vi "Condition _string_4_prod_count_YEAR_3.vi"(0 "Form Date":timestamp format="%<%Y-%m-%d>T", 1 "To Date":timestamp format="%<%Y-%m-%d>T", 3 "Shift":string(combo)="ALL", 4 "Select Station":string(combo)="ST 1", 5 "STACKHOLDER_ID":i32, 6 "Select Stakeholder":string(combo), 7 "Refnum out 2":T1, 9 "error in (no error)":errorcluster, 10 "Select Month":string(combo), 12 "Select Year":string(combo)) -> (11 "error out":errorcluster, 13 "Refnum out":T1, 14 "sum":i32[](array[numeric]), 15 "PROD COUNT TEST":string[](array[string]), 17 "Table":string[][](array[string]), 18 "Elements Found out":string[](array[string]), 19 "Array 3":string[][](array[string]))   [LabVIEW 2017]
uses:
  <vilib>/addons/database/Connection.llb/Conn ObjectReference.ctl
  <vilib>/addons/database/NI_Database_API.lvlib
panel:
  out "COUNT":string[](array[string])
  out "DATE":string[](array[string])
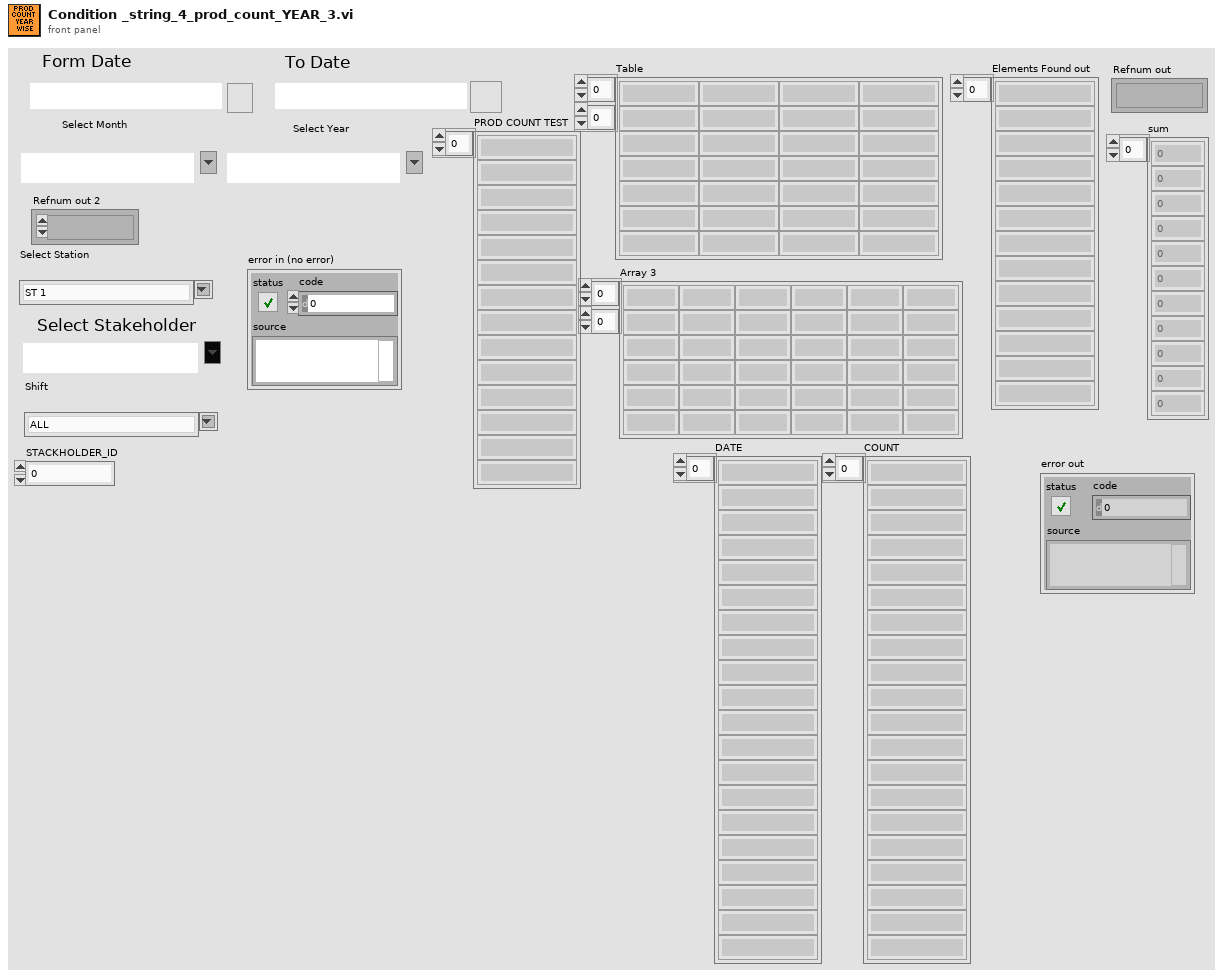
[diagram p1: front panel]
types:
  T1 = typedef "NI_Database_API.lvlib/Conn ObjectReference.ctl" = refnum<k1>
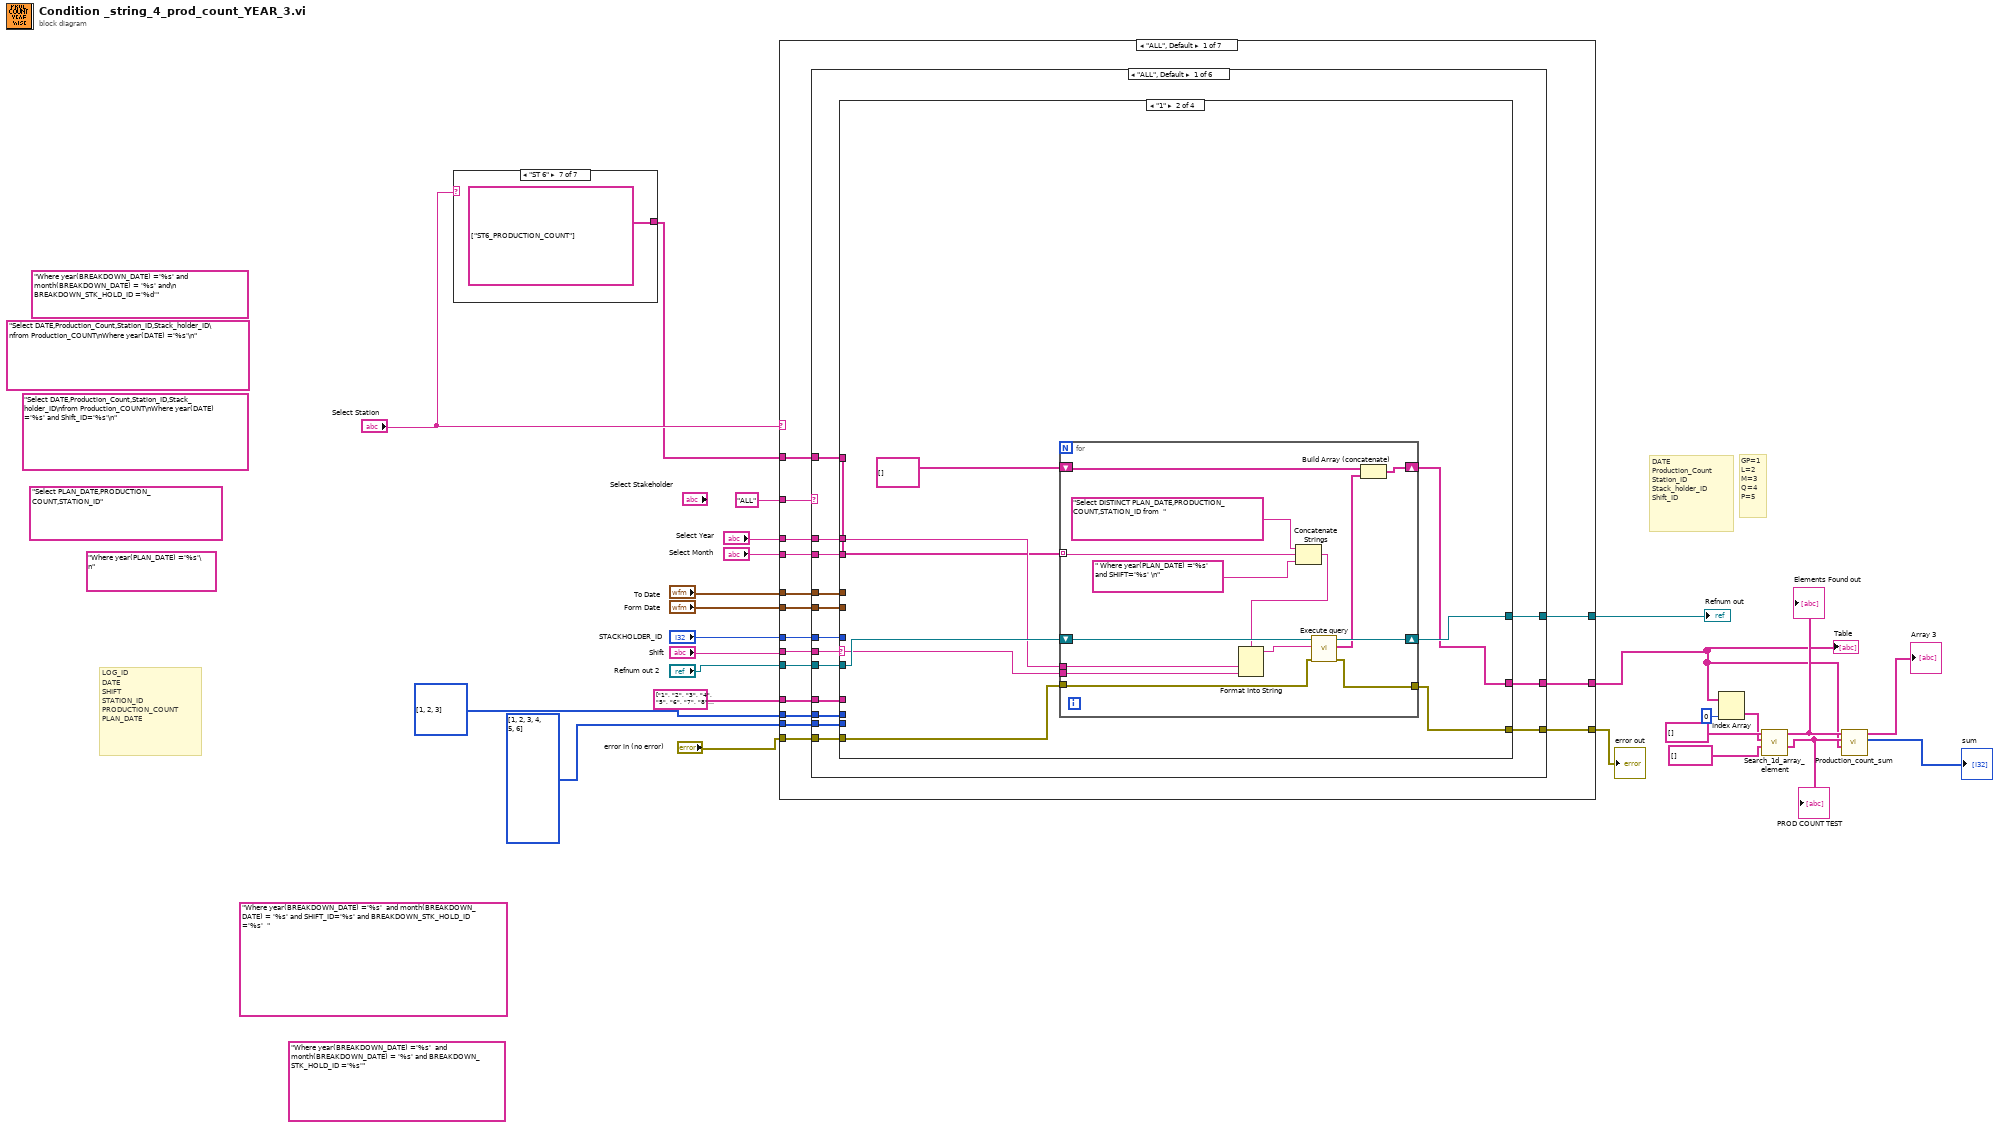
[diagram p0: block diagram]
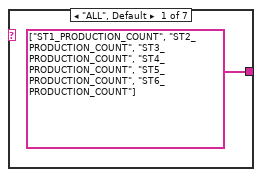
[diagram p2: hidden frame]
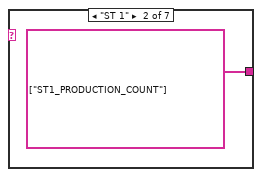
[diagram p3: hidden frame]
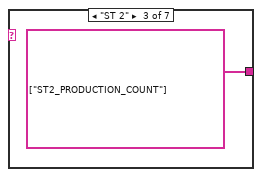
[diagram p4: hidden frame]
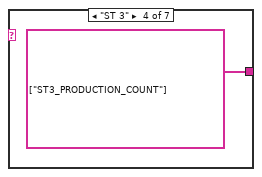
[diagram p5: hidden frame]
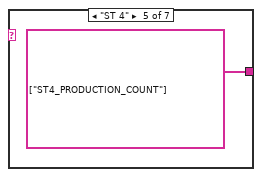
[diagram p6: hidden frame]
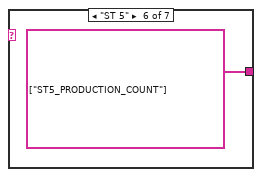
[diagram p7: hidden frame]
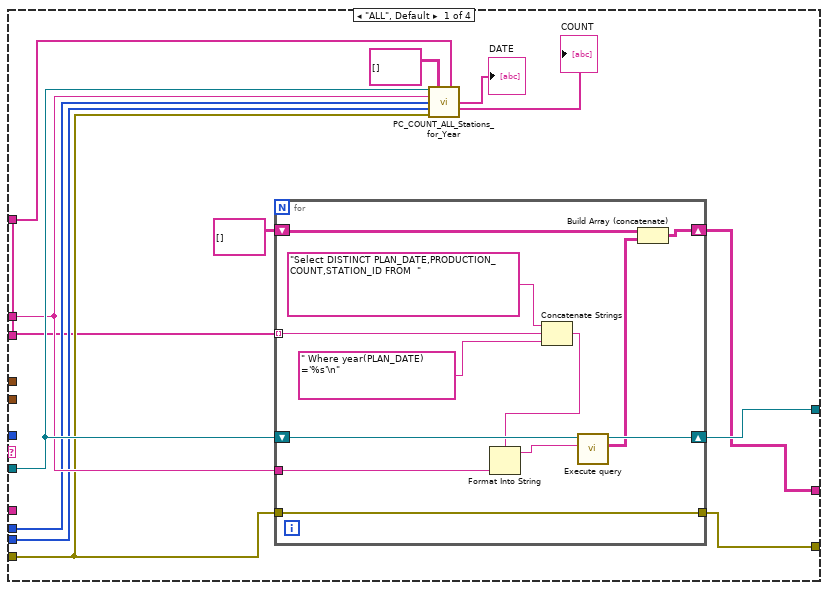
[diagram p8: hidden frame]
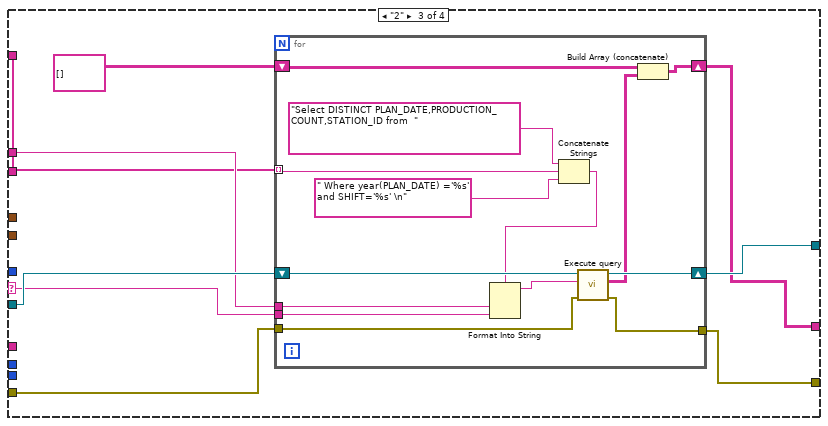
[diagram p9: hidden frame]
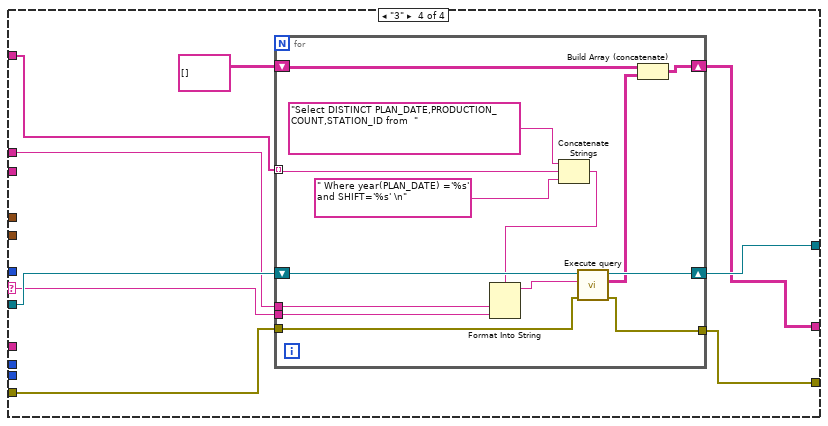
[diagram p10: hidden frame]
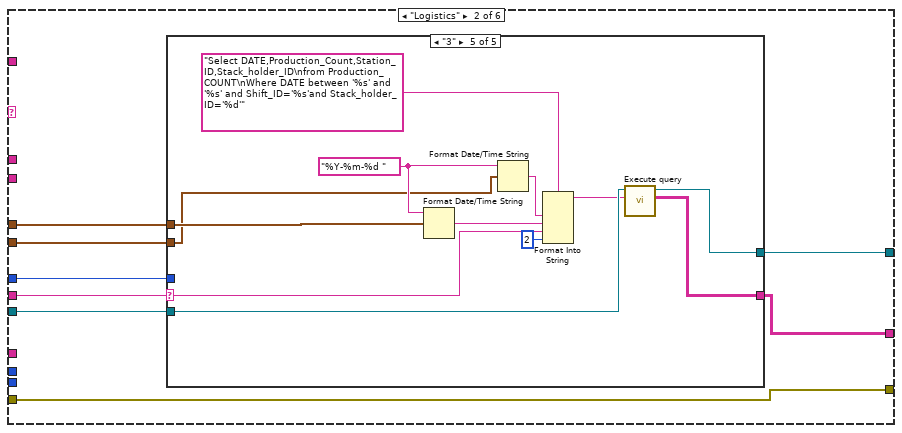
[diagram p11: hidden frame]
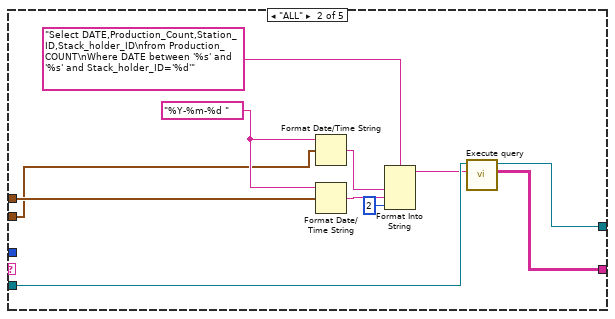
[diagram p13: hidden frame]
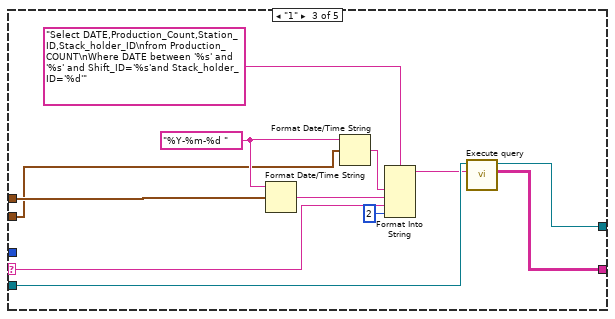
[diagram p14: hidden frame]
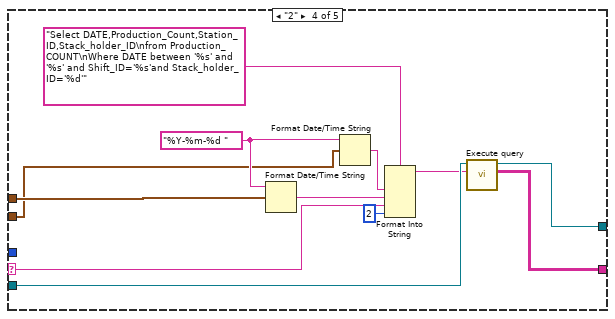
[diagram p15: hidden frame]
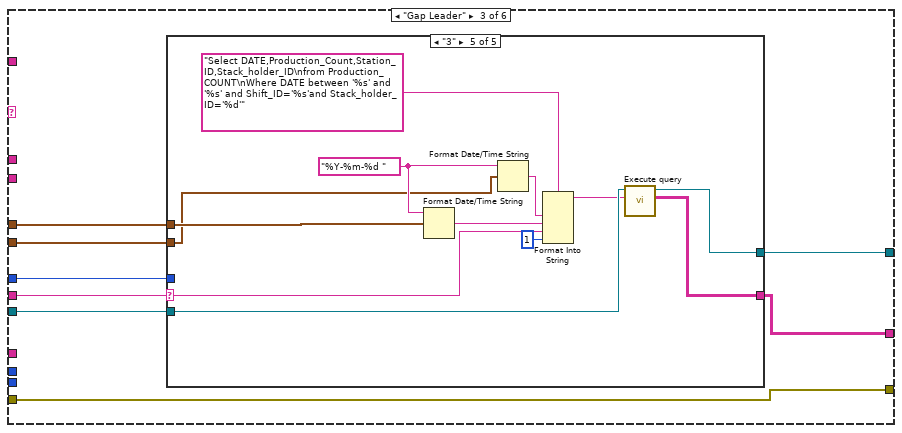
[diagram p16: hidden frame]
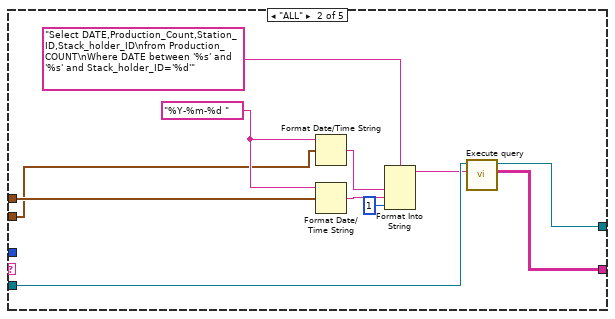
[diagram p18: hidden frame]
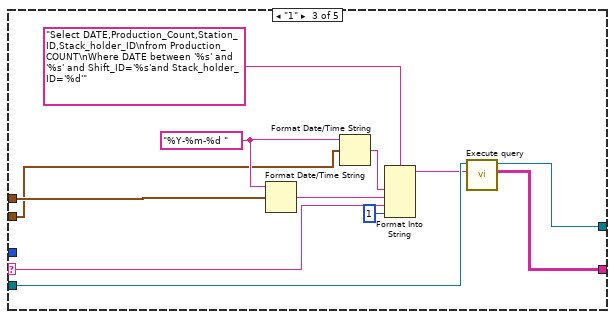
[diagram p19: hidden frame]
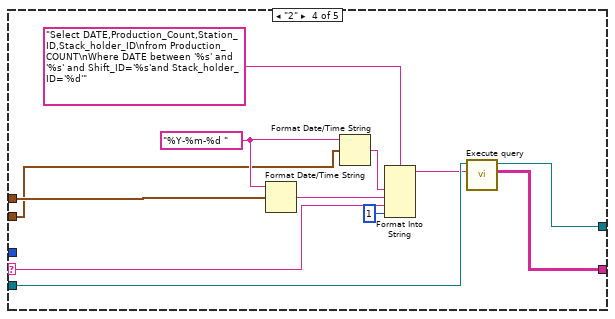
[diagram p20: hidden frame]
diagram:
  (unwired) "Where year(PLAN_DATE) ='%s'\n"
  (unwired) "Select PLAN_DATE,PRODUCTION_COUNT,STATION_ID"
  (unwired) "Select DATE,Production_Count,Station_ID,Stack_holder_ID\nfrom Production_COUNT\nWhere year(DATE) ='%s' and Shift_ID='%s'\n" ("string")
  (unwired) "Select DATE,Production_Count,Station_ID,Stack_holder_ID\nfrom Production_COUNT\nWhere year(DATE) ='%s'\n" ("string")
  (unwired) "Where year(BREAKDOWN_DATE) ='%s' and month(BREAKDOWN_DATE) = '%s' and\n BREAKDOWN_STK_HOLD_ID ='%d'" ("condition")
  (unwired) "Where year(BREAKDOWN_DATE) ='%s'  and month(BREAKDOWN_DATE) = '%s' and BREAKDOWN_STK_HOLD_ID ='%s'" ("condition")
  (unwired) "Where year(BREAKDOWN_DATE) ='%s'  and month(BREAKDOWN_DATE) = '%s' and SHIFT_ID='%s' and BREAKDOWN_STK_HOLD_ID ='%s'  " ("condition")
  # "LOG_ID\nDATE\nSHIFT\nSTATION_ID\nPRODUCTION_COUNT\nPLAN_DATE"
  # "GP=1\nL=2\nM=3\nQ=4\nP=5"
  # "DATE\nProduction_Count\nStation_ID\nStack_holder_ID\nShift_ID"
  n1 = case shown="\"ST 6\"" "Select Station" {
    tunnel: [string[] ["ST1_PRODUCTION_COUNT", "ST2_PRODUCTION_COUNT", "ST3_PRODUCTION_COUNT", "ST4_PRODUCTION_COUNT", "ST5_PRODUCTION_COUNT", "ST6_PRODUCTION_COUNT"] string[] ["ST1_PRODUCTION_COUNT"] string[] ["ST2_PRODUCTION_COUNT"] string[] ["ST3_PRODUCTION_COUNT"] string[] ["ST4_PRODUCTION_COUNT"] string[] ["ST5_PRODUCTION_COUNT"] string[] ["ST6_PRODUCTION_COUNT"]] -> w4
    frame "ALL", Default {
    }
    frame "ST 1" {
    }
    frame "ST 2" {
    }
    frame "ST 3" {
    }
    frame "ST 4" {
    }
    frame "ST 5" {
    }
    frame "ST 6" {
    }
  }
  n2 = case shown="\"ALL\", Default" "Select Station" {
    tunnel: "Shift" -> [w48 w450 w861 w1272 w1683 w2094 w2505]
    tunnel: "To Date" -> [w47 w449 w860 w1271 w1682 w2093 w2504]
    tunnel: "Form Date" -> [w46 w448 w859 w1270 w1681 w2092 w2503]
    tunnel: "STACKHOLDER_ID" -> [w45 w447 w858 w1269 w1680 w2091 w2502]
    tunnel: "Refnum out 2" -> [w44 w446 w857 w1268 w1679 w2090 w2501]
    tunnel: [w43 w445 w856 w1267 w1678 w2089 w2500] -> w20
    tunnel: "ALL" -> [w42 w444 w855 w1266 w1677 w2088 w2499]
    tunnel: i32[] [1, 2, 3, 4, 5, 6] -> [w41 _ _ _ _ _ _]
    tunnel: string[] ["1", "2", "3", "4", "5", "6", "7", "8", "9", "10", "11", "12"] -> [w40 _ _ _ _ _ _]
    tunnel: "Select Year" -> [w39 w443 w854 w1265 w1676 w2087 w2498]
    tunnel: "Select Month" -> [w38 w442 w853 w1264 w1675 w2086 w2497]
    tunnel: [w37 w441 w852 w1263 w1674 w2085 w2496] -> w7
    tunnel: w4 -> [w36 w440 w851 w1262 w1673 w2084 w2495]
    tunnel: "error in (no error)" -> [w35 w438 w849 w1260 w1671 w2082 w2493]
    tunnel: [w34 w439 w850 w1261 w1672 w2083 w2494] -> w2
    tunnel: i32[] [1, 2, 3] -> [w33 _ _ _ _ _ _]
    frame "ALL", Default {
      n3 = case shown="\"ALL\", Default" w42 {
        tunnel: w48 -> [w63 w165 w221 w277 w333 w389]
        tunnel: w47 -> [w62 w164 w220 w276 w332 w388]
        tunnel: w46 -> [w61 w163 w219 w275 w331 w387]
        tunnel: w45 -> [w60 w162 w218 w274 w330 w386]
        tunnel: w44 -> [w59 w161 w217 w273 w329 w385]
        tunnel: [w58 w160 w216 w272 w328 w384] -> w43
        tunnel: w41 -> [w57 _ _ _ _ _]
        tunnel: w40 -> [w56 _ _ _ _ _]
        tunnel: w39 -> [w55 _ _ _ _ _]
        tunnel: w38 -> [w54 _ _ _ _ _]
        tunnel: [w53 w158 w215 w270 w326 w382] -> w37
        tunnel: w36 -> [w52 _ _ _ _ _]
        tunnel: w35 -> [w51 w159 w214 w271 w327 w383]
        tunnel: [w50 w159 w214 w271 w327 w383] -> w34
        tunnel: w33 -> [w49 _ _ _ _ _]
        frame "ALL", Default {
          n4 = case shown="\"1\"" w63 {
            selector: w63 -> [_ w89 w112 w135]
            tunnel: w62 -> [_ _ _ _]
            tunnel: w61 -> [_ _ _ _]
            tunnel: w60 -> [_ _ _ _]
            tunnel: w59 -> [w72 w97 w120 w143]
            tunnel: [w76 w96 w119 w142] -> w58
            tunnel: w57 -> [w69 _ _ _]
            tunnel: w56 -> [_ _ _ _]
            tunnel: w55 -> [w71 w95 w118 w141]
            tunnel: w54 -> [_ _ _ _]
            tunnel: [w73 w90 w113 w136] -> w53
            tunnel: w52 -> [w66 w94 w117 w140]
            tunnel: w51 -> [w68 w92 w115 w138]
            tunnel: [w75 w93 w116 w139] -> w50
            tunnel: w49 -> [w70 _ _ _]
            frame "ALL", Default {
              n5 = for {
                tunnel: w71 -> [w86]
                shift-right: [w87] -> w76
                shift-left: w72 -> [w88]
                tunnel: w66 -> [w83] mode=indexing
                tunnel: [w80] -> w75
                tunnel: w68 -> [w80]
                shift-right: [w77] -> w73
                shift-left: string[][] [] ("Output Array") -> [w79]
                n6 = Concatenate Strings("Select DISTINCT PLAN_DATE,PRODUCTION_COUNT,STATION_ID FROM  ", w83, " Where year(PLAN_DATE) ='%s'\n") -> (w81:string)
                n7 = Format Into String(format string=w81, w86) -> (resulting string=w85:string)  [unwired: 2 in, 1 out]
                n8 = call "Execute query.vi"("String"=w85, "connection reference"=w88) -> ("Table"=w78:string[][], "connection reference 2"=w87:T1)  [unwired: 6 in, 2 out]
                n9 = Build Array (concatenate)(w79, w78) -> (w77:string[][])
              }
              n10 = call "PC_COUNT_ALL_Stations_for_Year.vi"("Refnum in"=w72, "data in"=string[][] [] ("Output Array"), "Array 3"=w66, "Select Year 2"=w71, "SHIFT"=w70, "STATION"=w69, "error in (no error)"=w68) -> ("DATE"=→"DATE":string[], "COUNT"=→"COUNT":string[])  [unwired: 4 in, 3 out]
            }
            frame "1" {
              n11 = for {
                tunnel: w95 -> [w109]
                shift-right: [w110] -> w96
                shift-left: w97 -> [w111]
                tunnel: w94 -> [w107] mode=indexing
                tunnel: [w100] -> w93
                tunnel: w92 -> [w101]
                shift-right: [w102] -> w90
                shift-left: string[][] [] ("Output Array") -> [w104]
                tunnel: w89 -> [w99]
                n12 = Concatenate Strings("Select DISTINCT PLAN_DATE,PRODUCTION_COUNT,STATION_ID from  ", w107, " Where year(PLAN_DATE) ='%s' and SHIFT='%s' \n") -> (w105:string)
                n13 = Format Into String(format string=w105, w109, w99) -> (resulting string=w108:string)  [unwired: 2 in, 1 out]
                n14 = call "Execute query.vi"("error in (no error)"=w101, "String"=w108, "connection reference"=w111) -> ("error out"=w100:errorcluster, "Table"=w103:string[][], "connection reference 2"=w110:T1)  [unwired: 5 in, 1 out]
                n15 = Build Array (concatenate)(w104, w103) -> (w102:string[][])
              }
            }
            frame "2" {
              n16 = for {
                tunnel: w118 -> [w132]
                shift-right: [w133] -> w119
                shift-left: w120 -> [w134]
                tunnel: w117 -> [w130] mode=indexing
                tunnel: [w123] -> w116
                tunnel: w115 -> [w124]
                shift-right: [w125] -> w113
                shift-left: string[][] [] ("Output Array") -> [w127]
                tunnel: w112 -> [w122]
                n17 = Concatenate Strings("Select DISTINCT PLAN_DATE,PRODUCTION_COUNT,STATION_ID from  ", w130, " Where year(PLAN_DATE) ='%s' and SHIFT='%s' \n") -> (w128:string)
                n18 = Format Into String(format string=w128, w132, w122) -> (resulting string=w131:string)  [unwired: 2 in, 1 out]
                n19 = call "Execute query.vi"("error in (no error)"=w124, "String"=w131, "connection reference"=w134) -> ("error out"=w123:errorcluster, "Table"=w126:string[][], "connection reference 2"=w133:T1)  [unwired: 5 in, 1 out]
                n20 = Build Array (concatenate)(w127, w126) -> (w125:string[][])
              }
            }
            frame "3" {
              n21 = for {
                tunnel: w141 -> [w155]
                shift-right: [w156] -> w142
                shift-left: w143 -> [w157]
                tunnel: w140 -> [w153] mode=indexing
                tunnel: [w146] -> w139
                tunnel: w138 -> [w147]
                shift-right: [w148] -> w136
                shift-left: string[][] [] ("Output Array") -> [w150]
                tunnel: w135 -> [w145]
                n22 = Concatenate Strings("Select DISTINCT PLAN_DATE,PRODUCTION_COUNT,STATION_ID from  ", w153, " Where year(PLAN_DATE) ='%s' and SHIFT='%s' \n") -> (w151:string)
                n23 = Format Into String(format string=w151, w155, w145) -> (resulting string=w154:string)  [unwired: 2 in, 1 out]
                n24 = call "Execute query.vi"("error in (no error)"=w147, "String"=w154, "connection reference"=w157) -> ("error out"=w146:errorcluster, "Table"=w149:string[][], "connection reference 2"=w156:T1)  [unwired: 5 in, 1 out]
                n25 = Build Array (concatenate)(w150, w149) -> (w148:string[][])
              }
            }
          }
        }
        frame "Logistics" {
          n26 = case shown="\"3\"" w165 {
            selector: w165 -> [_ _ w179 w191 w203]
            tunnel: w164 -> [_ w176 w188 w200 w212]
            tunnel: w163 -> [_ w175 w187 w199 w211]
            tunnel: w162 -> [_ _ _ _ _]
            tunnel: [_ w169 w181 w193 w205] -> w158
            tunnel: w161 -> [w166 w172 w184 w196 w208]
            tunnel: [w166 w168 w180 w192 w204] -> w160
            frame "False", Default {
            }
            frame "ALL" {
              w177 = "%Y-%m-%d " ("time format string (%c)")
              n27 = Format Date/Time String(time format string (%c)=w177, seconds (now)=w175) -> (date/time string=w174:string)  [unwired: 1 in]
              n28 = Format Date/Time String(time format string (%c)=w177, seconds (now)=w176) -> (date/time string=w173:string)  [unwired: 1 in]
              n29 = Format Into String(format string="Select DATE,Production_Count,Station_ID,Stack_holder_ID\nfrom Production_COUNT\nWhere DATE between '%s' and '%s' and Stack_holder_ID='%d'" ("string"), w174, w173, 2 ("input 3")) -> (resulting string=w170:string)  [unwired: 2 in, 1 out]
              n30 = call "Execute query.vi"("String"=w170, "connection reference"=w172) -> ("Table"=w169:string[][], "connection reference 2"=w168:T1)  [unwired: 6 in, 2 out]
            }
            frame "1" {
              w189 = "%Y-%m-%d " ("time format string (%c)")
              n31 = Format Date/Time String(time format string (%c)=w189, seconds (now)=w188) -> (date/time string=w185:string)  [unwired: 1 in]
              n32 = Format Date/Time String(time format string (%c)=w189, seconds (now)=w187) -> (date/time string=w186:string)  [unwired: 1 in]
              n33 = Format Into String(format string="Select DATE,Production_Count,Station_ID,Stack_holder_ID\nfrom Production_COUNT\nWhere DATE between '%s' and '%s' and Shift_ID='%s'and Stack_holder_ID='%d'" ("string"), w186, w185, w179, 2 ("input 4")) -> (resulting string=w182:string)  [unwired: 2 in, 1 out]
              n34 = call "Execute query.vi"("String"=w182, "connection reference"=w184) -> ("Table"=w181:string[][], "connection reference 2"=w180:T1)  [unwired: 6 in, 2 out]
            }
            frame "2" {
              w201 = "%Y-%m-%d " ("time format string (%c)")
              n35 = Format Date/Time String(time format string (%c)=w201, seconds (now)=w200) -> (date/time string=w197:string)  [unwired: 1 in]
              n36 = Format Date/Time String(time format string (%c)=w201, seconds (now)=w199) -> (date/time string=w198:string)  [unwired: 1 in]
              n37 = Format Into String(format string="Select DATE,Production_Count,Station_ID,Stack_holder_ID\nfrom Production_COUNT\nWhere DATE between '%s' and '%s' and Shift_ID='%s'and Stack_holder_ID='%d'" ("string"), w198, w197, w191, 2 ("input 4")) -> (resulting string=w194:string)  [unwired: 2 in, 1 out]
              n38 = call "Execute query.vi"("String"=w194, "connection reference"=w196) -> ("Table"=w193:string[][], "connection reference 2"=w192:T1)  [unwired: 6 in, 2 out]
            }
            frame "3" {
              w213 = "%Y-%m-%d " ("time format string (%c)")
              n39 = Format Date/Time String(time format string (%c)=w213, seconds (now)=w212) -> (date/time string=w209:string)  [unwired: 1 in]
              n40 = Format Date/Time String(time format string (%c)=w213, seconds (now)=w211) -> (date/time string=w210:string)  [unwired: 1 in]
              n41 = Format Into String(format string="Select DATE,Production_Count,Station_ID,Stack_holder_ID\nfrom Production_COUNT\nWhere DATE between '%s' and '%s' and Shift_ID='%s'and Stack_holder_ID='%d'" ("string"), w210, w209, w203, 2 ("input 4")) -> (resulting string=w206:string)  [unwired: 2 in, 1 out]
              n42 = call "Execute query.vi"("String"=w206, "connection reference"=w208) -> ("Table"=w205:string[][], "connection reference 2"=w204:T1)  [unwired: 6 in, 2 out]
            }
          }
        }
        frame "Gap Leader" {
          n43 = case shown="\"3\"" w221 {
            selector: w221 -> [_ _ w235 w247 w259]
            tunnel: w220 -> [_ w232 w244 w256 w268]
            tunnel: w219 -> [_ w231 w243 w255 w267]
            tunnel: w218 -> [_ _ _ _ _]
            tunnel: [_ w225 w237 w249 w261] -> w215
            tunnel: w217 -> [w222 w228 w240 w252 w264]
            tunnel: [w222 w224 w236 w248 w260] -> w216
            frame "False", Default {
            }
            frame "ALL" {
              w233 = "%Y-%m-%d " ("time format string (%c)")
              n44 = Format Date/Time String(time format string (%c)=w233, seconds (now)=w231) -> (date/time string=w230:string)  [unwired: 1 in]
              n45 = Format Date/Time String(time format string (%c)=w233, seconds (now)=w232) -> (date/time string=w229:string)  [unwired: 1 in]
              n46 = Format Into String(format string="Select DATE,Production_Count,Station_ID,Stack_holder_ID\nfrom Production_COUNT\nWhere DATE between '%s' and '%s' and Stack_holder_ID='%d'" ("string"), w230, w229, 1 ("input 3")) -> (resulting string=w226:string)  [unwired: 2 in, 1 out]
              n47 = call "Execute query.vi"("String"=w226, "connection reference"=w228) -> ("Table"=w225:string[][], "connection reference 2"=w224:T1)  [unwired: 6 in, 2 out]
            }
            frame "1" {
              w245 = "%Y-%m-%d " ("time format string (%c)")
              n48 = Format Date/Time String(time format string (%c)=w245, seconds (now)=w244) -> (date/time string=w241:string)  [unwired: 1 in]
              n49 = Format Date/Time String(time format string (%c)=w245, seconds (now)=w243) -> (date/time string=w242:string)  [unwired: 1 in]
              n50 = Format Into String(format string="Select DATE,Production_Count,Station_ID,Stack_holder_ID\nfrom Production_COUNT\nWhere DATE between '%s' and '%s' and Shift_ID='%s'and Stack_holder_ID='%d'" ("string"), w242, w241, w235, 1 ("input 4")) -> (resulting string=w238:string)  [unwired: 2 in, 1 out]
              n51 = call "Execute query.vi"("String"=w238, "connection reference"=w240) -> ("Table"=w237:string[][], "connection reference 2"=w236:T1)  [unwired: 6 in, 2 out]
            }
            frame "2" {
              w257 = "%Y-%m-%d " ("time format string (%c)")
              n52 = Format Date/Time String(time format string (%c)=w257, seconds (now)=w256) -> (date/time string=w253:string)  [unwired: 1 in]
              n53 = Format Date/Time String(time format string (%c)=w257, seconds (now)=w255) -> (date/time string=w254:string)  [unwired: 1 in]
              n54 = Format Into String(format string="Select DATE,Production_Count,Station_ID,Stack_holder_ID\nfrom Production_COUNT\nWhere DATE between '%s' and '%s' and Shift_ID='%s'and Stack_holder_ID='%d'" ("string"), w254, w253, w247, 1 ("input 4")) -> (resulting string=w250:string)  [unwired: 2 in, 1 out]
              n55 = call "Execute query.vi"("String"=w250, "connection reference"=w252) -> ("Table"=w249:string[][], "connection reference 2"=w248:T1)  [unwired: 6 in, 2 out]
            }
            frame "3" {
              w269 = "%Y-%m-%d " ("time format string (%c)")
              n56 = Format Date/Time String(time format string (%c)=w269, seconds (now)=w268) -> (date/time string=w265:string)  [unwired: 1 in]
              n57 = Format Date/Time String(time format string (%c)=w269, seconds (now)=w267) -> (date/time string=w266:string)  [unwired: 1 in]
              n58 = Format Into String(format string="Select DATE,Production_Count,Station_ID,Stack_holder_ID\nfrom Production_COUNT\nWhere DATE between '%s' and '%s' and Shift_ID='%s'and Stack_holder_ID='%d'" ("string"), w266, w265, w259, 1 ("input 4")) -> (resulting string=w262:string)  [unwired: 2 in, 1 out]
              n59 = call "Execute query.vi"("String"=w262, "connection reference"=w264) -> ("Table"=w261:string[][], "connection reference 2"=w260:T1)  [unwired: 6 in, 2 out]
            }
          }
        }
        frame "Maintenance" {
          n60 = case shown="\"ALL\"" w277 {
            selector: w277 -> [_ _ w291 w303 w315]
            tunnel: w276 -> [_ w288 w300 w312 w324]
            tunnel: w275 -> [_ w287 w299 w311 w323]
            tunnel: w274 -> [_ _ _ _ _]
            tunnel: [_ w281 w293 w305 w317] -> w270
            tunnel: w273 -> [w278 w284 w296 w308 w320]
            tunnel: [w278 w280 w292 w304 w316] -> w272
            frame "False", Default {
            }
            frame "ALL" {
              w289 = "%Y-%m-%d " ("time format string (%c)")
              n61 = Format Date/Time String(time format string (%c)=w289, seconds (now)=w287) -> (date/time string=w286:string)  [unwired: 1 in]
              n62 = Format Date/Time String(time format string (%c)=w289, seconds (now)=w288) -> (date/time string=w285:string)  [unwired: 1 in]
              n63 = Format Into String(format string="Select DATE,Production_Count,Station_ID,Stack_holder_ID\nfrom Production_COUNT\nWhere DATE between '%s' and '%s' and Stack_holder_ID='%d'" ("string"), w286, w285, 3 ("input 3")) -> (resulting string=w282:string)  [unwired: 2 in, 1 out]
              n64 = call "Execute query.vi"("String"=w282, "connection reference"=w284) -> ("Table"=w281:string[][], "connection reference 2"=w280:T1)  [unwired: 6 in, 2 out]
            }
            frame "1" {
              w301 = "%Y-%m-%d " ("time format string (%c)")
              n65 = Format Date/Time String(time format string (%c)=w301, seconds (now)=w300) -> (date/time string=w297:string)  [unwired: 1 in]
              n66 = Format Date/Time String(time format string (%c)=w301, seconds (now)=w299) -> (date/time string=w298:string)  [unwired: 1 in]
              n67 = Format Into String(format string="Select DATE,Production_Count,Station_ID,Stack_holder_ID\nfrom Production_COUNT\nWhere DATE between '%s' and '%s' and Shift_ID='%s'and Stack_holder_ID='%d'" ("string"), w298, w297, w291, 3 ("input 4")) -> (resulting string=w294:string)  [unwired: 2 in, 1 out]
              n68 = call "Execute query.vi"("String"=w294, "connection reference"=w296) -> ("Table"=w293:string[][], "connection reference 2"=w292:T1)  [unwired: 6 in, 2 out]
            }
            frame "2" {
              w313 = "%Y-%m-%d " ("time format string (%c)")
              n69 = Format Date/Time String(time format string (%c)=w313, seconds (now)=w312) -> (date/time string=w309:string)  [unwired: 1 in]
              n70 = Format Date/Time String(time format string (%c)=w313, seconds (now)=w311) -> (date/time string=w310:string)  [unwired: 1 in]
              n71 = Format Into String(format string="Select DATE,Production_Count,Station_ID,Stack_holder_ID\nfrom Production_COUNT\nWhere DATE between '%s' and '%s' and Shift_ID='%s'and Stack_holder_ID='%d'" ("string"), w310, w309, w303, 3 ("input 4")) -> (resulting string=w306:string)  [unwired: 2 in, 1 out]
              n72 = call "Execute query.vi"("String"=w306, "connection reference"=w308) -> ("Table"=w305:string[][], "connection reference 2"=w304:T1)  [unwired: 6 in, 2 out]
            }
            frame "3" {
              w325 = "%Y-%m-%d " ("time format string (%c)")
              n73 = Format Date/Time String(time format string (%c)=w325, seconds (now)=w324) -> (date/time string=w321:string)  [unwired: 1 in]
              n74 = Format Date/Time String(time format string (%c)=w325, seconds (now)=w323) -> (date/time string=w322:string)  [unwired: 1 in]
              n75 = Format Into String(format string="Select DATE,Production_Count,Station_ID,Stack_holder_ID\nfrom Production_COUNT\nWhere DATE between '%s' and '%s' and Shift_ID='%s'and Stack_holder_ID='%d'" ("string"), w322, w321, w315, 3 ("input 4")) -> (resulting string=w318:string)  [unwired: 2 in, 1 out]
              n76 = call "Execute query.vi"("String"=w318, "connection reference"=w320) -> ("Table"=w317:string[][], "connection reference 2"=w316:T1)  [unwired: 6 in, 2 out]
            }
          }
        }
        frame "Quality" {
          n77 = case shown="\"3\"" w333 {
            selector: w333 -> [_ _ w347 w359 w371]
            tunnel: w332 -> [_ w344 w356 w368 w380]
            tunnel: w331 -> [_ w343 w355 w367 w379]
            tunnel: w330 -> [_ _ _ _ _]
            tunnel: [_ w337 w349 w361 w373] -> w326
            tunnel: w329 -> [w334 w340 w352 w364 w376]
            tunnel: [w334 w336 w348 w360 w372] -> w328
            frame "False", Default {
            }
            frame "ALL" {
              w345 = "%Y-%m-%d " ("time format string (%c)")
              n78 = Format Date/Time String(time format string (%c)=w345, seconds (now)=w343) -> (date/time string=w342:string)  [unwired: 1 in]
              n79 = Format Date/Time String(time format string (%c)=w345, seconds (now)=w344) -> (date/time string=w341:string)  [unwired: 1 in]
              n80 = Format Into String(format string="Select DATE,Production_Count,Station_ID,Stack_holder_ID\nfrom Production_COUNT\nWhere DATE between '%s' and '%s' and Stack_holder_ID='%d'" ("string"), w342, w341, 4 ("input 3")) -> (resulting string=w338:string)  [unwired: 2 in, 1 out]
              n81 = call "Execute query.vi"("String"=w338, "connection reference"=w340) -> ("Table"=w337:string[][], "connection reference 2"=w336:T1)  [unwired: 6 in, 2 out]
            }
            frame "1" {
              w357 = "%Y-%m-%d " ("time format string (%c)")
              n82 = Format Date/Time String(time format string (%c)=w357, seconds (now)=w356) -> (date/time string=w353:string)  [unwired: 1 in]
              n83 = Format Date/Time String(time format string (%c)=w357, seconds (now)=w355) -> (date/time string=w354:string)  [unwired: 1 in]
              n84 = Format Into String(format string="Select DATE,Production_Count,Station_ID,Stack_holder_ID\nfrom Production_COUNT\nWhere DATE between '%s' and '%s' and Shift_ID='%s'and Stack_holder_ID='%d'" ("string"), w354, w353, w347, 4 ("input 4")) -> (resulting string=w350:string)  [unwired: 2 in, 1 out]
              n85 = call "Execute query.vi"("String"=w350, "connection reference"=w352) -> ("Table"=w349:string[][], "connection reference 2"=w348:T1)  [unwired: 6 in, 2 out]
            }
            frame "2" {
              w369 = "%Y-%m-%d " ("time format string (%c)")
              n86 = Format Date/Time String(time format string (%c)=w369, seconds (now)=w368) -> (date/time string=w365:string)  [unwired: 1 in]
              n87 = Format Date/Time String(time format string (%c)=w369, seconds (now)=w367) -> (date/time string=w366:string)  [unwired: 1 in]
              n88 = Format Into String(format string="Select DATE,Production_Count,Station_ID,Stack_holder_ID\nfrom Production_COUNT\nWhere DATE between '%s' and '%s' and Shift_ID='%s'and Stack_holder_ID='%d'" ("string"), w366, w365, w359, 4 ("input 4")) -> (resulting string=w362:string)  [unwired: 2 in, 1 out]
              n89 = call "Execute query.vi"("String"=w362, "connection reference"=w364) -> ("Table"=w361:string[][], "connection reference 2"=w360:T1)  [unwired: 6 in, 2 out]
            }
            frame "3" {
              w381 = "%Y-%m-%d " ("time format string (%c)")
              n90 = Format Date/Time String(time format string (%c)=w381, seconds (now)=w380) -> (date/time string=w377:string)  [unwired: 1 in]
              n91 = Format Date/Time String(time format string (%c)=w381, seconds (now)=w379) -> (date/time string=w378:string)  [unwired: 1 in]
              n92 = Format Into String(format string="Select DATE,Production_Count,Station_ID,Stack_holder_ID\nfrom Production_COUNT\nWhere DATE between '%s' and '%s' and Shift_ID='%s'and Stack_holder_ID='%d'" ("string"), w378, w377, w371, 4 ("input 4")) -> (resulting string=w374:string)  [unwired: 2 in, 1 out]
              n93 = call "Execute query.vi"("String"=w374, "connection reference"=w376) -> ("Table"=w373:string[][], "connection reference 2"=w372:T1)  [unwired: 6 in, 2 out]
            }
          }
        }
        frame "Production" {
          n94 = case shown="\"3\"" w389 {
            selector: w389 -> [_ _ w403 w415 w427]
            tunnel: w388 -> [_ w400 w412 w424 w436]
            tunnel: w387 -> [_ w399 w411 w423 w435]
            tunnel: w386 -> [_ _ _ _ _]
            tunnel: [_ w393 w405 w417 w429] -> w382
            tunnel: w385 -> [w390 w396 w408 w420 w432]
            tunnel: [w390 w392 w404 w416 w428] -> w384
            frame "False", Default {
            }
            frame "ALL" {
              w401 = "%Y-%m-%d " ("time format string (%c)")
              n95 = Format Date/Time String(time format string (%c)=w401, seconds (now)=w399) -> (date/time string=w398:string)  [unwired: 1 in]
              n96 = Format Date/Time String(time format string (%c)=w401, seconds (now)=w400) -> (date/time string=w397:string)  [unwired: 1 in]
              n97 = Format Into String(format string="Select DATE,Production_Count,Station_ID,Stack_holder_ID\nfrom Production_COUNT\nWhere DATE between '%s' and '%s' and Stack_holder_ID='%d'" ("string"), w398, w397, 5 ("input 3")) -> (resulting string=w394:string)  [unwired: 2 in, 1 out]
              n98 = call "Execute query.vi"("String"=w394, "connection reference"=w396) -> ("Table"=w393:string[][], "connection reference 2"=w392:T1)  [unwired: 6 in, 2 out]
            }
            frame "1" {
              w413 = "%Y-%m-%d " ("time format string (%c)")
              n99 = Format Date/Time String(time format string (%c)=w413, seconds (now)=w412) -> (date/time string=w409:string)  [unwired: 1 in]
              n100 = Format Date/Time String(time format string (%c)=w413, seconds (now)=w411) -> (date/time string=w410:string)  [unwired: 1 in]
              n101 = Format Into String(format string="Select DATE,Production_Count,Station_ID,Stack_holder_ID\nfrom Production_COUNT\nWhere DATE between '%s' and '%s' and Shift_ID='%s'and Stack_holder_ID='%d'" ("string"), w410, w409, w403, 5 ("input 4")) -> (resulting string=w406:string)  [unwired: 2 in, 1 out]
              n102 = call "Execute query.vi"("String"=w406, "connection reference"=w408) -> ("Table"=w405:string[][], "connection reference 2"=w404:T1)  [unwired: 6 in, 2 out]
            }
            frame "2" {
              w425 = "%Y-%m-%d " ("time format string (%c)")
              n103 = Format Date/Time String(time format string (%c)=w425, seconds (now)=w424) -> (date/time string=w421:string)  [unwired: 1 in]
              n104 = Format Date/Time String(time format string (%c)=w425, seconds (now)=w423) -> (date/time string=w422:string)  [unwired: 1 in]
              n105 = Format Into String(format string="Select DATE,Production_Count,Station_ID,Stack_holder_ID\nfrom Production_COUNT\nWhere DATE between '%s' and '%s' and Shift_ID='%s'and Stack_holder_ID='%d'" ("string"), w422, w421, w415, 5 ("input 4")) -> (resulting string=w418:string)  [unwired: 2 in, 1 out]
              n106 = call "Execute query.vi"("String"=w418, "connection reference"=w420) -> ("Table"=w417:string[][], "connection reference 2"=w416:T1)  [unwired: 6 in, 2 out]
            }
            frame "3" {
              w437 = "%Y-%m-%d " ("time format string (%c)")
              n107 = Format Date/Time String(time format string (%c)=w437, seconds (now)=w436) -> (date/time string=w433:string)  [unwired: 1 in]
              n108 = Format Date/Time String(time format string (%c)=w437, seconds (now)=w435) -> (date/time string=w434:string)  [unwired: 1 in]
              n109 = Format Into String(format string="Select DATE,Production_Count,Station_ID,Stack_holder_ID\nfrom Production_COUNT\nWhere DATE between '%s' and '%s' and Shift_ID='%s'and Stack_holder_ID='%d'" ("string"), w434, w433, w427, 5 ("input 4")) -> (resulting string=w430:string)  [unwired: 2 in, 1 out]
              n110 = call "Execute query.vi"("String"=w430, "connection reference"=w432) -> ("Table"=w429:string[][], "connection reference 2"=w428:T1)  [unwired: 6 in, 2 out]
            }
          }
        }
      }
    }
    frame "ST 1" {
      n111 = case shown="\"ALL\", Default" w444 {
        tunnel: w450 -> [w462 w563 w622 w678 w737 w796]
        tunnel: w449 -> [w461 w562 w621 w677 w736 w795]
        tunnel: w448 -> [w460 w561 w620 w676 w735 w794]
        tunnel: w447 -> [w459 w560 w619 w675 w734 w793]
        tunnel: [w458 w559 w618 w674 w733 w792] -> w441
        tunnel: w446 -> [w457 w558 w617 w673 w732 w791]
        tunnel: [w456 w557 w616 w672 w731 w790] -> w445
        tunnel: w443 -> [w455 _ _ _ _ _]
        tunnel: w442 -> [w454 _ _ _ _ _]
        tunnel: w440 -> [w453 _ _ _ _ _]
        tunnel: [w452 _ _ _ _ _] -> w439
        tunnel: w438 -> [w451 _ _ _ _ _]
        frame "ALL", Default {
          n112 = case shown="\"ALL\", Default" w462 {
            selector: w462 -> [_ w487 w511 w535]
            tunnel: w461 -> [_ _ _ _]
            tunnel: w460 -> [_ _ _ _]
            tunnel: w459 -> [_ _ _ _]
            tunnel: [w465 w488 w512 w536] -> w458
            tunnel: w457 -> [w470 w493 w517 w541]
            tunnel: [w469 w492 w516 w540] -> w456
            tunnel: w455 -> [w468 w491 w515 w539]
            tunnel: w454 -> [_ _ _ _]
            tunnel: w453 -> [w467 w490 w514 w538]
            tunnel: [w464 w486 w510 w534] -> w452
            tunnel: w451 -> [w463 w485 w509 w533]
            frame "ALL", Default {
              n113 = for {
                tunnel: w468 -> [w480]
                shift-right: [w482] -> w469
                shift-left: w470 -> [w484]
                tunnel: w467 -> [w476] mode=indexing
                shift-right: [w473] -> w465
                shift-left: string[][] [] -> [w475]
                tunnel: [w471] -> w464
                tunnel: w463 -> [w472]
                n114 = Concatenate Strings("Select DISTINCT PLAN_DATE,PRODUCTION_COUNT,STATION_ID from  ", w476, " Where year(PLAN_DATE) ='%s' and STATION_ID='%d'\n") -> (w477:string)
                n115 = Format Into String(format string=w477, w480, 1 ("input 3")) -> (resulting string=w483:string)  [unwired: 2 in, 1 out]
                n116 = call "Execute query.vi"("error in (no error)"=w472, "String"=w483, "connection reference"=w484) -> ("error out"=w471:errorcluster, "Table"=w474:string[][], "connection reference 2"=w482:T1)  [unwired: 5 in, 1 out]
                n117 = Build Array (concatenate)(w475, w474) -> (w473:string[][])
              }
            }
            frame "1" {
              n118 = for {
                tunnel: w491 -> [w504]
                shift-right: [w506] -> w492
                shift-left: w493 -> [w508]
                tunnel: w490 -> [w500] mode=indexing
                shift-right: [w497] -> w488
                shift-left: string[][] [] -> [w499]
                tunnel: w487 -> [w496]
                tunnel: [w494] -> w486
                tunnel: w485 -> [w495]
                n119 = Concatenate Strings("Select DISTINCT PLAN_DATE,PRODUCTION_COUNT,STATION_ID from  ", w500, " Where year(PLAN_DATE) ='%s' and STATION_ID='%d' and  SHIFT='%s'\n") -> (w501:string)
                n120 = Format Into String(format string=w501, w504, 1 ("input 3"), w496) -> (resulting string=w507:string)  [unwired: 2 in, 1 out]
                n121 = call "Execute query.vi"("error in (no error)"=w495, "String"=w507, "connection reference"=w508) -> ("error out"=w494:errorcluster, "Table"=w498:string[][], "connection reference 2"=w506:T1)  [unwired: 5 in, 1 out]
                n122 = Build Array (concatenate)(w499, w498) -> (w497:string[][])
              }
            }
            frame "2" {
              n123 = for {
                tunnel: w515 -> [w528]
                shift-right: [w530] -> w516
                shift-left: w517 -> [w532]
                tunnel: w514 -> [w524] mode=indexing
                shift-right: [w521] -> w512
                shift-left: string[][] [] -> [w523]
                tunnel: w511 -> [w520]
                tunnel: [w518] -> w510
                tunnel: w509 -> [w519]
                n124 = Concatenate Strings("Select DISTINCT PLAN_DATE,PRODUCTION_COUNT,STATION_ID from  ", w524, " Where year(PLAN_DATE) ='%s' and STATION_ID='%d' and SHIFT='%s'\n") -> (w525:string)
                n125 = Format Into String(format string=w525, w528, 1 ("input 3"), w520) -> (resulting string=w531:string)  [unwired: 2 in, 1 out]
                n126 = call "Execute query.vi"("error in (no error)"=w519, "String"=w531, "connection reference"=w532) -> ("error out"=w518:errorcluster, "Table"=w522:string[][], "connection reference 2"=w530:T1)  [unwired: 5 in, 1 out]
                n127 = Build Array (concatenate)(w523, w522) -> (w521:string[][])
              }
            }
            frame "3" {
              n128 = for {
                tunnel: w539 -> [w552]
                shift-right: [w554] -> w540
                shift-left: w541 -> [w556]
                tunnel: w538 -> [w548] mode=indexing
                shift-right: [w545] -> w536
                shift-left: string[][] [] -> [w547]
                tunnel: w535 -> [w544]
                tunnel: [w542] -> w534
                tunnel: w533 -> [w543]
                n129 = Concatenate Strings("Select DISTINCT PLAN_DATE,PRODUCTION_COUNT,STATION_ID from  ", w548, " Where year(PLAN_DATE) ='%s' and STATION_ID='%d' and  SHIFT='%s'\n") -> (w549:string)
                n130 = Format Into String(format string=w549, w552, 1 ("input 3"), w544) -> (resulting string=w555:string)  [unwired: 2 in, 1 out]
                n131 = call "Execute query.vi"("error in (no error)"=w543, "String"=w555, "connection reference"=w556) -> ("error out"=w542:errorcluster, "Table"=w546:string[][], "connection reference 2"=w554:T1)  [unwired: 5 in, 1 out]
                n132 = Build Array (concatenate)(w547, w546) -> (w545:string[][])
              }
            }
          }
        }
        frame "Logistics" {
          n133 = case shown="\"ALL\"" w563 {
            selector: w563 -> [_ _ w579 w592 w605]
            tunnel: w562 -> [_ w575 w588 w601 w614]
            tunnel: w561 -> [_ w574 w587 w600 w613]
            tunnel: w560 -> [_ _ _ _ _]
            tunnel: [_ w568 w581 w594 w607] -> w559
            tunnel: w558 -> [w564 w571 w584 w597 w610]
            tunnel: [w564 w567 w580 w593 w606] -> w557
            frame "False", Default {
            }
            frame "ALL" {
              w576 = "%Y-%m-%d " ("time format string (%c)")
              n134 = Format Date/Time String(time format string (%c)=w576, seconds (now)=w574) -> (date/time string=w573:string)  [unwired: 1 in]
              n135 = Format Date/Time String(time format string (%c)=w576, seconds (now)=w575) -> (date/time string=w572:string)  [unwired: 1 in]
              n136 = Format Into String(format string="Select DATE,Production_Count,Station_ID,Stack_holder_ID\nfrom Production_COUNT\nWhere DATE between '%s' and '%s' and Stack_holder_ID='%d'\nand Station_ID='%d'" ("string"), w573, w572, 2 ("input 3"), 1 ("input 4")) -> (resulting string=w569:string)  [unwired: 2 in, 1 out]
              n137 = call "Execute query.vi"("String"=w569, "connection reference"=w571) -> ("Table"=w568:string[][], "connection reference 2"=w567:T1)  [unwired: 6 in, 2 out]
            }
            frame "1" {
              w589 = "%Y-%m-%d " ("time format string (%c)")
              n138 = Format Date/Time String(time format string (%c)=w589, seconds (now)=w588) -> (date/time string=w585:string)  [unwired: 1 in]
              n139 = Format Date/Time String(time format string (%c)=w589, seconds (now)=w587) -> (date/time string=w586:string)  [unwired: 1 in]
              n140 = Format Into String(format string="Select DATE,Production_Count,Station_ID,Stack_holder_ID\nfrom Production_COUNT\nWhere DATE between '%s' and '%s' and Shift_ID='%s'and Stack_holder_ID='%d'\nand Station_ID='%d'" ("string"), w586, w585, w579, 2 ("input 4"), 1 ("input 4")) -> (resulting string=w582:string)  [unwired: 2 in, 1 out]
              n141 = call "Execute query.vi"("String"=w582, "connection reference"=w584) -> ("Table"=w581:string[][], "connection reference 2"=w580:T1)  [unwired: 6 in, 2 out]
            }
            frame "2" {
              w602 = "%Y-%m-%d " ("time format string (%c)")
              n142 = Format Date/Time String(time format string (%c)=w602, seconds (now)=w601) -> (date/time string=w598:string)  [unwired: 1 in]
              n143 = Format Date/Time String(time format string (%c)=w602, seconds (now)=w600) -> (date/time string=w599:string)  [unwired: 1 in]
              n144 = Format Into String(format string="Select DATE,Production_Count,Station_ID,Stack_holder_ID\nfrom Production_COUNT\nWhere DATE between '%s' and '%s' and Shift_ID='%s'and Stack_holder_ID='%d'\nand Station_ID='%d'" ("string"), w599, w598, w592, 2 ("input 4"), 1 ("input 4")) -> (resulting string=w595:string)  [unwired: 2 in, 1 out]
              n145 = call "Execute query.vi"("String"=w595, "connection reference"=w597) -> ("Table"=w594:string[][], "connection reference 2"=w593:T1)  [unwired: 6 in, 2 out]
            }
            frame "3" {
              w615 = "%Y-%m-%d " ("time format string (%c)")
              n146 = Format Date/Time String(time format string (%c)=w615, seconds (now)=w614) -> (date/time string=w611:string)  [unwired: 1 in]
              n147 = Format Date/Time String(time format string (%c)=w615, seconds (now)=w613) -> (date/time string=w612:string)  [unwired: 1 in]
              n148 = Format Into String(format string="Select DATE,Production_Count,Station_ID,Stack_holder_ID\nfrom Production_COUNT\nWhere DATE between '%s' and '%s' and Shift_ID='%s'and Stack_holder_ID='%d'\nand Station_ID='%d'" ("string"), w612, w611, w605, 2 ("input 4"), 1 ("input 4")) -> (resulting string=w608:string)  [unwired: 2 in, 1 out]
              n149 = call "Execute query.vi"("String"=w608, "connection reference"=w610) -> ("Table"=w607:string[][], "connection reference 2"=w606:T1)  [unwired: 6 in, 2 out]
            }
          }
        }
        frame "Gap Leader" {
          n150 = case shown="\"3\"" w622 {
            selector: w622 -> [_ _ w637 w649 w661]
            tunnel: w621 -> [_ w634 w646 w658 w670]
            tunnel: w620 -> [_ w633 w645 w657 w669]
            tunnel: w619 -> [_ _ _ _ _]
            tunnel: [_ w627 w639 w651 w663] -> w618
            tunnel: w617 -> [w623 w630 w642 w654 w666]
            tunnel: [w623 w626 w638 w650 w662] -> w616
            frame "False", Default {
            }
            frame "ALL" {
              w635 = "%Y-%m-%d " ("time format string (%c)")
              n151 = Format Date/Time String(time format string (%c)=w635, seconds (now)=w633) -> (date/time string=w632:string)  [unwired: 1 in]
              n152 = Format Date/Time String(time format string (%c)=w635, seconds (now)=w634) -> (date/time string=w631:string)  [unwired: 1 in]
              n153 = Format Into String(format string="Select DATE,Production_Count,Station_ID,Stack_holder_ID\nfrom Production_COUNT\nWhere DATE between '%s' and '%s' and Stack_holder_ID='%d'\nand Station_ID='%d'" ("string"), w632, w631, 1 ("input 3"), 1 ("input 3")) -> (resulting string=w628:string)  [unwired: 2 in, 1 out]
              n154 = call "Execute query.vi"("String"=w628, "connection reference"=w630) -> ("Table"=w627:string[][], "connection reference 2"=w626:T1)  [unwired: 6 in, 2 out]
            }
            frame "1" {
              w636 = 1 ("input 4")
              w647 = "%Y-%m-%d " ("time format string (%c)")
              n155 = Format Date/Time String(time format string (%c)=w647, seconds (now)=w646) -> (date/time string=w643:string)  [unwired: 1 in]
              n156 = Format Date/Time String(time format string (%c)=w647, seconds (now)=w645) -> (date/time string=w644:string)  [unwired: 1 in]
              n157 = Format Into String(format string="Select DATE,Production_Count,Station_ID,Stack_holder_ID\nfrom Production_COUNT\nWhere DATE between '%s' and '%s' and Shift_ID='%s'and Stack_holder_ID='%d'\nand Station_ID='%d'" ("string"), w644, w643, w637, w636, w636) -> (resulting string=w640:string)  [unwired: 2 in, 1 out]
              n158 = call "Execute query.vi"("String"=w640, "connection reference"=w642) -> ("Table"=w639:string[][], "connection reference 2"=w638:T1)  [unwired: 6 in, 2 out]
            }
            frame "2" {
              w648 = 1 ("input 4")
              w659 = "%Y-%m-%d " ("time format string (%c)")
              n159 = Format Date/Time String(time format string (%c)=w659, seconds (now)=w658) -> (date/time string=w655:string)  [unwired: 1 in]
              n160 = Format Date/Time String(time format string (%c)=w659, seconds (now)=w657) -> (date/time string=w656:string)  [unwired: 1 in]
              n161 = Format Into String(format string="Select DATE,Production_Count,Station_ID,Stack_holder_ID\nfrom Production_COUNT\nWhere DATE between '%s' and '%s' and Shift_ID='%s'and Stack_holder_ID='%d'\nand Station_ID='%d'" ("string"), w656, w655, w649, w648, w648) -> (resulting string=w652:string)  [unwired: 2 in, 1 out]
              n162 = call "Execute query.vi"("String"=w652, "connection reference"=w654) -> ("Table"=w651:string[][], "connection reference 2"=w650:T1)  [unwired: 6 in, 2 out]
            }
            frame "3" {
              w660 = 1 ("input 4")
              w671 = "%Y-%m-%d " ("time format string (%c)")
              n163 = Format Date/Time String(time format string (%c)=w671, seconds (now)=w670) -> (date/time string=w667:string)  [unwired: 1 in]
              n164 = Format Date/Time String(time format string (%c)=w671, seconds (now)=w669) -> (date/time string=w668:string)  [unwired: 1 in]
              n165 = Format Into String(format string="Select DATE,Production_Count,Station_ID,Stack_holder_ID\nfrom Production_COUNT\nWhere DATE between '%s' and '%s' and Shift_ID='%s'and Stack_holder_ID='%d'\nand Station_ID='%d'" ("string"), w668, w667, w661, w660, w660) -> (resulting string=w664:string)  [unwired: 2 in, 1 out]
              n166 = call "Execute query.vi"("String"=w664, "connection reference"=w666) -> ("Table"=w663:string[][], "connection reference 2"=w662:T1)  [unwired: 6 in, 2 out]
            }
          }
        }
        frame "Maintenance" {
          n167 = case shown="\"ALL\"" w678 {
            selector: w678 -> [_ _ w694 w707 w720]
            tunnel: w677 -> [_ w690 w703 w716 w729]
            tunnel: w676 -> [_ w689 w702 w715 w728]
            tunnel: w675 -> [_ _ _ _ _]
            tunnel: [_ w683 w696 w709 w722] -> w674
            tunnel: w673 -> [w679 w686 w699 w712 w725]
            tunnel: [w679 w682 w695 w708 w721] -> w672
            frame "False", Default {
            }
            frame "ALL" {
              w691 = "%Y-%m-%d " ("time format string (%c)")
              n168 = Format Date/Time String(time format string (%c)=w691, seconds (now)=w689) -> (date/time string=w688:string)  [unwired: 1 in]
              n169 = Format Date/Time String(time format string (%c)=w691, seconds (now)=w690) -> (date/time string=w687:string)  [unwired: 1 in]
              n170 = Format Into String(format string="Select DATE,Production_Count,Station_ID,Stack_holder_ID\nfrom Production_COUNT\nWhere DATE between '%s' and '%s' and Stack_holder_ID='%d'\nand Station_ID='%d'" ("string"), w688, w687, 3 ("input 3"), 1 ("input 4")) -> (resulting string=w684:string)  [unwired: 2 in, 1 out]
              n171 = call "Execute query.vi"("String"=w684, "connection reference"=w686) -> ("Table"=w683:string[][], "connection reference 2"=w682:T1)  [unwired: 6 in, 2 out]
            }
            frame "1" {
              w704 = "%Y-%m-%d " ("time format string (%c)")
              n172 = Format Date/Time String(time format string (%c)=w704, seconds (now)=w703) -> (date/time string=w700:string)  [unwired: 1 in]
              n173 = Format Date/Time String(time format string (%c)=w704, seconds (now)=w702) -> (date/time string=w701:string)  [unwired: 1 in]
              n174 = Format Into String(format string="Select DATE,Production_Count,Station_ID,Stack_holder_ID\nfrom Production_COUNT\nWhere DATE between '%s' and '%s' and Shift_ID='%s'and Stack_holder_ID='%d'\nand Station_ID='%d'" ("string"), w701, w700, w694, 3 ("input 4"), 1 ("input 5")) -> (resulting string=w697:string)  [unwired: 2 in, 1 out]
              n175 = call "Execute query.vi"("String"=w697, "connection reference"=w699) -> ("Table"=w696:string[][], "connection reference 2"=w695:T1)  [unwired: 6 in, 2 out]
            }
            frame "2" {
              w717 = "%Y-%m-%d " ("time format string (%c)")
              n176 = Format Date/Time String(time format string (%c)=w717, seconds (now)=w716) -> (date/time string=w713:string)  [unwired: 1 in]
              n177 = Format Date/Time String(time format string (%c)=w717, seconds (now)=w715) -> (date/time string=w714:string)  [unwired: 1 in]
              n178 = Format Into String(format string="Select DATE,Production_Count,Station_ID,Stack_holder_ID\nfrom Production_COUNT\nWhere DATE between '%s' and '%s' and Shift_ID='%s'and Stack_holder_ID='%d'\nand Station_ID='%d'" ("string"), w714, w713, w707, 3 ("input 4"), 1 ("input 5")) -> (resulting string=w710:string)  [unwired: 2 in, 1 out]
              n179 = call "Execute query.vi"("String"=w710, "connection reference"=w712) -> ("Table"=w709:string[][], "connection reference 2"=w708:T1)  [unwired: 6 in, 2 out]
            }
            frame "3" {
              w730 = "%Y-%m-%d " ("time format string (%c)")
              n180 = Format Date/Time String(time format string (%c)=w730, seconds (now)=w729) -> (date/time string=w726:string)  [unwired: 1 in]
              n181 = Format Date/Time String(time format string (%c)=w730, seconds (now)=w728) -> (date/time string=w727:string)  [unwired: 1 in]
              n182 = Format Into String(format string="Select DATE,Production_Count,Station_ID,Stack_holder_ID\nfrom Production_COUNT\nWhere DATE between '%s' and '%s' and Shift_ID='%s'and Stack_holder_ID='%d'\nand Station_ID='%d'" ("string"), w727, w726, w720, 3 ("input 4"), 1 ("input 5")) -> (resulting string=w723:string)  [unwired: 2 in, 1 out]
              n183 = call "Execute query.vi"("String"=w723, "connection reference"=w725) -> ("Table"=w722:string[][], "connection reference 2"=w721:T1)  [unwired: 6 in, 2 out]
            }
          }
        }
        frame "Quality" {
          n184 = case shown="\"ALL\"" w737 {
            selector: w737 -> [_ _ w753 w766 w779]
            tunnel: w736 -> [_ w749 w762 w775 w788]
            tunnel: w735 -> [_ w748 w761 w774 w787]
            tunnel: w734 -> [_ _ _ _ _]
            tunnel: [_ w742 w755 w768 w781] -> w733
            tunnel: w732 -> [w738 w745 w758 w771 w784]
            tunnel: [w738 w741 w754 w767 w780] -> w731
            frame "False", Default {
            }
            frame "ALL" {
              w750 = "%Y-%m-%d " ("time format string (%c)")
              n185 = Format Date/Time String(time format string (%c)=w750, seconds (now)=w748) -> (date/time string=w747:string)  [unwired: 1 in]
              n186 = Format Date/Time String(time format string (%c)=w750, seconds (now)=w749) -> (date/time string=w746:string)  [unwired: 1 in]
              n187 = Format Into String(format string="Select DATE,Production_Count,Station_ID,Stack_holder_ID\nfrom Production_COUNT\nWhere DATE between '%s' and '%s' and Stack_holder_ID='%d'\nand Station_ID='%d'" ("string"), w747, w746, 4 ("input 3"), 1 ("input 3")) -> (resulting string=w743:string)  [unwired: 2 in, 1 out]
              n188 = call "Execute query.vi"("String"=w743, "connection reference"=w745) -> ("Table"=w742:string[][], "connection reference 2"=w741:T1)  [unwired: 6 in, 2 out]
            }
            frame "1" {
              w763 = "%Y-%m-%d " ("time format string (%c)")
              n189 = Format Date/Time String(time format string (%c)=w763, seconds (now)=w762) -> (date/time string=w759:string)  [unwired: 1 in]
              n190 = Format Date/Time String(time format string (%c)=w763, seconds (now)=w761) -> (date/time string=w760:string)  [unwired: 1 in]
              n191 = Format Into String(format string="Select DATE,Production_Count,Station_ID,Stack_holder_ID\nfrom Production_COUNT\nWhere DATE between '%s' and '%s' and Shift_ID='%s'and Stack_holder_ID='%d'\nand Station_ID='%d'" ("string"), w760, w759, w753, 4 ("input 4"), 1 ("input 4")) -> (resulting string=w756:string)  [unwired: 2 in, 1 out]
              n192 = call "Execute query.vi"("String"=w756, "connection reference"=w758) -> ("Table"=w755:string[][], "connection reference 2"=w754:T1)  [unwired: 6 in, 2 out]
            }
            frame "2" {
              w776 = "%Y-%m-%d " ("time format string (%c)")
              n193 = Format Date/Time String(time format string (%c)=w776, seconds (now)=w775) -> (date/time string=w772:string)  [unwired: 1 in]
              n194 = Format Date/Time String(time format string (%c)=w776, seconds (now)=w774) -> (date/time string=w773:string)  [unwired: 1 in]
              n195 = Format Into String(format string="Select DATE,Production_Count,Station_ID,Stack_holder_ID\nfrom Production_COUNT\nWhere DATE between '%s' and '%s' and Shift_ID='%s'and Stack_holder_ID='%d'\nand Station_ID='%d'" ("string"), w773, w772, w766, 4 ("input 4"), 1 ("input 4")) -> (resulting string=w769:string)  [unwired: 2 in, 1 out]
              n196 = call "Execute query.vi"("String"=w769, "connection reference"=w771) -> ("Table"=w768:string[][], "connection reference 2"=w767:T1)  [unwired: 6 in, 2 out]
            }
            frame "3" {
              w789 = "%Y-%m-%d " ("time format string (%c)")
              n197 = Format Date/Time String(time format string (%c)=w789, seconds (now)=w788) -> (date/time string=w785:string)  [unwired: 1 in]
              n198 = Format Date/Time String(time format string (%c)=w789, seconds (now)=w787) -> (date/time string=w786:string)  [unwired: 1 in]
              n199 = Format Into String(format string="Select DATE,Production_Count,Station_ID,Stack_holder_ID\nfrom Production_COUNT\nWhere DATE between '%s' and '%s' and Shift_ID='%s'and Stack_holder_ID='%d'\nand Station_ID='%d'" ("string"), w786, w785, w779, 4 ("input 4"), 1 ("input 4")) -> (resulting string=w782:string)  [unwired: 2 in, 1 out]
              n200 = call "Execute query.vi"("String"=w782, "connection reference"=w784) -> ("Table"=w781:string[][], "connection reference 2"=w780:T1)  [unwired: 6 in, 2 out]
            }
          }
        }
        frame "Production" {
          n201 = case shown="\"ALL\"" w796 {
            selector: w796 -> [_ _ w812 w825 w838]
            tunnel: w795 -> [_ w808 w821 w834 w847]
            tunnel: w794 -> [_ w807 w820 w833 w846]
            tunnel: w793 -> [_ _ _ _ _]
            tunnel: [_ w801 w814 w827 w840] -> w792
            tunnel: w791 -> [w797 w804 w817 w830 w843]
            tunnel: [w797 w800 w813 w826 w839] -> w790
            frame "False", Default {
            }
            frame "ALL" {
              w809 = "%Y-%m-%d " ("time format string (%c)")
              n202 = Format Date/Time String(time format string (%c)=w809, seconds (now)=w807) -> (date/time string=w806:string)  [unwired: 1 in]
              n203 = Format Date/Time String(time format string (%c)=w809, seconds (now)=w808) -> (date/time string=w805:string)  [unwired: 1 in]
              n204 = Format Into String(format string="Select DATE,Production_Count,Station_ID,Stack_holder_ID\nfrom Production_COUNT\nWhere DATE between '%s' and '%s' and Stack_holder_ID='%d'\nand Station_ID='%d'" ("string"), w806, w805, 5 ("input 3"), 1 ("input 3")) -> (resulting string=w802:string)  [unwired: 2 in, 1 out]
              n205 = call "Execute query.vi"("String"=w802, "connection reference"=w804) -> ("Table"=w801:string[][], "connection reference 2"=w800:T1)  [unwired: 6 in, 2 out]
            }
            frame "1" {
              w822 = "%Y-%m-%d " ("time format string (%c)")
              n206 = Format Date/Time String(time format string (%c)=w822, seconds (now)=w821) -> (date/time string=w818:string)  [unwired: 1 in]
              n207 = Format Date/Time String(time format string (%c)=w822, seconds (now)=w820) -> (date/time string=w819:string)  [unwired: 1 in]
              n208 = Format Into String(format string="Select DATE,Production_Count,Station_ID,Stack_holder_ID\nfrom Production_COUNT\nWhere DATE between '%s' and '%s' and Shift_ID='%s'and Stack_holder_ID='%d'\nand Station_ID='%d'" ("string"), w819, w818, w812, 5 ("input 4"), 1 ("input 4")) -> (resulting string=w815:string)  [unwired: 2 in, 1 out]
              n209 = call "Execute query.vi"("String"=w815, "connection reference"=w817) -> ("Table"=w814:string[][], "connection reference 2"=w813:T1)  [unwired: 6 in, 2 out]
            }
            frame "2" {
              w835 = "%Y-%m-%d " ("time format string (%c)")
              n210 = Format Date/Time String(time format string (%c)=w835, seconds (now)=w834) -> (date/time string=w831:string)  [unwired: 1 in]
              n211 = Format Date/Time String(time format string (%c)=w835, seconds (now)=w833) -> (date/time string=w832:string)  [unwired: 1 in]
              n212 = Format Into String(format string="Select DATE,Production_Count,Station_ID,Stack_holder_ID\nfrom Production_COUNT\nWhere DATE between '%s' and '%s' and Shift_ID='%s'and Stack_holder_ID='%d'\nand Station_ID='%d'" ("string"), w832, w831, w825, 5 ("input 4"), 1 ("input 4")) -> (resulting string=w828:string)  [unwired: 2 in, 1 out]
              n213 = call "Execute query.vi"("String"=w828, "connection reference"=w830) -> ("Table"=w827:string[][], "connection reference 2"=w826:T1)  [unwired: 6 in, 2 out]
            }
            frame "3" {
              w848 = "%Y-%m-%d " ("time format string (%c)")
              n214 = Format Date/Time String(time format string (%c)=w848, seconds (now)=w847) -> (date/time string=w844:string)  [unwired: 1 in]
              n215 = Format Date/Time String(time format string (%c)=w848, seconds (now)=w846) -> (date/time string=w845:string)  [unwired: 1 in]
              n216 = Format Into String(format string="Select DATE,Production_Count,Station_ID,Stack_holder_ID\nfrom Production_COUNT\nWhere DATE between '%s' and '%s' and Shift_ID='%s'and Stack_holder_ID='%d'\nand Station_ID='%d'" ("string"), w845, w844, w838, 5 ("input 4"), 1 ("input 4")) -> (resulting string=w841:string)  [unwired: 2 in, 1 out]
              n217 = call "Execute query.vi"("String"=w841, "connection reference"=w843) -> ("Table"=w840:string[][], "connection reference 2"=w839:T1)  [unwired: 6 in, 2 out]
            }
          }
        }
      }
    }
    frame "ST 2" {
      n218 = case shown="\"ALL\", Default" w855 {
        tunnel: w861 -> [w873 w974 w1033 w1089 w1148 w1207]
        tunnel: w860 -> [w872 w973 w1032 w1088 w1147 w1206]
        tunnel: w859 -> [w871 w972 w1031 w1087 w1146 w1205]
        tunnel: w858 -> [w870 w971 w1030 w1086 w1145 w1204]
        tunnel: [w869 w970 w1029 w1085 w1144 w1203] -> w852
        tunnel: w857 -> [w868 w969 w1028 w1084 w1143 w1202]
        tunnel: [w867 w968 w1027 w1083 w1142 w1201] -> w856
        tunnel: w854 -> [w866 _ _ _ _ _]
        tunnel: w853 -> [w865 _ _ _ _ _]
        tunnel: w851 -> [w864 _ _ _ _ _]
        tunnel: [w863 _ _ _ _ _] -> w850
        tunnel: w849 -> [w862 _ _ _ _ _]
        frame "ALL", Default {
          n219 = case shown="\"ALL\", Default" w873 {
            selector: w873 -> [_ w898 w922 w946]
            tunnel: w872 -> [_ _ _ _]
            tunnel: w871 -> [_ _ _ _]
            tunnel: w870 -> [_ _ _ _]
            tunnel: [w876 w899 w923 w947] -> w869
            tunnel: w868 -> [w881 w904 w928 w952]
            tunnel: [w880 w903 w927 w951] -> w867
            tunnel: w866 -> [w879 w902 w926 w950]
            tunnel: w865 -> [_ _ _ _]
            tunnel: w864 -> [w878 w901 w925 w949]
            tunnel: [w875 w897 w921 w945] -> w863
            tunnel: w862 -> [w874 w896 w920 w944]
            frame "ALL", Default {
              n220 = for {
                tunnel: w879 -> [w891]
                shift-right: [w893] -> w880
                shift-left: w881 -> [w895]
                tunnel: w878 -> [w887] mode=indexing
                shift-right: [w884] -> w876
                shift-left: string[][] [] -> [w886]
                tunnel: [w882] -> w875
                tunnel: w874 -> [w883]
                n221 = Concatenate Strings("Select DISTINCT PLAN_DATE,PRODUCTION_COUNT,STATION_ID from  ", w887, " Where year(PLAN_DATE) ='%s' and STATION_ID='%d'\n") -> (w888:string)
                n222 = Format Into String(format string=w888, w891, 2 ("input 3")) -> (resulting string=w894:string)  [unwired: 2 in, 1 out]
                n223 = call "Execute query.vi"("error in (no error)"=w883, "String"=w894, "connection reference"=w895) -> ("error out"=w882:errorcluster, "Table"=w885:string[][], "connection reference 2"=w893:T1)  [unwired: 5 in, 1 out]
                n224 = Build Array (concatenate)(w886, w885) -> (w884:string[][])
              }
            }
            frame "1" {
              n225 = for {
                tunnel: w902 -> [w915]
                shift-right: [w917] -> w903
                shift-left: w904 -> [w919]
                tunnel: w901 -> [w911] mode=indexing
                shift-right: [w908] -> w899
                shift-left: string[][] [] -> [w910]
                tunnel: w898 -> [w907]
                tunnel: [w905] -> w897
                tunnel: w896 -> [w906]
                n226 = Concatenate Strings("Select DISTINCT PLAN_DATE,PRODUCTION_COUNT,STATION_ID from  ", w911, " Where year(PLAN_DATE) ='%s' and STATION_ID='%d' and  SHIFT='%s'\n") -> (w912:string)
                n227 = Format Into String(format string=w912, w915, 2 ("input 3"), w907) -> (resulting string=w918:string)  [unwired: 2 in, 1 out]
                n228 = call "Execute query.vi"("error in (no error)"=w906, "String"=w918, "connection reference"=w919) -> ("error out"=w905:errorcluster, "Table"=w909:string[][], "connection reference 2"=w917:T1)  [unwired: 5 in, 1 out]
                n229 = Build Array (concatenate)(w910, w909) -> (w908:string[][])
              }
            }
            frame "2" {
              n230 = for {
                tunnel: w926 -> [w939]
                shift-right: [w941] -> w927
                shift-left: w928 -> [w943]
                tunnel: w925 -> [w935] mode=indexing
                shift-right: [w932] -> w923
                shift-left: string[][] [] -> [w934]
                tunnel: w922 -> [w931]
                tunnel: [w929] -> w921
                tunnel: w920 -> [w930]
                n231 = Concatenate Strings("Select DISTINCT PLAN_DATE,PRODUCTION_COUNT,STATION_ID from  ", w935, " Where year(PLAN_DATE) ='%s' and STATION_ID='%d' and SHIFT='%s'\n") -> (w936:string)
                n232 = Format Into String(format string=w936, w939, 2 ("input 3"), w931) -> (resulting string=w942:string)  [unwired: 2 in, 1 out]
                n233 = call "Execute query.vi"("error in (no error)"=w930, "String"=w942, "connection reference"=w943) -> ("error out"=w929:errorcluster, "Table"=w933:string[][], "connection reference 2"=w941:T1)  [unwired: 5 in, 1 out]
                n234 = Build Array (concatenate)(w934, w933) -> (w932:string[][])
              }
            }
            frame "3" {
              n235 = for {
                tunnel: w950 -> [w963]
                shift-right: [w965] -> w951
                shift-left: w952 -> [w967]
                tunnel: w949 -> [w959] mode=indexing
                shift-right: [w956] -> w947
                shift-left: string[][] [] -> [w958]
                tunnel: w946 -> [w955]
                tunnel: [w953] -> w945
                tunnel: w944 -> [w954]
                n236 = Concatenate Strings("Select DISTINCT PLAN_DATE,PRODUCTION_COUNT,STATION_ID from  ", w959, " Where year(PLAN_DATE) ='%s' and STATION_ID='%d' and  SHIFT='%s'\n") -> (w960:string)
                n237 = Format Into String(format string=w960, w963, 2 ("input 3"), w955) -> (resulting string=w966:string)  [unwired: 2 in, 1 out]
                n238 = call "Execute query.vi"("error in (no error)"=w954, "String"=w966, "connection reference"=w967) -> ("error out"=w953:errorcluster, "Table"=w957:string[][], "connection reference 2"=w965:T1)  [unwired: 5 in, 1 out]
                n239 = Build Array (concatenate)(w958, w957) -> (w956:string[][])
              }
            }
          }
        }
        frame "Logistics" {
          n240 = case shown="\"ALL\"" w974 {
            selector: w974 -> [_ _ w990 w1003 w1016]
            tunnel: w973 -> [_ w986 w999 w1012 w1025]
            tunnel: w972 -> [_ w985 w998 w1011 w1024]
            tunnel: w971 -> [_ _ _ _ _]
            tunnel: [_ w979 w992 w1005 w1018] -> w970
            tunnel: w969 -> [w975 w982 w995 w1008 w1021]
            tunnel: [w975 w978 w991 w1004 w1017] -> w968
            frame "False", Default {
            }
            frame "ALL" {
              w987 = "%Y-%m-%d " ("time format string (%c)")
              n241 = Format Date/Time String(time format string (%c)=w987, seconds (now)=w985) -> (date/time string=w984:string)  [unwired: 1 in]
              n242 = Format Date/Time String(time format string (%c)=w987, seconds (now)=w986) -> (date/time string=w983:string)  [unwired: 1 in]
              n243 = Format Into String(format string="Select DATE,Production_Count,Station_ID,Stack_holder_ID\nfrom Production_COUNT\nWhere DATE between '%s' and '%s' and Stack_holder_ID='%d'\nand Station_ID='%d'" ("string"), w984, w983, 2 ("input 3"), 1 ("input 4")) -> (resulting string=w980:string)  [unwired: 2 in, 1 out]
              n244 = call "Execute query.vi"("String"=w980, "connection reference"=w982) -> ("Table"=w979:string[][], "connection reference 2"=w978:T1)  [unwired: 6 in, 2 out]
            }
            frame "1" {
              w1000 = "%Y-%m-%d " ("time format string (%c)")
              n245 = Format Date/Time String(time format string (%c)=w1000, seconds (now)=w999) -> (date/time string=w996:string)  [unwired: 1 in]
              n246 = Format Date/Time String(time format string (%c)=w1000, seconds (now)=w998) -> (date/time string=w997:string)  [unwired: 1 in]
              n247 = Format Into String(format string="Select DATE,Production_Count,Station_ID,Stack_holder_ID\nfrom Production_COUNT\nWhere DATE between '%s' and '%s' and Shift_ID='%s'and Stack_holder_ID='%d'\nand Station_ID='%d'" ("string"), w997, w996, w990, 2 ("input 4"), 1 ("input 4")) -> (resulting string=w993:string)  [unwired: 2 in, 1 out]
              n248 = call "Execute query.vi"("String"=w993, "connection reference"=w995) -> ("Table"=w992:string[][], "connection reference 2"=w991:T1)  [unwired: 6 in, 2 out]
            }
            frame "2" {
              w1013 = "%Y-%m-%d " ("time format string (%c)")
              n249 = Format Date/Time String(time format string (%c)=w1013, seconds (now)=w1012) -> (date/time string=w1009:string)  [unwired: 1 in]
              n250 = Format Date/Time String(time format string (%c)=w1013, seconds (now)=w1011) -> (date/time string=w1010:string)  [unwired: 1 in]
              n251 = Format Into String(format string="Select DATE,Production_Count,Station_ID,Stack_holder_ID\nfrom Production_COUNT\nWhere DATE between '%s' and '%s' and Shift_ID='%s'and Stack_holder_ID='%d'\nand Station_ID='%d'" ("string"), w1010, w1009, w1003, 2 ("input 4"), 1 ("input 4")) -> (resulting string=w1006:string)  [unwired: 2 in, 1 out]
              n252 = call "Execute query.vi"("String"=w1006, "connection reference"=w1008) -> ("Table"=w1005:string[][], "connection reference 2"=w1004:T1)  [unwired: 6 in, 2 out]
            }
            frame "3" {
              w1026 = "%Y-%m-%d " ("time format string (%c)")
              n253 = Format Date/Time String(time format string (%c)=w1026, seconds (now)=w1025) -> (date/time string=w1022:string)  [unwired: 1 in]
              n254 = Format Date/Time String(time format string (%c)=w1026, seconds (now)=w1024) -> (date/time string=w1023:string)  [unwired: 1 in]
              n255 = Format Into String(format string="Select DATE,Production_Count,Station_ID,Stack_holder_ID\nfrom Production_COUNT\nWhere DATE between '%s' and '%s' and Shift_ID='%s'and Stack_holder_ID='%d'\nand Station_ID='%d'" ("string"), w1023, w1022, w1016, 2 ("input 4"), 1 ("input 4")) -> (resulting string=w1019:string)  [unwired: 2 in, 1 out]
              n256 = call "Execute query.vi"("String"=w1019, "connection reference"=w1021) -> ("Table"=w1018:string[][], "connection reference 2"=w1017:T1)  [unwired: 6 in, 2 out]
            }
          }
        }
        frame "Gap Leader" {
          n257 = case shown="\"3\"" w1033 {
            selector: w1033 -> [_ _ w1048 w1060 w1072]
            tunnel: w1032 -> [_ w1045 w1057 w1069 w1081]
            tunnel: w1031 -> [_ w1044 w1056 w1068 w1080]
            tunnel: w1030 -> [_ _ _ _ _]
            tunnel: [_ w1038 w1050 w1062 w1074] -> w1029
            tunnel: w1028 -> [w1034 w1041 w1053 w1065 w1077]
            tunnel: [w1034 w1037 w1049 w1061 w1073] -> w1027
            frame "False", Default {
            }
            frame "ALL" {
              w1046 = "%Y-%m-%d " ("time format string (%c)")
              n258 = Format Date/Time String(time format string (%c)=w1046, seconds (now)=w1044) -> (date/time string=w1043:string)  [unwired: 1 in]
              n259 = Format Date/Time String(time format string (%c)=w1046, seconds (now)=w1045) -> (date/time string=w1042:string)  [unwired: 1 in]
              n260 = Format Into String(format string="Select DATE,Production_Count,Station_ID,Stack_holder_ID\nfrom Production_COUNT\nWhere DATE between '%s' and '%s' and Stack_holder_ID='%d'\nand Station_ID='%d'" ("string"), w1043, w1042, 1 ("input 3"), 1 ("input 3")) -> (resulting string=w1039:string)  [unwired: 2 in, 1 out]
              n261 = call "Execute query.vi"("String"=w1039, "connection reference"=w1041) -> ("Table"=w1038:string[][], "connection reference 2"=w1037:T1)  [unwired: 6 in, 2 out]
            }
            frame "1" {
              w1047 = 1 ("input 4")
              w1058 = "%Y-%m-%d " ("time format string (%c)")
              n262 = Format Date/Time String(time format string (%c)=w1058, seconds (now)=w1057) -> (date/time string=w1054:string)  [unwired: 1 in]
              n263 = Format Date/Time String(time format string (%c)=w1058, seconds (now)=w1056) -> (date/time string=w1055:string)  [unwired: 1 in]
              n264 = Format Into String(format string="Select DATE,Production_Count,Station_ID,Stack_holder_ID\nfrom Production_COUNT\nWhere DATE between '%s' and '%s' and Shift_ID='%s'and Stack_holder_ID='%d'\nand Station_ID='%d'" ("string"), w1055, w1054, w1048, w1047, w1047) -> (resulting string=w1051:string)  [unwired: 2 in, 1 out]
              n265 = call "Execute query.vi"("String"=w1051, "connection reference"=w1053) -> ("Table"=w1050:string[][], "connection reference 2"=w1049:T1)  [unwired: 6 in, 2 out]
            }
            frame "2" {
              w1059 = 1 ("input 4")
              w1070 = "%Y-%m-%d " ("time format string (%c)")
              n266 = Format Date/Time String(time format string (%c)=w1070, seconds (now)=w1069) -> (date/time string=w1066:string)  [unwired: 1 in]
              n267 = Format Date/Time String(time format string (%c)=w1070, seconds (now)=w1068) -> (date/time string=w1067:string)  [unwired: 1 in]
              n268 = Format Into String(format string="Select DATE,Production_Count,Station_ID,Stack_holder_ID\nfrom Production_COUNT\nWhere DATE between '%s' and '%s' and Shift_ID='%s'and Stack_holder_ID='%d'\nand Station_ID='%d'" ("string"), w1067, w1066, w1060, w1059, w1059) -> (resulting string=w1063:string)  [unwired: 2 in, 1 out]
              n269 = call "Execute query.vi"("String"=w1063, "connection reference"=w1065) -> ("Table"=w1062:string[][], "connection reference 2"=w1061:T1)  [unwired: 6 in, 2 out]
            }
            frame "3" {
              w1071 = 1 ("input 4")
              w1082 = "%Y-%m-%d " ("time format string (%c)")
              n270 = Format Date/Time String(time format string (%c)=w1082, seconds (now)=w1081) -> (date/time string=w1078:string)  [unwired: 1 in]
              n271 = Format Date/Time String(time format string (%c)=w1082, seconds (now)=w1080) -> (date/time string=w1079:string)  [unwired: 1 in]
              n272 = Format Into String(format string="Select DATE,Production_Count,Station_ID,Stack_holder_ID\nfrom Production_COUNT\nWhere DATE between '%s' and '%s' and Shift_ID='%s'and Stack_holder_ID='%d'\nand Station_ID='%d'" ("string"), w1079, w1078, w1072, w1071, w1071) -> (resulting string=w1075:string)  [unwired: 2 in, 1 out]
              n273 = call "Execute query.vi"("String"=w1075, "connection reference"=w1077) -> ("Table"=w1074:string[][], "connection reference 2"=w1073:T1)  [unwired: 6 in, 2 out]
            }
          }
        }
        frame "Maintenance" {
          n274 = case shown="\"ALL\"" w1089 {
            selector: w1089 -> [_ _ w1105 w1118 w1131]
            tunnel: w1088 -> [_ w1101 w1114 w1127 w1140]
            tunnel: w1087 -> [_ w1100 w1113 w1126 w1139]
            tunnel: w1086 -> [_ _ _ _ _]
            tunnel: [_ w1094 w1107 w1120 w1133] -> w1085
            tunnel: w1084 -> [w1090 w1097 w1110 w1123 w1136]
            tunnel: [w1090 w1093 w1106 w1119 w1132] -> w1083
            frame "False", Default {
            }
            frame "ALL" {
              w1102 = "%Y-%m-%d " ("time format string (%c)")
              n275 = Format Date/Time String(time format string (%c)=w1102, seconds (now)=w1100) -> (date/time string=w1099:string)  [unwired: 1 in]
              n276 = Format Date/Time String(time format string (%c)=w1102, seconds (now)=w1101) -> (date/time string=w1098:string)  [unwired: 1 in]
              n277 = Format Into String(format string="Select DATE,Production_Count,Station_ID,Stack_holder_ID\nfrom Production_COUNT\nWhere DATE between '%s' and '%s' and Stack_holder_ID='%d'\nand Station_ID='%d'" ("string"), w1099, w1098, 3 ("input 3"), 1 ("input 4")) -> (resulting string=w1095:string)  [unwired: 2 in, 1 out]
              n278 = call "Execute query.vi"("String"=w1095, "connection reference"=w1097) -> ("Table"=w1094:string[][], "connection reference 2"=w1093:T1)  [unwired: 6 in, 2 out]
            }
            frame "1" {
              w1115 = "%Y-%m-%d " ("time format string (%c)")
              n279 = Format Date/Time String(time format string (%c)=w1115, seconds (now)=w1114) -> (date/time string=w1111:string)  [unwired: 1 in]
              n280 = Format Date/Time String(time format string (%c)=w1115, seconds (now)=w1113) -> (date/time string=w1112:string)  [unwired: 1 in]
              n281 = Format Into String(format string="Select DATE,Production_Count,Station_ID,Stack_holder_ID\nfrom Production_COUNT\nWhere DATE between '%s' and '%s' and Shift_ID='%s'and Stack_holder_ID='%d'\nand Station_ID='%d'" ("string"), w1112, w1111, w1105, 3 ("input 4"), 1 ("input 5")) -> (resulting string=w1108:string)  [unwired: 2 in, 1 out]
              n282 = call "Execute query.vi"("String"=w1108, "connection reference"=w1110) -> ("Table"=w1107:string[][], "connection reference 2"=w1106:T1)  [unwired: 6 in, 2 out]
            }
            frame "2" {
              w1128 = "%Y-%m-%d " ("time format string (%c)")
              n283 = Format Date/Time String(time format string (%c)=w1128, seconds (now)=w1127) -> (date/time string=w1124:string)  [unwired: 1 in]
              n284 = Format Date/Time String(time format string (%c)=w1128, seconds (now)=w1126) -> (date/time string=w1125:string)  [unwired: 1 in]
              n285 = Format Into String(format string="Select DATE,Production_Count,Station_ID,Stack_holder_ID\nfrom Production_COUNT\nWhere DATE between '%s' and '%s' and Shift_ID='%s'and Stack_holder_ID='%d'\nand Station_ID='%d'" ("string"), w1125, w1124, w1118, 3 ("input 4"), 1 ("input 5")) -> (resulting string=w1121:string)  [unwired: 2 in, 1 out]
              n286 = call "Execute query.vi"("String"=w1121, "connection reference"=w1123) -> ("Table"=w1120:string[][], "connection reference 2"=w1119:T1)  [unwired: 6 in, 2 out]
            }
            frame "3" {
              w1141 = "%Y-%m-%d " ("time format string (%c)")
              n287 = Format Date/Time String(time format string (%c)=w1141, seconds (now)=w1140) -> (date/time string=w1137:string)  [unwired: 1 in]
              n288 = Format Date/Time String(time format string (%c)=w1141, seconds (now)=w1139) -> (date/time string=w1138:string)  [unwired: 1 in]
              n289 = Format Into String(format string="Select DATE,Production_Count,Station_ID,Stack_holder_ID\nfrom Production_COUNT\nWhere DATE between '%s' and '%s' and Shift_ID='%s'and Stack_holder_ID='%d'\nand Station_ID='%d'" ("string"), w1138, w1137, w1131, 3 ("input 4"), 1 ("input 5")) -> (resulting string=w1134:string)  [unwired: 2 in, 1 out]
              n290 = call "Execute query.vi"("String"=w1134, "connection reference"=w1136) -> ("Table"=w1133:string[][], "connection reference 2"=w1132:T1)  [unwired: 6 in, 2 out]
            }
          }
        }
        frame "Quality" {
          n291 = case shown="\"ALL\"" w1148 {
            selector: w1148 -> [_ _ w1164 w1177 w1190]
            tunnel: w1147 -> [_ w1160 w1173 w1186 w1199]
            tunnel: w1146 -> [_ w1159 w1172 w1185 w1198]
            tunnel: w1145 -> [_ _ _ _ _]
            tunnel: [_ w1153 w1166 w1179 w1192] -> w1144
            tunnel: w1143 -> [w1149 w1156 w1169 w1182 w1195]
            tunnel: [w1149 w1152 w1165 w1178 w1191] -> w1142
            frame "False", Default {
            }
            frame "ALL" {
              w1161 = "%Y-%m-%d " ("time format string (%c)")
              n292 = Format Date/Time String(time format string (%c)=w1161, seconds (now)=w1159) -> (date/time string=w1158:string)  [unwired: 1 in]
              n293 = Format Date/Time String(time format string (%c)=w1161, seconds (now)=w1160) -> (date/time string=w1157:string)  [unwired: 1 in]
              n294 = Format Into String(format string="Select DATE,Production_Count,Station_ID,Stack_holder_ID\nfrom Production_COUNT\nWhere DATE between '%s' and '%s' and Stack_holder_ID='%d'\nand Station_ID='%d'" ("string"), w1158, w1157, 4 ("input 3"), 1 ("input 3")) -> (resulting string=w1154:string)  [unwired: 2 in, 1 out]
              n295 = call "Execute query.vi"("String"=w1154, "connection reference"=w1156) -> ("Table"=w1153:string[][], "connection reference 2"=w1152:T1)  [unwired: 6 in, 2 out]
            }
            frame "1" {
              w1174 = "%Y-%m-%d " ("time format string (%c)")
              n296 = Format Date/Time String(time format string (%c)=w1174, seconds (now)=w1173) -> (date/time string=w1170:string)  [unwired: 1 in]
              n297 = Format Date/Time String(time format string (%c)=w1174, seconds (now)=w1172) -> (date/time string=w1171:string)  [unwired: 1 in]
              n298 = Format Into String(format string="Select DATE,Production_Count,Station_ID,Stack_holder_ID\nfrom Production_COUNT\nWhere DATE between '%s' and '%s' and Shift_ID='%s'and Stack_holder_ID='%d'\nand Station_ID='%d'" ("string"), w1171, w1170, w1164, 4 ("input 4"), 1 ("input 4")) -> (resulting string=w1167:string)  [unwired: 2 in, 1 out]
              n299 = call "Execute query.vi"("String"=w1167, "connection reference"=w1169) -> ("Table"=w1166:string[][], "connection reference 2"=w1165:T1)  [unwired: 6 in, 2 out]
            }
            frame "2" {
              w1187 = "%Y-%m-%d " ("time format string (%c)")
              n300 = Format Date/Time String(time format string (%c)=w1187, seconds (now)=w1186) -> (date/time string=w1183:string)  [unwired: 1 in]
              n301 = Format Date/Time String(time format string (%c)=w1187, seconds (now)=w1185) -> (date/time string=w1184:string)  [unwired: 1 in]
              n302 = Format Into String(format string="Select DATE,Production_Count,Station_ID,Stack_holder_ID\nfrom Production_COUNT\nWhere DATE between '%s' and '%s' and Shift_ID='%s'and Stack_holder_ID='%d'\nand Station_ID='%d'" ("string"), w1184, w1183, w1177, 4 ("input 4"), 1 ("input 4")) -> (resulting string=w1180:string)  [unwired: 2 in, 1 out]
              n303 = call "Execute query.vi"("String"=w1180, "connection reference"=w1182) -> ("Table"=w1179:string[][], "connection reference 2"=w1178:T1)  [unwired: 6 in, 2 out]
            }
            frame "3" {
              w1200 = "%Y-%m-%d " ("time format string (%c)")
              n304 = Format Date/Time String(time format string (%c)=w1200, seconds (now)=w1199) -> (date/time string=w1196:string)  [unwired: 1 in]
              n305 = Format Date/Time String(time format string (%c)=w1200, seconds (now)=w1198) -> (date/time string=w1197:string)  [unwired: 1 in]
              n306 = Format Into String(format string="Select DATE,Production_Count,Station_ID,Stack_holder_ID\nfrom Production_COUNT\nWhere DATE between '%s' and '%s' and Shift_ID='%s'and Stack_holder_ID='%d'\nand Station_ID='%d'" ("string"), w1197, w1196, w1190, 4 ("input 4"), 1 ("input 4")) -> (resulting string=w1193:string)  [unwired: 2 in, 1 out]
              n307 = call "Execute query.vi"("String"=w1193, "connection reference"=w1195) -> ("Table"=w1192:string[][], "connection reference 2"=w1191:T1)  [unwired: 6 in, 2 out]
            }
          }
        }
        frame "Production" {
          n308 = case shown="\"ALL\"" w1207 {
            selector: w1207 -> [_ _ w1223 w1236 w1249]
            tunnel: w1206 -> [_ w1219 w1232 w1245 w1258]
            tunnel: w1205 -> [_ w1218 w1231 w1244 w1257]
            tunnel: w1204 -> [_ _ _ _ _]
            tunnel: [_ w1212 w1225 w1238 w1251] -> w1203
            tunnel: w1202 -> [w1208 w1215 w1228 w1241 w1254]
            tunnel: [w1208 w1211 w1224 w1237 w1250] -> w1201
            frame "False", Default {
            }
            frame "ALL" {
              w1220 = "%Y-%m-%d " ("time format string (%c)")
              n309 = Format Date/Time String(time format string (%c)=w1220, seconds (now)=w1218) -> (date/time string=w1217:string)  [unwired: 1 in]
              n310 = Format Date/Time String(time format string (%c)=w1220, seconds (now)=w1219) -> (date/time string=w1216:string)  [unwired: 1 in]
              n311 = Format Into String(format string="Select DATE,Production_Count,Station_ID,Stack_holder_ID\nfrom Production_COUNT\nWhere DATE between '%s' and '%s' and Stack_holder_ID='%d'\nand Station_ID='%d'" ("string"), w1217, w1216, 5 ("input 3"), 1 ("input 3")) -> (resulting string=w1213:string)  [unwired: 2 in, 1 out]
              n312 = call "Execute query.vi"("String"=w1213, "connection reference"=w1215) -> ("Table"=w1212:string[][], "connection reference 2"=w1211:T1)  [unwired: 6 in, 2 out]
            }
            frame "1" {
              w1233 = "%Y-%m-%d " ("time format string (%c)")
              n313 = Format Date/Time String(time format string (%c)=w1233, seconds (now)=w1232) -> (date/time string=w1229:string)  [unwired: 1 in]
              n314 = Format Date/Time String(time format string (%c)=w1233, seconds (now)=w1231) -> (date/time string=w1230:string)  [unwired: 1 in]
              n315 = Format Into String(format string="Select DATE,Production_Count,Station_ID,Stack_holder_ID\nfrom Production_COUNT\nWhere DATE between '%s' and '%s' and Shift_ID='%s'and Stack_holder_ID='%d'\nand Station_ID='%d'" ("string"), w1230, w1229, w1223, 5 ("input 4"), 1 ("input 4")) -> (resulting string=w1226:string)  [unwired: 2 in, 1 out]
              n316 = call "Execute query.vi"("String"=w1226, "connection reference"=w1228) -> ("Table"=w1225:string[][], "connection reference 2"=w1224:T1)  [unwired: 6 in, 2 out]
            }
            frame "2" {
              w1246 = "%Y-%m-%d " ("time format string (%c)")
              n317 = Format Date/Time String(time format string (%c)=w1246, seconds (now)=w1245) -> (date/time string=w1242:string)  [unwired: 1 in]
              n318 = Format Date/Time String(time format string (%c)=w1246, seconds (now)=w1244) -> (date/time string=w1243:string)  [unwired: 1 in]
              n319 = Format Into String(format string="Select DATE,Production_Count,Station_ID,Stack_holder_ID\nfrom Production_COUNT\nWhere DATE between '%s' and '%s' and Shift_ID='%s'and Stack_holder_ID='%d'\nand Station_ID='%d'" ("string"), w1243, w1242, w1236, 5 ("input 4"), 1 ("input 4")) -> (resulting string=w1239:string)  [unwired: 2 in, 1 out]
              n320 = call "Execute query.vi"("String"=w1239, "connection reference"=w1241) -> ("Table"=w1238:string[][], "connection reference 2"=w1237:T1)  [unwired: 6 in, 2 out]
            }
            frame "3" {
              w1259 = "%Y-%m-%d " ("time format string (%c)")
              n321 = Format Date/Time String(time format string (%c)=w1259, seconds (now)=w1258) -> (date/time string=w1255:string)  [unwired: 1 in]
              n322 = Format Date/Time String(time format string (%c)=w1259, seconds (now)=w1257) -> (date/time string=w1256:string)  [unwired: 1 in]
              n323 = Format Into String(format string="Select DATE,Production_Count,Station_ID,Stack_holder_ID\nfrom Production_COUNT\nWhere DATE between '%s' and '%s' and Shift_ID='%s'and Stack_holder_ID='%d'\nand Station_ID='%d'" ("string"), w1256, w1255, w1249, 5 ("input 4"), 1 ("input 4")) -> (resulting string=w1252:string)  [unwired: 2 in, 1 out]
              n324 = call "Execute query.vi"("String"=w1252, "connection reference"=w1254) -> ("Table"=w1251:string[][], "connection reference 2"=w1250:T1)  [unwired: 6 in, 2 out]
            }
          }
        }
      }
    }
    frame "ST 3" {
      n325 = case shown="\"ALL\", Default" w1266 {
        tunnel: w1272 -> [w1284 w1385 w1444 w1500 w1559 w1618]
        tunnel: w1271 -> [w1283 w1384 w1443 w1499 w1558 w1617]
        tunnel: w1270 -> [w1282 w1383 w1442 w1498 w1557 w1616]
        tunnel: w1269 -> [w1281 w1382 w1441 w1497 w1556 w1615]
        tunnel: [w1280 w1381 w1440 w1496 w1555 w1614] -> w1263
        tunnel: w1268 -> [w1279 w1380 w1439 w1495 w1554 w1613]
        tunnel: [w1278 w1379 w1438 w1494 w1553 w1612] -> w1267
        tunnel: w1265 -> [w1277 _ _ _ _ _]
        tunnel: w1264 -> [w1276 _ _ _ _ _]
        tunnel: w1262 -> [w1275 _ _ _ _ _]
        tunnel: [w1274 _ _ _ _ _] -> w1261
        tunnel: w1260 -> [w1273 _ _ _ _ _]
        frame "ALL", Default {
          n326 = case shown="\"3\"" w1284 {
            selector: w1284 -> [_ w1309 w1333 w1357]
            tunnel: w1283 -> [_ _ _ _]
            tunnel: w1282 -> [_ _ _ _]
            tunnel: w1281 -> [_ _ _ _]
            tunnel: [w1287 w1310 w1334 w1358] -> w1280
            tunnel: w1279 -> [w1292 w1315 w1339 w1363]
            tunnel: [w1291 w1314 w1338 w1362] -> w1278
            tunnel: w1277 -> [w1290 w1313 w1337 w1361]
            tunnel: w1276 -> [_ _ _ _]
            tunnel: w1275 -> [w1289 w1312 w1336 w1360]
            tunnel: [w1286 w1308 w1332 w1356] -> w1274
            tunnel: w1273 -> [w1285 w1307 w1331 w1355]
            frame "ALL", Default {
              n327 = for {
                tunnel: w1290 -> [w1302]
                shift-right: [w1304] -> w1291
                shift-left: w1292 -> [w1306]
                tunnel: w1289 -> [w1298] mode=indexing
                shift-right: [w1295] -> w1287
                shift-left: string[][] [] -> [w1297]
                tunnel: [w1293] -> w1286
                tunnel: w1285 -> [w1294]
                n328 = Concatenate Strings("Select DISTINCT PLAN_DATE,PRODUCTION_COUNT,STATION_ID from  ", w1298, " Where year(PLAN_DATE) ='%s' and STATION_ID='%d'\n") -> (w1299:string)
                n329 = Format Into String(format string=w1299, w1302, 3 ("input 3")) -> (resulting string=w1305:string)  [unwired: 2 in, 1 out]
                n330 = call "Execute query.vi"("error in (no error)"=w1294, "String"=w1305, "connection reference"=w1306) -> ("error out"=w1293:errorcluster, "Table"=w1296:string[][], "connection reference 2"=w1304:T1)  [unwired: 5 in, 1 out]
                n331 = Build Array (concatenate)(w1297, w1296) -> (w1295:string[][])
              }
            }
            frame "1" {
              n332 = for {
                tunnel: w1313 -> [w1326]
                shift-right: [w1328] -> w1314
                shift-left: w1315 -> [w1330]
                tunnel: w1312 -> [w1322] mode=indexing
                shift-right: [w1319] -> w1310
                shift-left: string[][] [] -> [w1321]
                tunnel: w1309 -> [w1318]
                tunnel: [w1316] -> w1308
                tunnel: w1307 -> [w1317]
                n333 = Concatenate Strings("Select DISTINCT PLAN_DATE,PRODUCTION_COUNT,STATION_ID from  ", w1322, " Where year(PLAN_DATE) ='%s' and STATION_ID='%d' and  SHIFT='%s'\n") -> (w1323:string)
                n334 = Format Into String(format string=w1323, w1326, 3 ("input 3"), w1318) -> (resulting string=w1329:string)  [unwired: 2 in, 1 out]
                n335 = call "Execute query.vi"("error in (no error)"=w1317, "String"=w1329, "connection reference"=w1330) -> ("error out"=w1316:errorcluster, "Table"=w1320:string[][], "connection reference 2"=w1328:T1)  [unwired: 5 in, 1 out]
                n336 = Build Array (concatenate)(w1321, w1320) -> (w1319:string[][])
              }
            }
            frame "2" {
              n337 = for {
                tunnel: w1337 -> [w1350]
                shift-right: [w1352] -> w1338
                shift-left: w1339 -> [w1354]
                tunnel: w1336 -> [w1346] mode=indexing
                shift-right: [w1343] -> w1334
                shift-left: string[][] [] -> [w1345]
                tunnel: w1333 -> [w1342]
                tunnel: [w1340] -> w1332
                tunnel: w1331 -> [w1341]
                n338 = Concatenate Strings("Select DISTINCT PLAN_DATE,PRODUCTION_COUNT,STATION_ID from  ", w1346, " Where year(PLAN_DATE) ='%s' and STATION_ID='%d' and SHIFT='%s'\n") -> (w1347:string)
                n339 = Format Into String(format string=w1347, w1350, 3 ("input 3"), w1342) -> (resulting string=w1353:string)  [unwired: 2 in, 1 out]
                n340 = call "Execute query.vi"("error in (no error)"=w1341, "String"=w1353, "connection reference"=w1354) -> ("error out"=w1340:errorcluster, "Table"=w1344:string[][], "connection reference 2"=w1352:T1)  [unwired: 5 in, 1 out]
                n341 = Build Array (concatenate)(w1345, w1344) -> (w1343:string[][])
              }
            }
            frame "3" {
              n342 = for {
                tunnel: w1361 -> [w1374]
                shift-right: [w1376] -> w1362
                shift-left: w1363 -> [w1378]
                tunnel: w1360 -> [w1370] mode=indexing
                shift-right: [w1367] -> w1358
                shift-left: string[][] [] -> [w1369]
                tunnel: w1357 -> [w1366]
                tunnel: [w1364] -> w1356
                tunnel: w1355 -> [w1365]
                n343 = Concatenate Strings("Select DISTINCT PLAN_DATE,PRODUCTION_COUNT,STATION_ID from  ", w1370, " Where year(PLAN_DATE) ='%s' and STATION_ID='%d' and  SHIFT='%s'\n") -> (w1371:string)
                n344 = Format Into String(format string=w1371, w1374, 3 ("input 3"), w1366) -> (resulting string=w1377:string)  [unwired: 2 in, 1 out]
                n345 = call "Execute query.vi"("error in (no error)"=w1365, "String"=w1377, "connection reference"=w1378) -> ("error out"=w1364:errorcluster, "Table"=w1368:string[][], "connection reference 2"=w1376:T1)  [unwired: 5 in, 1 out]
                n346 = Build Array (concatenate)(w1369, w1368) -> (w1367:string[][])
              }
            }
          }
        }
        frame "Logistics" {
          n347 = case shown="\"ALL\"" w1385 {
            selector: w1385 -> [_ _ w1401 w1414 w1427]
            tunnel: w1384 -> [_ w1397 w1410 w1423 w1436]
            tunnel: w1383 -> [_ w1396 w1409 w1422 w1435]
            tunnel: w1382 -> [_ _ _ _ _]
            tunnel: [_ w1390 w1403 w1416 w1429] -> w1381
            tunnel: w1380 -> [w1386 w1393 w1406 w1419 w1432]
            tunnel: [w1386 w1389 w1402 w1415 w1428] -> w1379
            frame "False", Default {
            }
            frame "ALL" {
              w1398 = "%Y-%m-%d " ("time format string (%c)")
              n348 = Format Date/Time String(time format string (%c)=w1398, seconds (now)=w1396) -> (date/time string=w1395:string)  [unwired: 1 in]
              n349 = Format Date/Time String(time format string (%c)=w1398, seconds (now)=w1397) -> (date/time string=w1394:string)  [unwired: 1 in]
              n350 = Format Into String(format string="Select DATE,Production_Count,Station_ID,Stack_holder_ID\nfrom Production_COUNT\nWhere DATE between '%s' and '%s' and Stack_holder_ID='%d'\nand Station_ID='%d'" ("string"), w1395, w1394, 2 ("input 3"), 1 ("input 4")) -> (resulting string=w1391:string)  [unwired: 2 in, 1 out]
              n351 = call "Execute query.vi"("String"=w1391, "connection reference"=w1393) -> ("Table"=w1390:string[][], "connection reference 2"=w1389:T1)  [unwired: 6 in, 2 out]
            }
            frame "1" {
              w1411 = "%Y-%m-%d " ("time format string (%c)")
              n352 = Format Date/Time String(time format string (%c)=w1411, seconds (now)=w1410) -> (date/time string=w1407:string)  [unwired: 1 in]
              n353 = Format Date/Time String(time format string (%c)=w1411, seconds (now)=w1409) -> (date/time string=w1408:string)  [unwired: 1 in]
              n354 = Format Into String(format string="Select DATE,Production_Count,Station_ID,Stack_holder_ID\nfrom Production_COUNT\nWhere DATE between '%s' and '%s' and Shift_ID='%s'and Stack_holder_ID='%d'\nand Station_ID='%d'" ("string"), w1408, w1407, w1401, 2 ("input 4"), 1 ("input 4")) -> (resulting string=w1404:string)  [unwired: 2 in, 1 out]
              n355 = call "Execute query.vi"("String"=w1404, "connection reference"=w1406) -> ("Table"=w1403:string[][], "connection reference 2"=w1402:T1)  [unwired: 6 in, 2 out]
            }
            frame "2" {
              w1424 = "%Y-%m-%d " ("time format string (%c)")
              n356 = Format Date/Time String(time format string (%c)=w1424, seconds (now)=w1423) -> (date/time string=w1420:string)  [unwired: 1 in]
              n357 = Format Date/Time String(time format string (%c)=w1424, seconds (now)=w1422) -> (date/time string=w1421:string)  [unwired: 1 in]
              n358 = Format Into String(format string="Select DATE,Production_Count,Station_ID,Stack_holder_ID\nfrom Production_COUNT\nWhere DATE between '%s' and '%s' and Shift_ID='%s'and Stack_holder_ID='%d'\nand Station_ID='%d'" ("string"), w1421, w1420, w1414, 2 ("input 4"), 1 ("input 4")) -> (resulting string=w1417:string)  [unwired: 2 in, 1 out]
              n359 = call "Execute query.vi"("String"=w1417, "connection reference"=w1419) -> ("Table"=w1416:string[][], "connection reference 2"=w1415:T1)  [unwired: 6 in, 2 out]
            }
            frame "3" {
              w1437 = "%Y-%m-%d " ("time format string (%c)")
              n360 = Format Date/Time String(time format string (%c)=w1437, seconds (now)=w1436) -> (date/time string=w1433:string)  [unwired: 1 in]
              n361 = Format Date/Time String(time format string (%c)=w1437, seconds (now)=w1435) -> (date/time string=w1434:string)  [unwired: 1 in]
              n362 = Format Into String(format string="Select DATE,Production_Count,Station_ID,Stack_holder_ID\nfrom Production_COUNT\nWhere DATE between '%s' and '%s' and Shift_ID='%s'and Stack_holder_ID='%d'\nand Station_ID='%d'" ("string"), w1434, w1433, w1427, 2 ("input 4"), 1 ("input 4")) -> (resulting string=w1430:string)  [unwired: 2 in, 1 out]
              n363 = call "Execute query.vi"("String"=w1430, "connection reference"=w1432) -> ("Table"=w1429:string[][], "connection reference 2"=w1428:T1)  [unwired: 6 in, 2 out]
            }
          }
        }
        frame "Gap Leader" {
          n364 = case shown="\"3\"" w1444 {
            selector: w1444 -> [_ _ w1459 w1471 w1483]
            tunnel: w1443 -> [_ w1456 w1468 w1480 w1492]
            tunnel: w1442 -> [_ w1455 w1467 w1479 w1491]
            tunnel: w1441 -> [_ _ _ _ _]
            tunnel: [_ w1449 w1461 w1473 w1485] -> w1440
            tunnel: w1439 -> [w1445 w1452 w1464 w1476 w1488]
            tunnel: [w1445 w1448 w1460 w1472 w1484] -> w1438
            frame "False", Default {
            }
            frame "ALL" {
              w1457 = "%Y-%m-%d " ("time format string (%c)")
              n365 = Format Date/Time String(time format string (%c)=w1457, seconds (now)=w1455) -> (date/time string=w1454:string)  [unwired: 1 in]
              n366 = Format Date/Time String(time format string (%c)=w1457, seconds (now)=w1456) -> (date/time string=w1453:string)  [unwired: 1 in]
              n367 = Format Into String(format string="Select DATE,Production_Count,Station_ID,Stack_holder_ID\nfrom Production_COUNT\nWhere DATE between '%s' and '%s' and Stack_holder_ID='%d'\nand Station_ID='%d'" ("string"), w1454, w1453, 1 ("input 3"), 1 ("input 3")) -> (resulting string=w1450:string)  [unwired: 2 in, 1 out]
              n368 = call "Execute query.vi"("String"=w1450, "connection reference"=w1452) -> ("Table"=w1449:string[][], "connection reference 2"=w1448:T1)  [unwired: 6 in, 2 out]
            }
            frame "1" {
              w1458 = 1 ("input 4")
              w1469 = "%Y-%m-%d " ("time format string (%c)")
              n369 = Format Date/Time String(time format string (%c)=w1469, seconds (now)=w1468) -> (date/time string=w1465:string)  [unwired: 1 in]
              n370 = Format Date/Time String(time format string (%c)=w1469, seconds (now)=w1467) -> (date/time string=w1466:string)  [unwired: 1 in]
              n371 = Format Into String(format string="Select DATE,Production_Count,Station_ID,Stack_holder_ID\nfrom Production_COUNT\nWhere DATE between '%s' and '%s' and Shift_ID='%s'and Stack_holder_ID='%d'\nand Station_ID='%d'" ("string"), w1466, w1465, w1459, w1458, w1458) -> (resulting string=w1462:string)  [unwired: 2 in, 1 out]
              n372 = call "Execute query.vi"("String"=w1462, "connection reference"=w1464) -> ("Table"=w1461:string[][], "connection reference 2"=w1460:T1)  [unwired: 6 in, 2 out]
            }
            frame "2" {
              w1470 = 1 ("input 4")
              w1481 = "%Y-%m-%d " ("time format string (%c)")
              n373 = Format Date/Time String(time format string (%c)=w1481, seconds (now)=w1480) -> (date/time string=w1477:string)  [unwired: 1 in]
              n374 = Format Date/Time String(time format string (%c)=w1481, seconds (now)=w1479) -> (date/time string=w1478:string)  [unwired: 1 in]
              n375 = Format Into String(format string="Select DATE,Production_Count,Station_ID,Stack_holder_ID\nfrom Production_COUNT\nWhere DATE between '%s' and '%s' and Shift_ID='%s'and Stack_holder_ID='%d'\nand Station_ID='%d'" ("string"), w1478, w1477, w1471, w1470, w1470) -> (resulting string=w1474:string)  [unwired: 2 in, 1 out]
              n376 = call "Execute query.vi"("String"=w1474, "connection reference"=w1476) -> ("Table"=w1473:string[][], "connection reference 2"=w1472:T1)  [unwired: 6 in, 2 out]
            }
            frame "3" {
              w1482 = 1 ("input 4")
              w1493 = "%Y-%m-%d " ("time format string (%c)")
              n377 = Format Date/Time String(time format string (%c)=w1493, seconds (now)=w1492) -> (date/time string=w1489:string)  [unwired: 1 in]
              n378 = Format Date/Time String(time format string (%c)=w1493, seconds (now)=w1491) -> (date/time string=w1490:string)  [unwired: 1 in]
              n379 = Format Into String(format string="Select DATE,Production_Count,Station_ID,Stack_holder_ID\nfrom Production_COUNT\nWhere DATE between '%s' and '%s' and Shift_ID='%s'and Stack_holder_ID='%d'\nand Station_ID='%d'" ("string"), w1490, w1489, w1483, w1482, w1482) -> (resulting string=w1486:string)  [unwired: 2 in, 1 out]
              n380 = call "Execute query.vi"("String"=w1486, "connection reference"=w1488) -> ("Table"=w1485:string[][], "connection reference 2"=w1484:T1)  [unwired: 6 in, 2 out]
            }
          }
        }
        frame "Maintenance" {
          n381 = case shown="\"ALL\"" w1500 {
            selector: w1500 -> [_ _ w1516 w1529 w1542]
            tunnel: w1499 -> [_ w1512 w1525 w1538 w1551]
            tunnel: w1498 -> [_ w1511 w1524 w1537 w1550]
            tunnel: w1497 -> [_ _ _ _ _]
            tunnel: [_ w1505 w1518 w1531 w1544] -> w1496
            tunnel: w1495 -> [w1501 w1508 w1521 w1534 w1547]
            tunnel: [w1501 w1504 w1517 w1530 w1543] -> w1494
            frame "False", Default {
            }
            frame "ALL" {
              w1513 = "%Y-%m-%d " ("time format string (%c)")
              n382 = Format Date/Time String(time format string (%c)=w1513, seconds (now)=w1511) -> (date/time string=w1510:string)  [unwired: 1 in]
              n383 = Format Date/Time String(time format string (%c)=w1513, seconds (now)=w1512) -> (date/time string=w1509:string)  [unwired: 1 in]
              n384 = Format Into String(format string="Select DATE,Production_Count,Station_ID,Stack_holder_ID\nfrom Production_COUNT\nWhere DATE between '%s' and '%s' and Stack_holder_ID='%d'\nand Station_ID='%d'" ("string"), w1510, w1509, 3 ("input 3"), 1 ("input 4")) -> (resulting string=w1506:string)  [unwired: 2 in, 1 out]
              n385 = call "Execute query.vi"("String"=w1506, "connection reference"=w1508) -> ("Table"=w1505:string[][], "connection reference 2"=w1504:T1)  [unwired: 6 in, 2 out]
            }
            frame "1" {
              w1526 = "%Y-%m-%d " ("time format string (%c)")
              n386 = Format Date/Time String(time format string (%c)=w1526, seconds (now)=w1525) -> (date/time string=w1522:string)  [unwired: 1 in]
              n387 = Format Date/Time String(time format string (%c)=w1526, seconds (now)=w1524) -> (date/time string=w1523:string)  [unwired: 1 in]
              n388 = Format Into String(format string="Select DATE,Production_Count,Station_ID,Stack_holder_ID\nfrom Production_COUNT\nWhere DATE between '%s' and '%s' and Shift_ID='%s'and Stack_holder_ID='%d'\nand Station_ID='%d'" ("string"), w1523, w1522, w1516, 3 ("input 4"), 1 ("input 5")) -> (resulting string=w1519:string)  [unwired: 2 in, 1 out]
              n389 = call "Execute query.vi"("String"=w1519, "connection reference"=w1521) -> ("Table"=w1518:string[][], "connection reference 2"=w1517:T1)  [unwired: 6 in, 2 out]
            }
            frame "2" {
              w1539 = "%Y-%m-%d " ("time format string (%c)")
              n390 = Format Date/Time String(time format string (%c)=w1539, seconds (now)=w1538) -> (date/time string=w1535:string)  [unwired: 1 in]
              n391 = Format Date/Time String(time format string (%c)=w1539, seconds (now)=w1537) -> (date/time string=w1536:string)  [unwired: 1 in]
              n392 = Format Into String(format string="Select DATE,Production_Count,Station_ID,Stack_holder_ID\nfrom Production_COUNT\nWhere DATE between '%s' and '%s' and Shift_ID='%s'and Stack_holder_ID='%d'\nand Station_ID='%d'" ("string"), w1536, w1535, w1529, 3 ("input 4"), 1 ("input 5")) -> (resulting string=w1532:string)  [unwired: 2 in, 1 out]
              n393 = call "Execute query.vi"("String"=w1532, "connection reference"=w1534) -> ("Table"=w1531:string[][], "connection reference 2"=w1530:T1)  [unwired: 6 in, 2 out]
            }
            frame "3" {
              w1552 = "%Y-%m-%d " ("time format string (%c)")
              n394 = Format Date/Time String(time format string (%c)=w1552, seconds (now)=w1551) -> (date/time string=w1548:string)  [unwired: 1 in]
              n395 = Format Date/Time String(time format string (%c)=w1552, seconds (now)=w1550) -> (date/time string=w1549:string)  [unwired: 1 in]
              n396 = Format Into String(format string="Select DATE,Production_Count,Station_ID,Stack_holder_ID\nfrom Production_COUNT\nWhere DATE between '%s' and '%s' and Shift_ID='%s'and Stack_holder_ID='%d'\nand Station_ID='%d'" ("string"), w1549, w1548, w1542, 3 ("input 4"), 1 ("input 5")) -> (resulting string=w1545:string)  [unwired: 2 in, 1 out]
              n397 = call "Execute query.vi"("String"=w1545, "connection reference"=w1547) -> ("Table"=w1544:string[][], "connection reference 2"=w1543:T1)  [unwired: 6 in, 2 out]
            }
          }
        }
        frame "Quality" {
          n398 = case shown="\"ALL\"" w1559 {
            selector: w1559 -> [_ _ w1575 w1588 w1601]
            tunnel: w1558 -> [_ w1571 w1584 w1597 w1610]
            tunnel: w1557 -> [_ w1570 w1583 w1596 w1609]
            tunnel: w1556 -> [_ _ _ _ _]
            tunnel: [_ w1564 w1577 w1590 w1603] -> w1555
            tunnel: w1554 -> [w1560 w1567 w1580 w1593 w1606]
            tunnel: [w1560 w1563 w1576 w1589 w1602] -> w1553
            frame "False", Default {
            }
            frame "ALL" {
              w1572 = "%Y-%m-%d " ("time format string (%c)")
              n399 = Format Date/Time String(time format string (%c)=w1572, seconds (now)=w1570) -> (date/time string=w1569:string)  [unwired: 1 in]
              n400 = Format Date/Time String(time format string (%c)=w1572, seconds (now)=w1571) -> (date/time string=w1568:string)  [unwired: 1 in]
              n401 = Format Into String(format string="Select DATE,Production_Count,Station_ID,Stack_holder_ID\nfrom Production_COUNT\nWhere DATE between '%s' and '%s' and Stack_holder_ID='%d'\nand Station_ID='%d'" ("string"), w1569, w1568, 4 ("input 3"), 1 ("input 3")) -> (resulting string=w1565:string)  [unwired: 2 in, 1 out]
              n402 = call "Execute query.vi"("String"=w1565, "connection reference"=w1567) -> ("Table"=w1564:string[][], "connection reference 2"=w1563:T1)  [unwired: 6 in, 2 out]
            }
            frame "1" {
              w1585 = "%Y-%m-%d " ("time format string (%c)")
              n403 = Format Date/Time String(time format string (%c)=w1585, seconds (now)=w1584) -> (date/time string=w1581:string)  [unwired: 1 in]
              n404 = Format Date/Time String(time format string (%c)=w1585, seconds (now)=w1583) -> (date/time string=w1582:string)  [unwired: 1 in]
              n405 = Format Into String(format string="Select DATE,Production_Count,Station_ID,Stack_holder_ID\nfrom Production_COUNT\nWhere DATE between '%s' and '%s' and Shift_ID='%s'and Stack_holder_ID='%d'\nand Station_ID='%d'" ("string"), w1582, w1581, w1575, 4 ("input 4"), 1 ("input 4")) -> (resulting string=w1578:string)  [unwired: 2 in, 1 out]
              n406 = call "Execute query.vi"("String"=w1578, "connection reference"=w1580) -> ("Table"=w1577:string[][], "connection reference 2"=w1576:T1)  [unwired: 6 in, 2 out]
            }
            frame "2" {
              w1598 = "%Y-%m-%d " ("time format string (%c)")
              n407 = Format Date/Time String(time format string (%c)=w1598, seconds (now)=w1597) -> (date/time string=w1594:string)  [unwired: 1 in]
              n408 = Format Date/Time String(time format string (%c)=w1598, seconds (now)=w1596) -> (date/time string=w1595:string)  [unwired: 1 in]
              n409 = Format Into String(format string="Select DATE,Production_Count,Station_ID,Stack_holder_ID\nfrom Production_COUNT\nWhere DATE between '%s' and '%s' and Shift_ID='%s'and Stack_holder_ID='%d'\nand Station_ID='%d'" ("string"), w1595, w1594, w1588, 4 ("input 4"), 1 ("input 4")) -> (resulting string=w1591:string)  [unwired: 2 in, 1 out]
              n410 = call "Execute query.vi"("String"=w1591, "connection reference"=w1593) -> ("Table"=w1590:string[][], "connection reference 2"=w1589:T1)  [unwired: 6 in, 2 out]
            }
            frame "3" {
              w1611 = "%Y-%m-%d " ("time format string (%c)")
              n411 = Format Date/Time String(time format string (%c)=w1611, seconds (now)=w1610) -> (date/time string=w1607:string)  [unwired: 1 in]
              n412 = Format Date/Time String(time format string (%c)=w1611, seconds (now)=w1609) -> (date/time string=w1608:string)  [unwired: 1 in]
              n413 = Format Into String(format string="Select DATE,Production_Count,Station_ID,Stack_holder_ID\nfrom Production_COUNT\nWhere DATE between '%s' and '%s' and Shift_ID='%s'and Stack_holder_ID='%d'\nand Station_ID='%d'" ("string"), w1608, w1607, w1601, 4 ("input 4"), 1 ("input 4")) -> (resulting string=w1604:string)  [unwired: 2 in, 1 out]
              n414 = call "Execute query.vi"("String"=w1604, "connection reference"=w1606) -> ("Table"=w1603:string[][], "connection reference 2"=w1602:T1)  [unwired: 6 in, 2 out]
            }
          }
        }
        frame "Production" {
          n415 = case shown="\"ALL\"" w1618 {
            selector: w1618 -> [_ _ w1634 w1647 w1660]
            tunnel: w1617 -> [_ w1630 w1643 w1656 w1669]
            tunnel: w1616 -> [_ w1629 w1642 w1655 w1668]
            tunnel: w1615 -> [_ _ _ _ _]
            tunnel: [_ w1623 w1636 w1649 w1662] -> w1614
            tunnel: w1613 -> [w1619 w1626 w1639 w1652 w1665]
            tunnel: [w1619 w1622 w1635 w1648 w1661] -> w1612
            frame "False", Default {
            }
            frame "ALL" {
              w1631 = "%Y-%m-%d " ("time format string (%c)")
              n416 = Format Date/Time String(time format string (%c)=w1631, seconds (now)=w1629) -> (date/time string=w1628:string)  [unwired: 1 in]
              n417 = Format Date/Time String(time format string (%c)=w1631, seconds (now)=w1630) -> (date/time string=w1627:string)  [unwired: 1 in]
              n418 = Format Into String(format string="Select DATE,Production_Count,Station_ID,Stack_holder_ID\nfrom Production_COUNT\nWhere DATE between '%s' and '%s' and Stack_holder_ID='%d'\nand Station_ID='%d'" ("string"), w1628, w1627, 5 ("input 3"), 1 ("input 3")) -> (resulting string=w1624:string)  [unwired: 2 in, 1 out]
              n419 = call "Execute query.vi"("String"=w1624, "connection reference"=w1626) -> ("Table"=w1623:string[][], "connection reference 2"=w1622:T1)  [unwired: 6 in, 2 out]
            }
            frame "1" {
              w1644 = "%Y-%m-%d " ("time format string (%c)")
              n420 = Format Date/Time String(time format string (%c)=w1644, seconds (now)=w1643) -> (date/time string=w1640:string)  [unwired: 1 in]
              n421 = Format Date/Time String(time format string (%c)=w1644, seconds (now)=w1642) -> (date/time string=w1641:string)  [unwired: 1 in]
              n422 = Format Into String(format string="Select DATE,Production_Count,Station_ID,Stack_holder_ID\nfrom Production_COUNT\nWhere DATE between '%s' and '%s' and Shift_ID='%s'and Stack_holder_ID='%d'\nand Station_ID='%d'" ("string"), w1641, w1640, w1634, 5 ("input 4"), 1 ("input 4")) -> (resulting string=w1637:string)  [unwired: 2 in, 1 out]
              n423 = call "Execute query.vi"("String"=w1637, "connection reference"=w1639) -> ("Table"=w1636:string[][], "connection reference 2"=w1635:T1)  [unwired: 6 in, 2 out]
            }
            frame "2" {
              w1657 = "%Y-%m-%d " ("time format string (%c)")
              n424 = Format Date/Time String(time format string (%c)=w1657, seconds (now)=w1656) -> (date/time string=w1653:string)  [unwired: 1 in]
              n425 = Format Date/Time String(time format string (%c)=w1657, seconds (now)=w1655) -> (date/time string=w1654:string)  [unwired: 1 in]
              n426 = Format Into String(format string="Select DATE,Production_Count,Station_ID,Stack_holder_ID\nfrom Production_COUNT\nWhere DATE between '%s' and '%s' and Shift_ID='%s'and Stack_holder_ID='%d'\nand Station_ID='%d'" ("string"), w1654, w1653, w1647, 5 ("input 4"), 1 ("input 4")) -> (resulting string=w1650:string)  [unwired: 2 in, 1 out]
              n427 = call "Execute query.vi"("String"=w1650, "connection reference"=w1652) -> ("Table"=w1649:string[][], "connection reference 2"=w1648:T1)  [unwired: 6 in, 2 out]
            }
            frame "3" {
              w1670 = "%Y-%m-%d " ("time format string (%c)")
              n428 = Format Date/Time String(time format string (%c)=w1670, seconds (now)=w1669) -> (date/time string=w1666:string)  [unwired: 1 in]
              n429 = Format Date/Time String(time format string (%c)=w1670, seconds (now)=w1668) -> (date/time string=w1667:string)  [unwired: 1 in]
              n430 = Format Into String(format string="Select DATE,Production_Count,Station_ID,Stack_holder_ID\nfrom Production_COUNT\nWhere DATE between '%s' and '%s' and Shift_ID='%s'and Stack_holder_ID='%d'\nand Station_ID='%d'" ("string"), w1667, w1666, w1660, 5 ("input 4"), 1 ("input 4")) -> (resulting string=w1663:string)  [unwired: 2 in, 1 out]
              n431 = call "Execute query.vi"("String"=w1663, "connection reference"=w1665) -> ("Table"=w1662:string[][], "connection reference 2"=w1661:T1)  [unwired: 6 in, 2 out]
            }
          }
        }
      }
    }
    frame "ST 4" {
      n432 = case shown="\"ALL\", Default" w1677 {
        tunnel: w1683 -> [w1695 w1796 w1855 w1911 w1970 w2029]
        tunnel: w1682 -> [w1694 w1795 w1854 w1910 w1969 w2028]
        tunnel: w1681 -> [w1693 w1794 w1853 w1909 w1968 w2027]
        tunnel: w1680 -> [w1692 w1793 w1852 w1908 w1967 w2026]
        tunnel: [w1691 w1792 w1851 w1907 w1966 w2025] -> w1674
        tunnel: w1679 -> [w1690 w1791 w1850 w1906 w1965 w2024]
        tunnel: [w1689 w1790 w1849 w1905 w1964 w2023] -> w1678
        tunnel: w1676 -> [w1688 _ _ _ _ _]
        tunnel: w1675 -> [w1687 _ _ _ _ _]
        tunnel: w1673 -> [w1686 _ _ _ _ _]
        tunnel: [w1685 _ _ _ _ _] -> w1672
        tunnel: w1671 -> [w1684 _ _ _ _ _]
        frame "ALL", Default {
          n433 = case shown="\"ALL\", Default" w1695 {
            selector: w1695 -> [_ w1720 w1744 w1768]
            tunnel: w1694 -> [_ _ _ _]
            tunnel: w1693 -> [_ _ _ _]
            tunnel: w1692 -> [_ _ _ _]
            tunnel: [w1698 w1721 w1745 w1769] -> w1691
            tunnel: w1690 -> [w1703 w1726 w1750 w1774]
            tunnel: [w1702 w1725 w1749 w1773] -> w1689
            tunnel: w1688 -> [w1701 w1724 w1748 w1772]
            tunnel: w1687 -> [_ _ _ _]
            tunnel: w1686 -> [w1700 w1723 w1747 w1771]
            tunnel: [w1697 w1719 w1743 w1767] -> w1685
            tunnel: w1684 -> [w1696 w1718 w1742 w1766]
            frame "ALL", Default {
              n434 = for {
                tunnel: w1701 -> [w1713]
                shift-right: [w1715] -> w1702
                shift-left: w1703 -> [w1717]
                tunnel: w1700 -> [w1709] mode=indexing
                shift-right: [w1706] -> w1698
                shift-left: string[][] [] -> [w1708]
                tunnel: [w1704] -> w1697
                tunnel: w1696 -> [w1705]
                n435 = Concatenate Strings("Select DISTINCT PLAN_DATE,PRODUCTION_COUNT,STATION_ID from  ", w1709, " Where year(PLAN_DATE) ='%s' and STATION_ID='%d'\n") -> (w1710:string)
                n436 = Format Into String(format string=w1710, w1713, 4 ("input 3")) -> (resulting string=w1716:string)  [unwired: 2 in, 1 out]
                n437 = call "Execute query.vi"("error in (no error)"=w1705, "String"=w1716, "connection reference"=w1717) -> ("error out"=w1704:errorcluster, "Table"=w1707:string[][], "connection reference 2"=w1715:T1)  [unwired: 5 in, 1 out]
                n438 = Build Array (concatenate)(w1708, w1707) -> (w1706:string[][])
              }
            }
            frame "1" {
              n439 = for {
                tunnel: w1724 -> [w1737]
                shift-right: [w1739] -> w1725
                shift-left: w1726 -> [w1741]
                tunnel: w1723 -> [w1733] mode=indexing
                shift-right: [w1730] -> w1721
                shift-left: string[][] [] -> [w1732]
                tunnel: w1720 -> [w1729]
                tunnel: [w1727] -> w1719
                tunnel: w1718 -> [w1728]
                n440 = Concatenate Strings("Select DISTINCT PLAN_DATE,PRODUCTION_COUNT,STATION_ID from  ", w1733, " Where year(PLAN_DATE) ='%s' and STATION_ID='%d' and  SHIFT='%s'\n") -> (w1734:string)
                n441 = Format Into String(format string=w1734, w1737, 4 ("input 3"), w1729) -> (resulting string=w1740:string)  [unwired: 2 in, 1 out]
                n442 = call "Execute query.vi"("error in (no error)"=w1728, "String"=w1740, "connection reference"=w1741) -> ("error out"=w1727:errorcluster, "Table"=w1731:string[][], "connection reference 2"=w1739:T1)  [unwired: 5 in, 1 out]
                n443 = Build Array (concatenate)(w1732, w1731) -> (w1730:string[][])
              }
            }
            frame "2" {
              n444 = for {
                tunnel: w1748 -> [w1761]
                shift-right: [w1763] -> w1749
                shift-left: w1750 -> [w1765]
                tunnel: w1747 -> [w1757] mode=indexing
                shift-right: [w1754] -> w1745
                shift-left: string[][] [] -> [w1756]
                tunnel: w1744 -> [w1753]
                tunnel: [w1751] -> w1743
                tunnel: w1742 -> [w1752]
                n445 = Concatenate Strings("Select DISTINCT PLAN_DATE,PRODUCTION_COUNT,STATION_ID from  ", w1757, " Where year(PLAN_DATE) ='%s' and STATION_ID='%d' and SHIFT='%s'\n") -> (w1758:string)
                n446 = Format Into String(format string=w1758, w1761, 4 ("input 3"), w1753) -> (resulting string=w1764:string)  [unwired: 2 in, 1 out]
                n447 = call "Execute query.vi"("error in (no error)"=w1752, "String"=w1764, "connection reference"=w1765) -> ("error out"=w1751:errorcluster, "Table"=w1755:string[][], "connection reference 2"=w1763:T1)  [unwired: 5 in, 1 out]
                n448 = Build Array (concatenate)(w1756, w1755) -> (w1754:string[][])
              }
            }
            frame "3" {
              n449 = for {
                tunnel: w1772 -> [w1785]
                shift-right: [w1787] -> w1773
                shift-left: w1774 -> [w1789]
                tunnel: w1771 -> [w1781] mode=indexing
                shift-right: [w1778] -> w1769
                shift-left: string[][] [] -> [w1780]
                tunnel: w1768 -> [w1777]
                tunnel: [w1775] -> w1767
                tunnel: w1766 -> [w1776]
                n450 = Concatenate Strings("Select DISTINCT PLAN_DATE,PRODUCTION_COUNT,STATION_ID from  ", w1781, " Where year(PLAN_DATE) ='%s' and STATION_ID='%d' and  SHIFT='%s'\n") -> (w1782:string)
                n451 = Format Into String(format string=w1782, w1785, 4 ("input 3"), w1777) -> (resulting string=w1788:string)  [unwired: 2 in, 1 out]
                n452 = call "Execute query.vi"("error in (no error)"=w1776, "String"=w1788, "connection reference"=w1789) -> ("error out"=w1775:errorcluster, "Table"=w1779:string[][], "connection reference 2"=w1787:T1)  [unwired: 5 in, 1 out]
                n453 = Build Array (concatenate)(w1780, w1779) -> (w1778:string[][])
              }
            }
          }
        }
        frame "Logistics" {
          n454 = case shown="\"ALL\"" w1796 {
            selector: w1796 -> [_ _ w1812 w1825 w1838]
            tunnel: w1795 -> [_ w1808 w1821 w1834 w1847]
            tunnel: w1794 -> [_ w1807 w1820 w1833 w1846]
            tunnel: w1793 -> [_ _ _ _ _]
            tunnel: [_ w1801 w1814 w1827 w1840] -> w1792
            tunnel: w1791 -> [w1797 w1804 w1817 w1830 w1843]
            tunnel: [w1797 w1800 w1813 w1826 w1839] -> w1790
            frame "False", Default {
            }
            frame "ALL" {
              w1809 = "%Y-%m-%d " ("time format string (%c)")
              n455 = Format Date/Time String(time format string (%c)=w1809, seconds (now)=w1807) -> (date/time string=w1806:string)  [unwired: 1 in]
              n456 = Format Date/Time String(time format string (%c)=w1809, seconds (now)=w1808) -> (date/time string=w1805:string)  [unwired: 1 in]
              n457 = Format Into String(format string="Select DATE,Production_Count,Station_ID,Stack_holder_ID\nfrom Production_COUNT\nWhere DATE between '%s' and '%s' and Stack_holder_ID='%d'\nand Station_ID='%d'" ("string"), w1806, w1805, 2 ("input 3"), 1 ("input 4")) -> (resulting string=w1802:string)  [unwired: 2 in, 1 out]
              n458 = call "Execute query.vi"("String"=w1802, "connection reference"=w1804) -> ("Table"=w1801:string[][], "connection reference 2"=w1800:T1)  [unwired: 6 in, 2 out]
            }
            frame "1" {
              w1822 = "%Y-%m-%d " ("time format string (%c)")
              n459 = Format Date/Time String(time format string (%c)=w1822, seconds (now)=w1821) -> (date/time string=w1818:string)  [unwired: 1 in]
              n460 = Format Date/Time String(time format string (%c)=w1822, seconds (now)=w1820) -> (date/time string=w1819:string)  [unwired: 1 in]
              n461 = Format Into String(format string="Select DATE,Production_Count,Station_ID,Stack_holder_ID\nfrom Production_COUNT\nWhere DATE between '%s' and '%s' and Shift_ID='%s'and Stack_holder_ID='%d'\nand Station_ID='%d'" ("string"), w1819, w1818, w1812, 2 ("input 4"), 1 ("input 4")) -> (resulting string=w1815:string)  [unwired: 2 in, 1 out]
              n462 = call "Execute query.vi"("String"=w1815, "connection reference"=w1817) -> ("Table"=w1814:string[][], "connection reference 2"=w1813:T1)  [unwired: 6 in, 2 out]
            }
            frame "2" {
              w1835 = "%Y-%m-%d " ("time format string (%c)")
              n463 = Format Date/Time String(time format string (%c)=w1835, seconds (now)=w1834) -> (date/time string=w1831:string)  [unwired: 1 in]
              n464 = Format Date/Time String(time format string (%c)=w1835, seconds (now)=w1833) -> (date/time string=w1832:string)  [unwired: 1 in]
              n465 = Format Into String(format string="Select DATE,Production_Count,Station_ID,Stack_holder_ID\nfrom Production_COUNT\nWhere DATE between '%s' and '%s' and Shift_ID='%s'and Stack_holder_ID='%d'\nand Station_ID='%d'" ("string"), w1832, w1831, w1825, 2 ("input 4"), 1 ("input 4")) -> (resulting string=w1828:string)  [unwired: 2 in, 1 out]
              n466 = call "Execute query.vi"("String"=w1828, "connection reference"=w1830) -> ("Table"=w1827:string[][], "connection reference 2"=w1826:T1)  [unwired: 6 in, 2 out]
            }
            frame "3" {
              w1848 = "%Y-%m-%d " ("time format string (%c)")
              n467 = Format Date/Time String(time format string (%c)=w1848, seconds (now)=w1847) -> (date/time string=w1844:string)  [unwired: 1 in]
              n468 = Format Date/Time String(time format string (%c)=w1848, seconds (now)=w1846) -> (date/time string=w1845:string)  [unwired: 1 in]
              n469 = Format Into String(format string="Select DATE,Production_Count,Station_ID,Stack_holder_ID\nfrom Production_COUNT\nWhere DATE between '%s' and '%s' and Shift_ID='%s'and Stack_holder_ID='%d'\nand Station_ID='%d'" ("string"), w1845, w1844, w1838, 2 ("input 4"), 1 ("input 4")) -> (resulting string=w1841:string)  [unwired: 2 in, 1 out]
              n470 = call "Execute query.vi"("String"=w1841, "connection reference"=w1843) -> ("Table"=w1840:string[][], "connection reference 2"=w1839:T1)  [unwired: 6 in, 2 out]
            }
          }
        }
        frame "Gap Leader" {
          n471 = case shown="\"3\"" w1855 {
            selector: w1855 -> [_ _ w1870 w1882 w1894]
            tunnel: w1854 -> [_ w1867 w1879 w1891 w1903]
            tunnel: w1853 -> [_ w1866 w1878 w1890 w1902]
            tunnel: w1852 -> [_ _ _ _ _]
            tunnel: [_ w1860 w1872 w1884 w1896] -> w1851
            tunnel: w1850 -> [w1856 w1863 w1875 w1887 w1899]
            tunnel: [w1856 w1859 w1871 w1883 w1895] -> w1849
            frame "False", Default {
            }
            frame "ALL" {
              w1868 = "%Y-%m-%d " ("time format string (%c)")
              n472 = Format Date/Time String(time format string (%c)=w1868, seconds (now)=w1866) -> (date/time string=w1865:string)  [unwired: 1 in]
              n473 = Format Date/Time String(time format string (%c)=w1868, seconds (now)=w1867) -> (date/time string=w1864:string)  [unwired: 1 in]
              n474 = Format Into String(format string="Select DATE,Production_Count,Station_ID,Stack_holder_ID\nfrom Production_COUNT\nWhere DATE between '%s' and '%s' and Stack_holder_ID='%d'\nand Station_ID='%d'" ("string"), w1865, w1864, 1 ("input 3"), 1 ("input 3")) -> (resulting string=w1861:string)  [unwired: 2 in, 1 out]
              n475 = call "Execute query.vi"("String"=w1861, "connection reference"=w1863) -> ("Table"=w1860:string[][], "connection reference 2"=w1859:T1)  [unwired: 6 in, 2 out]
            }
            frame "1" {
              w1869 = 1 ("input 4")
              w1880 = "%Y-%m-%d " ("time format string (%c)")
              n476 = Format Date/Time String(time format string (%c)=w1880, seconds (now)=w1879) -> (date/time string=w1876:string)  [unwired: 1 in]
              n477 = Format Date/Time String(time format string (%c)=w1880, seconds (now)=w1878) -> (date/time string=w1877:string)  [unwired: 1 in]
              n478 = Format Into String(format string="Select DATE,Production_Count,Station_ID,Stack_holder_ID\nfrom Production_COUNT\nWhere DATE between '%s' and '%s' and Shift_ID='%s'and Stack_holder_ID='%d'\nand Station_ID='%d'" ("string"), w1877, w1876, w1870, w1869, w1869) -> (resulting string=w1873:string)  [unwired: 2 in, 1 out]
              n479 = call "Execute query.vi"("String"=w1873, "connection reference"=w1875) -> ("Table"=w1872:string[][], "connection reference 2"=w1871:T1)  [unwired: 6 in, 2 out]
            }
            frame "2" {
              w1881 = 1 ("input 4")
              w1892 = "%Y-%m-%d " ("time format string (%c)")
              n480 = Format Date/Time String(time format string (%c)=w1892, seconds (now)=w1891) -> (date/time string=w1888:string)  [unwired: 1 in]
              n481 = Format Date/Time String(time format string (%c)=w1892, seconds (now)=w1890) -> (date/time string=w1889:string)  [unwired: 1 in]
              n482 = Format Into String(format string="Select DATE,Production_Count,Station_ID,Stack_holder_ID\nfrom Production_COUNT\nWhere DATE between '%s' and '%s' and Shift_ID='%s'and Stack_holder_ID='%d'\nand Station_ID='%d'" ("string"), w1889, w1888, w1882, w1881, w1881) -> (resulting string=w1885:string)  [unwired: 2 in, 1 out]
              n483 = call "Execute query.vi"("String"=w1885, "connection reference"=w1887) -> ("Table"=w1884:string[][], "connection reference 2"=w1883:T1)  [unwired: 6 in, 2 out]
            }
            frame "3" {
              w1893 = 1 ("input 4")
              w1904 = "%Y-%m-%d " ("time format string (%c)")
              n484 = Format Date/Time String(time format string (%c)=w1904, seconds (now)=w1903) -> (date/time string=w1900:string)  [unwired: 1 in]
              n485 = Format Date/Time String(time format string (%c)=w1904, seconds (now)=w1902) -> (date/time string=w1901:string)  [unwired: 1 in]
              n486 = Format Into String(format string="Select DATE,Production_Count,Station_ID,Stack_holder_ID\nfrom Production_COUNT\nWhere DATE between '%s' and '%s' and Shift_ID='%s'and Stack_holder_ID='%d'\nand Station_ID='%d'" ("string"), w1901, w1900, w1894, w1893, w1893) -> (resulting string=w1897:string)  [unwired: 2 in, 1 out]
              n487 = call "Execute query.vi"("String"=w1897, "connection reference"=w1899) -> ("Table"=w1896:string[][], "connection reference 2"=w1895:T1)  [unwired: 6 in, 2 out]
            }
          }
        }
        frame "Maintenance" {
          n488 = case shown="\"ALL\"" w1911 {
            selector: w1911 -> [_ _ w1927 w1940 w1953]
            tunnel: w1910 -> [_ w1923 w1936 w1949 w1962]
            tunnel: w1909 -> [_ w1922 w1935 w1948 w1961]
            tunnel: w1908 -> [_ _ _ _ _]
            tunnel: [_ w1916 w1929 w1942 w1955] -> w1907
            tunnel: w1906 -> [w1912 w1919 w1932 w1945 w1958]
            tunnel: [w1912 w1915 w1928 w1941 w1954] -> w1905
            frame "False", Default {
            }
            frame "ALL" {
              w1924 = "%Y-%m-%d " ("time format string (%c)")
              n489 = Format Date/Time String(time format string (%c)=w1924, seconds (now)=w1922) -> (date/time string=w1921:string)  [unwired: 1 in]
              n490 = Format Date/Time String(time format string (%c)=w1924, seconds (now)=w1923) -> (date/time string=w1920:string)  [unwired: 1 in]
              n491 = Format Into String(format string="Select DATE,Production_Count,Station_ID,Stack_holder_ID\nfrom Production_COUNT\nWhere DATE between '%s' and '%s' and Stack_holder_ID='%d'\nand Station_ID='%d'" ("string"), w1921, w1920, 3 ("input 3"), 1 ("input 4")) -> (resulting string=w1917:string)  [unwired: 2 in, 1 out]
              n492 = call "Execute query.vi"("String"=w1917, "connection reference"=w1919) -> ("Table"=w1916:string[][], "connection reference 2"=w1915:T1)  [unwired: 6 in, 2 out]
            }
            frame "1" {
              w1937 = "%Y-%m-%d " ("time format string (%c)")
              n493 = Format Date/Time String(time format string (%c)=w1937, seconds (now)=w1936) -> (date/time string=w1933:string)  [unwired: 1 in]
              n494 = Format Date/Time String(time format string (%c)=w1937, seconds (now)=w1935) -> (date/time string=w1934:string)  [unwired: 1 in]
              n495 = Format Into String(format string="Select DATE,Production_Count,Station_ID,Stack_holder_ID\nfrom Production_COUNT\nWhere DATE between '%s' and '%s' and Shift_ID='%s'and Stack_holder_ID='%d'\nand Station_ID='%d'" ("string"), w1934, w1933, w1927, 3 ("input 4"), 1 ("input 5")) -> (resulting string=w1930:string)  [unwired: 2 in, 1 out]
              n496 = call "Execute query.vi"("String"=w1930, "connection reference"=w1932) -> ("Table"=w1929:string[][], "connection reference 2"=w1928:T1)  [unwired: 6 in, 2 out]
            }
            frame "2" {
              w1950 = "%Y-%m-%d " ("time format string (%c)")
              n497 = Format Date/Time String(time format string (%c)=w1950, seconds (now)=w1949) -> (date/time string=w1946:string)  [unwired: 1 in]
              n498 = Format Date/Time String(time format string (%c)=w1950, seconds (now)=w1948) -> (date/time string=w1947:string)  [unwired: 1 in]
              n499 = Format Into String(format string="Select DATE,Production_Count,Station_ID,Stack_holder_ID\nfrom Production_COUNT\nWhere DATE between '%s' and '%s' and Shift_ID='%s'and Stack_holder_ID='%d'\nand Station_ID='%d'" ("string"), w1947, w1946, w1940, 3 ("input 4"), 1 ("input 5")) -> (resulting string=w1943:string)  [unwired: 2 in, 1 out]
              n500 = call "Execute query.vi"("String"=w1943, "connection reference"=w1945) -> ("Table"=w1942:string[][], "connection reference 2"=w1941:T1)  [unwired: 6 in, 2 out]
            }
            frame "3" {
              w1963 = "%Y-%m-%d " ("time format string (%c)")
              n501 = Format Date/Time String(time format string (%c)=w1963, seconds (now)=w1962) -> (date/time string=w1959:string)  [unwired: 1 in]
              n502 = Format Date/Time String(time format string (%c)=w1963, seconds (now)=w1961) -> (date/time string=w1960:string)  [unwired: 1 in]
              n503 = Format Into String(format string="Select DATE,Production_Count,Station_ID,Stack_holder_ID\nfrom Production_COUNT\nWhere DATE between '%s' and '%s' and Shift_ID='%s'and Stack_holder_ID='%d'\nand Station_ID='%d'" ("string"), w1960, w1959, w1953, 3 ("input 4"), 1 ("input 5")) -> (resulting string=w1956:string)  [unwired: 2 in, 1 out]
              n504 = call "Execute query.vi"("String"=w1956, "connection reference"=w1958) -> ("Table"=w1955:string[][], "connection reference 2"=w1954:T1)  [unwired: 6 in, 2 out]
            }
          }
        }
        frame "Quality" {
          n505 = case shown="\"ALL\"" w1970 {
            selector: w1970 -> [_ _ w1986 w1999 w2012]
            tunnel: w1969 -> [_ w1982 w1995 w2008 w2021]
            tunnel: w1968 -> [_ w1981 w1994 w2007 w2020]
            tunnel: w1967 -> [_ _ _ _ _]
            tunnel: [_ w1975 w1988 w2001 w2014] -> w1966
            tunnel: w1965 -> [w1971 w1978 w1991 w2004 w2017]
            tunnel: [w1971 w1974 w1987 w2000 w2013] -> w1964
            frame "False", Default {
            }
            frame "ALL" {
              w1983 = "%Y-%m-%d " ("time format string (%c)")
              n506 = Format Date/Time String(time format string (%c)=w1983, seconds (now)=w1981) -> (date/time string=w1980:string)  [unwired: 1 in]
              n507 = Format Date/Time String(time format string (%c)=w1983, seconds (now)=w1982) -> (date/time string=w1979:string)  [unwired: 1 in]
              n508 = Format Into String(format string="Select DATE,Production_Count,Station_ID,Stack_holder_ID\nfrom Production_COUNT\nWhere DATE between '%s' and '%s' and Stack_holder_ID='%d'\nand Station_ID='%d'" ("string"), w1980, w1979, 4 ("input 3"), 1 ("input 3")) -> (resulting string=w1976:string)  [unwired: 2 in, 1 out]
              n509 = call "Execute query.vi"("String"=w1976, "connection reference"=w1978) -> ("Table"=w1975:string[][], "connection reference 2"=w1974:T1)  [unwired: 6 in, 2 out]
            }
            frame "1" {
              w1996 = "%Y-%m-%d " ("time format string (%c)")
              n510 = Format Date/Time String(time format string (%c)=w1996, seconds (now)=w1995) -> (date/time string=w1992:string)  [unwired: 1 in]
              n511 = Format Date/Time String(time format string (%c)=w1996, seconds (now)=w1994) -> (date/time string=w1993:string)  [unwired: 1 in]
              n512 = Format Into String(format string="Select DATE,Production_Count,Station_ID,Stack_holder_ID\nfrom Production_COUNT\nWhere DATE between '%s' and '%s' and Shift_ID='%s'and Stack_holder_ID='%d'\nand Station_ID='%d'" ("string"), w1993, w1992, w1986, 4 ("input 4"), 1 ("input 4")) -> (resulting string=w1989:string)  [unwired: 2 in, 1 out]
              n513 = call "Execute query.vi"("String"=w1989, "connection reference"=w1991) -> ("Table"=w1988:string[][], "connection reference 2"=w1987:T1)  [unwired: 6 in, 2 out]
            }
            frame "2" {
              w2009 = "%Y-%m-%d " ("time format string (%c)")
              n514 = Format Date/Time String(time format string (%c)=w2009, seconds (now)=w2008) -> (date/time string=w2005:string)  [unwired: 1 in]
              n515 = Format Date/Time String(time format string (%c)=w2009, seconds (now)=w2007) -> (date/time string=w2006:string)  [unwired: 1 in]
              n516 = Format Into String(format string="Select DATE,Production_Count,Station_ID,Stack_holder_ID\nfrom Production_COUNT\nWhere DATE between '%s' and '%s' and Shift_ID='%s'and Stack_holder_ID='%d'\nand Station_ID='%d'" ("string"), w2006, w2005, w1999, 4 ("input 4"), 1 ("input 4")) -> (resulting string=w2002:string)  [unwired: 2 in, 1 out]
              n517 = call "Execute query.vi"("String"=w2002, "connection reference"=w2004) -> ("Table"=w2001:string[][], "connection reference 2"=w2000:T1)  [unwired: 6 in, 2 out]
            }
            frame "3" {
              w2022 = "%Y-%m-%d " ("time format string (%c)")
              n518 = Format Date/Time String(time format string (%c)=w2022, seconds (now)=w2021) -> (date/time string=w2018:string)  [unwired: 1 in]
              n519 = Format Date/Time String(time format string (%c)=w2022, seconds (now)=w2020) -> (date/time string=w2019:string)  [unwired: 1 in]
              n520 = Format Into String(format string="Select DATE,Production_Count,Station_ID,Stack_holder_ID\nfrom Production_COUNT\nWhere DATE between '%s' and '%s' and Shift_ID='%s'and Stack_holder_ID='%d'\nand Station_ID='%d'" ("string"), w2019, w2018, w2012, 4 ("input 4"), 1 ("input 4")) -> (resulting string=w2015:string)  [unwired: 2 in, 1 out]
              n521 = call "Execute query.vi"("String"=w2015, "connection reference"=w2017) -> ("Table"=w2014:string[][], "connection reference 2"=w2013:T1)  [unwired: 6 in, 2 out]
            }
          }
        }
        frame "Production" {
          n522 = case shown="\"ALL\"" w2029 {
            selector: w2029 -> [_ _ w2045 w2058 w2071]
            tunnel: w2028 -> [_ w2041 w2054 w2067 w2080]
            tunnel: w2027 -> [_ w2040 w2053 w2066 w2079]
            tunnel: w2026 -> [_ _ _ _ _]
            tunnel: [_ w2034 w2047 w2060 w2073] -> w2025
            tunnel: w2024 -> [w2030 w2037 w2050 w2063 w2076]
            tunnel: [w2030 w2033 w2046 w2059 w2072] -> w2023
            frame "False", Default {
            }
            frame "ALL" {
              w2042 = "%Y-%m-%d " ("time format string (%c)")
              n523 = Format Date/Time String(time format string (%c)=w2042, seconds (now)=w2040) -> (date/time string=w2039:string)  [unwired: 1 in]
              n524 = Format Date/Time String(time format string (%c)=w2042, seconds (now)=w2041) -> (date/time string=w2038:string)  [unwired: 1 in]
              n525 = Format Into String(format string="Select DATE,Production_Count,Station_ID,Stack_holder_ID\nfrom Production_COUNT\nWhere DATE between '%s' and '%s' and Stack_holder_ID='%d'\nand Station_ID='%d'" ("string"), w2039, w2038, 5 ("input 3"), 1 ("input 3")) -> (resulting string=w2035:string)  [unwired: 2 in, 1 out]
              n526 = call "Execute query.vi"("String"=w2035, "connection reference"=w2037) -> ("Table"=w2034:string[][], "connection reference 2"=w2033:T1)  [unwired: 6 in, 2 out]
            }
            frame "1" {
              w2055 = "%Y-%m-%d " ("time format string (%c)")
              n527 = Format Date/Time String(time format string (%c)=w2055, seconds (now)=w2054) -> (date/time string=w2051:string)  [unwired: 1 in]
              n528 = Format Date/Time String(time format string (%c)=w2055, seconds (now)=w2053) -> (date/time string=w2052:string)  [unwired: 1 in]
              n529 = Format Into String(format string="Select DATE,Production_Count,Station_ID,Stack_holder_ID\nfrom Production_COUNT\nWhere DATE between '%s' and '%s' and Shift_ID='%s'and Stack_holder_ID='%d'\nand Station_ID='%d'" ("string"), w2052, w2051, w2045, 5 ("input 4"), 1 ("input 4")) -> (resulting string=w2048:string)  [unwired: 2 in, 1 out]
              n530 = call "Execute query.vi"("String"=w2048, "connection reference"=w2050) -> ("Table"=w2047:string[][], "connection reference 2"=w2046:T1)  [unwired: 6 in, 2 out]
            }
            frame "2" {
              w2068 = "%Y-%m-%d " ("time format string (%c)")
              n531 = Format Date/Time String(time format string (%c)=w2068, seconds (now)=w2067) -> (date/time string=w2064:string)  [unwired: 1 in]
              n532 = Format Date/Time String(time format string (%c)=w2068, seconds (now)=w2066) -> (date/time string=w2065:string)  [unwired: 1 in]
              n533 = Format Into String(format string="Select DATE,Production_Count,Station_ID,Stack_holder_ID\nfrom Production_COUNT\nWhere DATE between '%s' and '%s' and Shift_ID='%s'and Stack_holder_ID='%d'\nand Station_ID='%d'" ("string"), w2065, w2064, w2058, 5 ("input 4"), 1 ("input 4")) -> (resulting string=w2061:string)  [unwired: 2 in, 1 out]
              n534 = call "Execute query.vi"("String"=w2061, "connection reference"=w2063) -> ("Table"=w2060:string[][], "connection reference 2"=w2059:T1)  [unwired: 6 in, 2 out]
            }
            frame "3" {
              w2081 = "%Y-%m-%d " ("time format string (%c)")
              n535 = Format Date/Time String(time format string (%c)=w2081, seconds (now)=w2080) -> (date/time string=w2077:string)  [unwired: 1 in]
              n536 = Format Date/Time String(time format string (%c)=w2081, seconds (now)=w2079) -> (date/time string=w2078:string)  [unwired: 1 in]
              n537 = Format Into String(format string="Select DATE,Production_Count,Station_ID,Stack_holder_ID\nfrom Production_COUNT\nWhere DATE between '%s' and '%s' and Shift_ID='%s'and Stack_holder_ID='%d'\nand Station_ID='%d'" ("string"), w2078, w2077, w2071, 5 ("input 4"), 1 ("input 4")) -> (resulting string=w2074:string)  [unwired: 2 in, 1 out]
              n538 = call "Execute query.vi"("String"=w2074, "connection reference"=w2076) -> ("Table"=w2073:string[][], "connection reference 2"=w2072:T1)  [unwired: 6 in, 2 out]
            }
          }
        }
      }
    }
    frame "ST 5" {
      n539 = case shown="\"ALL\", Default" w2088 {
        tunnel: w2094 -> [w2106 w2207 w2266 w2322 w2381 w2440]
        tunnel: w2093 -> [w2105 w2206 w2265 w2321 w2380 w2439]
        tunnel: w2092 -> [w2104 w2205 w2264 w2320 w2379 w2438]
        tunnel: w2091 -> [w2103 w2204 w2263 w2319 w2378 w2437]
        tunnel: [w2102 w2203 w2262 w2318 w2377 w2436] -> w2085
        tunnel: w2090 -> [w2101 w2202 w2261 w2317 w2376 w2435]
        tunnel: [w2100 w2201 w2260 w2316 w2375 w2434] -> w2089
        tunnel: w2087 -> [w2099 _ _ _ _ _]
        tunnel: w2086 -> [w2098 _ _ _ _ _]
        tunnel: w2084 -> [w2097 _ _ _ _ _]
        tunnel: [w2096 _ _ _ _ _] -> w2083
        tunnel: w2082 -> [w2095 _ _ _ _ _]
        frame "ALL", Default {
          n540 = case shown="\"3\"" w2106 {
            selector: w2106 -> [_ w2131 w2155 w2179]
            tunnel: w2105 -> [_ _ _ _]
            tunnel: w2104 -> [_ _ _ _]
            tunnel: w2103 -> [_ _ _ _]
            tunnel: [w2109 w2132 w2156 w2180] -> w2102
            tunnel: w2101 -> [w2114 w2137 w2161 w2185]
            tunnel: [w2113 w2136 w2160 w2184] -> w2100
            tunnel: w2099 -> [w2112 w2135 w2159 w2183]
            tunnel: w2098 -> [_ _ _ _]
            tunnel: w2097 -> [w2111 w2134 w2158 w2182]
            tunnel: [w2108 w2130 w2154 w2178] -> w2096
            tunnel: w2095 -> [w2107 w2129 w2153 w2177]
            frame "ALL", Default {
              n541 = for {
                tunnel: w2112 -> [w2124]
                shift-right: [w2126] -> w2113
                shift-left: w2114 -> [w2128]
                tunnel: w2111 -> [w2120] mode=indexing
                shift-right: [w2117] -> w2109
                shift-left: string[][] [] -> [w2119]
                tunnel: [w2115] -> w2108
                tunnel: w2107 -> [w2116]
                n542 = Concatenate Strings("Select DISTINCT PLAN_DATE,PRODUCTION_COUNT,STATION_ID from  ", w2120, " Where year(PLAN_DATE) ='%s' and STATION_ID='%d'\n") -> (w2121:string)
                n543 = Format Into String(format string=w2121, w2124, 5 ("input 3")) -> (resulting string=w2127:string)  [unwired: 2 in, 1 out]
                n544 = call "Execute query.vi"("error in (no error)"=w2116, "String"=w2127, "connection reference"=w2128) -> ("error out"=w2115:errorcluster, "Table"=w2118:string[][], "connection reference 2"=w2126:T1)  [unwired: 5 in, 1 out]
                n545 = Build Array (concatenate)(w2119, w2118) -> (w2117:string[][])
              }
            }
            frame "1" {
              n546 = for {
                tunnel: w2135 -> [w2148]
                shift-right: [w2150] -> w2136
                shift-left: w2137 -> [w2152]
                tunnel: w2134 -> [w2144] mode=indexing
                shift-right: [w2141] -> w2132
                shift-left: string[][] [] -> [w2143]
                tunnel: w2131 -> [w2140]
                tunnel: [w2138] -> w2130
                tunnel: w2129 -> [w2139]
                n547 = Concatenate Strings("Select DISTINCT PLAN_DATE,PRODUCTION_COUNT,STATION_ID from  ", w2144, " Where year(PLAN_DATE) ='%s' and STATION_ID='%d' and  SHIFT='%s'\n") -> (w2145:string)
                n548 = Format Into String(format string=w2145, w2148, 5 ("input 3"), w2140) -> (resulting string=w2151:string)  [unwired: 2 in, 1 out]
                n549 = call "Execute query.vi"("error in (no error)"=w2139, "String"=w2151, "connection reference"=w2152) -> ("error out"=w2138:errorcluster, "Table"=w2142:string[][], "connection reference 2"=w2150:T1)  [unwired: 5 in, 1 out]
                n550 = Build Array (concatenate)(w2143, w2142) -> (w2141:string[][])
              }
            }
            frame "2" {
              n551 = for {
                tunnel: w2159 -> [w2172]
                shift-right: [w2174] -> w2160
                shift-left: w2161 -> [w2176]
                tunnel: w2158 -> [w2168] mode=indexing
                shift-right: [w2165] -> w2156
                shift-left: string[][] [] -> [w2167]
                tunnel: w2155 -> [w2164]
                tunnel: [w2162] -> w2154
                tunnel: w2153 -> [w2163]
                n552 = Concatenate Strings("Select DISTINCT PLAN_DATE,PRODUCTION_COUNT,STATION_ID from  ", w2168, " Where year(PLAN_DATE) ='%s' and STATION_ID='%d' and SHIFT='%s'\n") -> (w2169:string)
                n553 = Format Into String(format string=w2169, w2172, 5 ("input 3"), w2164) -> (resulting string=w2175:string)  [unwired: 2 in, 1 out]
                n554 = call "Execute query.vi"("error in (no error)"=w2163, "String"=w2175, "connection reference"=w2176) -> ("error out"=w2162:errorcluster, "Table"=w2166:string[][], "connection reference 2"=w2174:T1)  [unwired: 5 in, 1 out]
                n555 = Build Array (concatenate)(w2167, w2166) -> (w2165:string[][])
              }
            }
            frame "3" {
              n556 = for {
                tunnel: w2183 -> [w2196]
                shift-right: [w2198] -> w2184
                shift-left: w2185 -> [w2200]
                tunnel: w2182 -> [w2192] mode=indexing
                shift-right: [w2189] -> w2180
                shift-left: string[][] [] -> [w2191]
                tunnel: w2179 -> [w2188]
                tunnel: [w2186] -> w2178
                tunnel: w2177 -> [w2187]
                n557 = Concatenate Strings("Select DISTINCT PLAN_DATE,PRODUCTION_COUNT,STATION_ID from  ", w2192, " Where year(PLAN_DATE) ='%s' and STATION_ID='%d' and  SHIFT='%s'\n") -> (w2193:string)
                n558 = Format Into String(format string=w2193, w2196, 5 ("input 3"), w2188) -> (resulting string=w2199:string)  [unwired: 2 in, 1 out]
                n559 = call "Execute query.vi"("error in (no error)"=w2187, "String"=w2199, "connection reference"=w2200) -> ("error out"=w2186:errorcluster, "Table"=w2190:string[][], "connection reference 2"=w2198:T1)  [unwired: 5 in, 1 out]
                n560 = Build Array (concatenate)(w2191, w2190) -> (w2189:string[][])
              }
            }
          }
        }
        frame "Logistics" {
          n561 = case shown="\"ALL\"" w2207 {
            selector: w2207 -> [_ _ w2223 w2236 w2249]
            tunnel: w2206 -> [_ w2219 w2232 w2245 w2258]
            tunnel: w2205 -> [_ w2218 w2231 w2244 w2257]
            tunnel: w2204 -> [_ _ _ _ _]
            tunnel: [_ w2212 w2225 w2238 w2251] -> w2203
            tunnel: w2202 -> [w2208 w2215 w2228 w2241 w2254]
            tunnel: [w2208 w2211 w2224 w2237 w2250] -> w2201
            frame "False", Default {
            }
            frame "ALL" {
              w2220 = "%Y-%m-%d " ("time format string (%c)")
              n562 = Format Date/Time String(time format string (%c)=w2220, seconds (now)=w2218) -> (date/time string=w2217:string)  [unwired: 1 in]
              n563 = Format Date/Time String(time format string (%c)=w2220, seconds (now)=w2219) -> (date/time string=w2216:string)  [unwired: 1 in]
              n564 = Format Into String(format string="Select DATE,Production_Count,Station_ID,Stack_holder_ID\nfrom Production_COUNT\nWhere DATE between '%s' and '%s' and Stack_holder_ID='%d'\nand Station_ID='%d'" ("string"), w2217, w2216, 2 ("input 3"), 1 ("input 4")) -> (resulting string=w2213:string)  [unwired: 2 in, 1 out]
              n565 = call "Execute query.vi"("String"=w2213, "connection reference"=w2215) -> ("Table"=w2212:string[][], "connection reference 2"=w2211:T1)  [unwired: 6 in, 2 out]
            }
            frame "1" {
              w2233 = "%Y-%m-%d " ("time format string (%c)")
              n566 = Format Date/Time String(time format string (%c)=w2233, seconds (now)=w2232) -> (date/time string=w2229:string)  [unwired: 1 in]
              n567 = Format Date/Time String(time format string (%c)=w2233, seconds (now)=w2231) -> (date/time string=w2230:string)  [unwired: 1 in]
              n568 = Format Into String(format string="Select DATE,Production_Count,Station_ID,Stack_holder_ID\nfrom Production_COUNT\nWhere DATE between '%s' and '%s' and Shift_ID='%s'and Stack_holder_ID='%d'\nand Station_ID='%d'" ("string"), w2230, w2229, w2223, 2 ("input 4"), 1 ("input 4")) -> (resulting string=w2226:string)  [unwired: 2 in, 1 out]
              n569 = call "Execute query.vi"("String"=w2226, "connection reference"=w2228) -> ("Table"=w2225:string[][], "connection reference 2"=w2224:T1)  [unwired: 6 in, 2 out]
            }
            frame "2" {
              w2246 = "%Y-%m-%d " ("time format string (%c)")
              n570 = Format Date/Time String(time format string (%c)=w2246, seconds (now)=w2245) -> (date/time string=w2242:string)  [unwired: 1 in]
              n571 = Format Date/Time String(time format string (%c)=w2246, seconds (now)=w2244) -> (date/time string=w2243:string)  [unwired: 1 in]
              n572 = Format Into String(format string="Select DATE,Production_Count,Station_ID,Stack_holder_ID\nfrom Production_COUNT\nWhere DATE between '%s' and '%s' and Shift_ID='%s'and Stack_holder_ID='%d'\nand Station_ID='%d'" ("string"), w2243, w2242, w2236, 2 ("input 4"), 1 ("input 4")) -> (resulting string=w2239:string)  [unwired: 2 in, 1 out]
              n573 = call "Execute query.vi"("String"=w2239, "connection reference"=w2241) -> ("Table"=w2238:string[][], "connection reference 2"=w2237:T1)  [unwired: 6 in, 2 out]
            }
            frame "3" {
              w2259 = "%Y-%m-%d " ("time format string (%c)")
              n574 = Format Date/Time String(time format string (%c)=w2259, seconds (now)=w2258) -> (date/time string=w2255:string)  [unwired: 1 in]
              n575 = Format Date/Time String(time format string (%c)=w2259, seconds (now)=w2257) -> (date/time string=w2256:string)  [unwired: 1 in]
              n576 = Format Into String(format string="Select DATE,Production_Count,Station_ID,Stack_holder_ID\nfrom Production_COUNT\nWhere DATE between '%s' and '%s' and Shift_ID='%s'and Stack_holder_ID='%d'\nand Station_ID='%d'" ("string"), w2256, w2255, w2249, 2 ("input 4"), 1 ("input 4")) -> (resulting string=w2252:string)  [unwired: 2 in, 1 out]
              n577 = call "Execute query.vi"("String"=w2252, "connection reference"=w2254) -> ("Table"=w2251:string[][], "connection reference 2"=w2250:T1)  [unwired: 6 in, 2 out]
            }
          }
        }
        frame "Gap Leader" {
          n578 = case shown="\"3\"" w2266 {
            selector: w2266 -> [_ _ w2281 w2293 w2305]
            tunnel: w2265 -> [_ w2278 w2290 w2302 w2314]
            tunnel: w2264 -> [_ w2277 w2289 w2301 w2313]
            tunnel: w2263 -> [_ _ _ _ _]
            tunnel: [_ w2271 w2283 w2295 w2307] -> w2262
            tunnel: w2261 -> [w2267 w2274 w2286 w2298 w2310]
            tunnel: [w2267 w2270 w2282 w2294 w2306] -> w2260
            frame "False", Default {
            }
            frame "ALL" {
              w2279 = "%Y-%m-%d " ("time format string (%c)")
              n579 = Format Date/Time String(time format string (%c)=w2279, seconds (now)=w2277) -> (date/time string=w2276:string)  [unwired: 1 in]
              n580 = Format Date/Time String(time format string (%c)=w2279, seconds (now)=w2278) -> (date/time string=w2275:string)  [unwired: 1 in]
              n581 = Format Into String(format string="Select DATE,Production_Count,Station_ID,Stack_holder_ID\nfrom Production_COUNT\nWhere DATE between '%s' and '%s' and Stack_holder_ID='%d'\nand Station_ID='%d'" ("string"), w2276, w2275, 1 ("input 3"), 1 ("input 3")) -> (resulting string=w2272:string)  [unwired: 2 in, 1 out]
              n582 = call "Execute query.vi"("String"=w2272, "connection reference"=w2274) -> ("Table"=w2271:string[][], "connection reference 2"=w2270:T1)  [unwired: 6 in, 2 out]
            }
            frame "1" {
              w2280 = 1 ("input 4")
              w2291 = "%Y-%m-%d " ("time format string (%c)")
              n583 = Format Date/Time String(time format string (%c)=w2291, seconds (now)=w2290) -> (date/time string=w2287:string)  [unwired: 1 in]
              n584 = Format Date/Time String(time format string (%c)=w2291, seconds (now)=w2289) -> (date/time string=w2288:string)  [unwired: 1 in]
              n585 = Format Into String(format string="Select DATE,Production_Count,Station_ID,Stack_holder_ID\nfrom Production_COUNT\nWhere DATE between '%s' and '%s' and Shift_ID='%s'and Stack_holder_ID='%d'\nand Station_ID='%d'" ("string"), w2288, w2287, w2281, w2280, w2280) -> (resulting string=w2284:string)  [unwired: 2 in, 1 out]
              n586 = call "Execute query.vi"("String"=w2284, "connection reference"=w2286) -> ("Table"=w2283:string[][], "connection reference 2"=w2282:T1)  [unwired: 6 in, 2 out]
            }
            frame "2" {
              w2292 = 1 ("input 4")
              w2303 = "%Y-%m-%d " ("time format string (%c)")
              n587 = Format Date/Time String(time format string (%c)=w2303, seconds (now)=w2302) -> (date/time string=w2299:string)  [unwired: 1 in]
              n588 = Format Date/Time String(time format string (%c)=w2303, seconds (now)=w2301) -> (date/time string=w2300:string)  [unwired: 1 in]
              n589 = Format Into String(format string="Select DATE,Production_Count,Station_ID,Stack_holder_ID\nfrom Production_COUNT\nWhere DATE between '%s' and '%s' and Shift_ID='%s'and Stack_holder_ID='%d'\nand Station_ID='%d'" ("string"), w2300, w2299, w2293, w2292, w2292) -> (resulting string=w2296:string)  [unwired: 2 in, 1 out]
              n590 = call "Execute query.vi"("String"=w2296, "connection reference"=w2298) -> ("Table"=w2295:string[][], "connection reference 2"=w2294:T1)  [unwired: 6 in, 2 out]
            }
            frame "3" {
              w2304 = 1 ("input 4")
              w2315 = "%Y-%m-%d " ("time format string (%c)")
              n591 = Format Date/Time String(time format string (%c)=w2315, seconds (now)=w2314) -> (date/time string=w2311:string)  [unwired: 1 in]
              n592 = Format Date/Time String(time format string (%c)=w2315, seconds (now)=w2313) -> (date/time string=w2312:string)  [unwired: 1 in]
              n593 = Format Into String(format string="Select DATE,Production_Count,Station_ID,Stack_holder_ID\nfrom Production_COUNT\nWhere DATE between '%s' and '%s' and Shift_ID='%s'and Stack_holder_ID='%d'\nand Station_ID='%d'" ("string"), w2312, w2311, w2305, w2304, w2304) -> (resulting string=w2308:string)  [unwired: 2 in, 1 out]
              n594 = call "Execute query.vi"("String"=w2308, "connection reference"=w2310) -> ("Table"=w2307:string[][], "connection reference 2"=w2306:T1)  [unwired: 6 in, 2 out]
            }
          }
        }
        frame "Maintenance" {
          n595 = case shown="\"ALL\"" w2322 {
            selector: w2322 -> [_ _ w2338 w2351 w2364]
            tunnel: w2321 -> [_ w2334 w2347 w2360 w2373]
            tunnel: w2320 -> [_ w2333 w2346 w2359 w2372]
            tunnel: w2319 -> [_ _ _ _ _]
            tunnel: [_ w2327 w2340 w2353 w2366] -> w2318
            tunnel: w2317 -> [w2323 w2330 w2343 w2356 w2369]
            tunnel: [w2323 w2326 w2339 w2352 w2365] -> w2316
            frame "False", Default {
            }
            frame "ALL" {
              w2335 = "%Y-%m-%d " ("time format string (%c)")
              n596 = Format Date/Time String(time format string (%c)=w2335, seconds (now)=w2333) -> (date/time string=w2332:string)  [unwired: 1 in]
              n597 = Format Date/Time String(time format string (%c)=w2335, seconds (now)=w2334) -> (date/time string=w2331:string)  [unwired: 1 in]
              n598 = Format Into String(format string="Select DATE,Production_Count,Station_ID,Stack_holder_ID\nfrom Production_COUNT\nWhere DATE between '%s' and '%s' and Stack_holder_ID='%d'\nand Station_ID='%d'" ("string"), w2332, w2331, 3 ("input 3"), 1 ("input 4")) -> (resulting string=w2328:string)  [unwired: 2 in, 1 out]
              n599 = call "Execute query.vi"("String"=w2328, "connection reference"=w2330) -> ("Table"=w2327:string[][], "connection reference 2"=w2326:T1)  [unwired: 6 in, 2 out]
            }
            frame "1" {
              w2348 = "%Y-%m-%d " ("time format string (%c)")
              n600 = Format Date/Time String(time format string (%c)=w2348, seconds (now)=w2347) -> (date/time string=w2344:string)  [unwired: 1 in]
              n601 = Format Date/Time String(time format string (%c)=w2348, seconds (now)=w2346) -> (date/time string=w2345:string)  [unwired: 1 in]
              n602 = Format Into String(format string="Select DATE,Production_Count,Station_ID,Stack_holder_ID\nfrom Production_COUNT\nWhere DATE between '%s' and '%s' and Shift_ID='%s'and Stack_holder_ID='%d'\nand Station_ID='%d'" ("string"), w2345, w2344, w2338, 3 ("input 4"), 1 ("input 5")) -> (resulting string=w2341:string)  [unwired: 2 in, 1 out]
              n603 = call "Execute query.vi"("String"=w2341, "connection reference"=w2343) -> ("Table"=w2340:string[][], "connection reference 2"=w2339:T1)  [unwired: 6 in, 2 out]
            }
            frame "2" {
              w2361 = "%Y-%m-%d " ("time format string (%c)")
              n604 = Format Date/Time String(time format string (%c)=w2361, seconds (now)=w2360) -> (date/time string=w2357:string)  [unwired: 1 in]
              n605 = Format Date/Time String(time format string (%c)=w2361, seconds (now)=w2359) -> (date/time string=w2358:string)  [unwired: 1 in]
              n606 = Format Into String(format string="Select DATE,Production_Count,Station_ID,Stack_holder_ID\nfrom Production_COUNT\nWhere DATE between '%s' and '%s' and Shift_ID='%s'and Stack_holder_ID='%d'\nand Station_ID='%d'" ("string"), w2358, w2357, w2351, 3 ("input 4"), 1 ("input 5")) -> (resulting string=w2354:string)  [unwired: 2 in, 1 out]
              n607 = call "Execute query.vi"("String"=w2354, "connection reference"=w2356) -> ("Table"=w2353:string[][], "connection reference 2"=w2352:T1)  [unwired: 6 in, 2 out]
            }
            frame "3" {
              w2374 = "%Y-%m-%d " ("time format string (%c)")
              n608 = Format Date/Time String(time format string (%c)=w2374, seconds (now)=w2373) -> (date/time string=w2370:string)  [unwired: 1 in]
              n609 = Format Date/Time String(time format string (%c)=w2374, seconds (now)=w2372) -> (date/time string=w2371:string)  [unwired: 1 in]
              n610 = Format Into String(format string="Select DATE,Production_Count,Station_ID,Stack_holder_ID\nfrom Production_COUNT\nWhere DATE between '%s' and '%s' and Shift_ID='%s'and Stack_holder_ID='%d'\nand Station_ID='%d'" ("string"), w2371, w2370, w2364, 3 ("input 4"), 1 ("input 5")) -> (resulting string=w2367:string)  [unwired: 2 in, 1 out]
              n611 = call "Execute query.vi"("String"=w2367, "connection reference"=w2369) -> ("Table"=w2366:string[][], "connection reference 2"=w2365:T1)  [unwired: 6 in, 2 out]
            }
          }
        }
        frame "Quality" {
          n612 = case shown="\"ALL\"" w2381 {
            selector: w2381 -> [_ _ w2397 w2410 w2423]
            tunnel: w2380 -> [_ w2393 w2406 w2419 w2432]
            tunnel: w2379 -> [_ w2392 w2405 w2418 w2431]
            tunnel: w2378 -> [_ _ _ _ _]
            tunnel: [_ w2386 w2399 w2412 w2425] -> w2377
            tunnel: w2376 -> [w2382 w2389 w2402 w2415 w2428]
            tunnel: [w2382 w2385 w2398 w2411 w2424] -> w2375
            frame "False", Default {
            }
            frame "ALL" {
              w2394 = "%Y-%m-%d " ("time format string (%c)")
              n613 = Format Date/Time String(time format string (%c)=w2394, seconds (now)=w2392) -> (date/time string=w2391:string)  [unwired: 1 in]
              n614 = Format Date/Time String(time format string (%c)=w2394, seconds (now)=w2393) -> (date/time string=w2390:string)  [unwired: 1 in]
              n615 = Format Into String(format string="Select DATE,Production_Count,Station_ID,Stack_holder_ID\nfrom Production_COUNT\nWhere DATE between '%s' and '%s' and Stack_holder_ID='%d'\nand Station_ID='%d'" ("string"), w2391, w2390, 4 ("input 3"), 1 ("input 3")) -> (resulting string=w2387:string)  [unwired: 2 in, 1 out]
              n616 = call "Execute query.vi"("String"=w2387, "connection reference"=w2389) -> ("Table"=w2386:string[][], "connection reference 2"=w2385:T1)  [unwired: 6 in, 2 out]
            }
            frame "1" {
              w2407 = "%Y-%m-%d " ("time format string (%c)")
              n617 = Format Date/Time String(time format string (%c)=w2407, seconds (now)=w2406) -> (date/time string=w2403:string)  [unwired: 1 in]
              n618 = Format Date/Time String(time format string (%c)=w2407, seconds (now)=w2405) -> (date/time string=w2404:string)  [unwired: 1 in]
              n619 = Format Into String(format string="Select DATE,Production_Count,Station_ID,Stack_holder_ID\nfrom Production_COUNT\nWhere DATE between '%s' and '%s' and Shift_ID='%s'and Stack_holder_ID='%d'\nand Station_ID='%d'" ("string"), w2404, w2403, w2397, 4 ("input 4"), 1 ("input 4")) -> (resulting string=w2400:string)  [unwired: 2 in, 1 out]
              n620 = call "Execute query.vi"("String"=w2400, "connection reference"=w2402) -> ("Table"=w2399:string[][], "connection reference 2"=w2398:T1)  [unwired: 6 in, 2 out]
            }
            frame "2" {
              w2420 = "%Y-%m-%d " ("time format string (%c)")
              n621 = Format Date/Time String(time format string (%c)=w2420, seconds (now)=w2419) -> (date/time string=w2416:string)  [unwired: 1 in]
              n622 = Format Date/Time String(time format string (%c)=w2420, seconds (now)=w2418) -> (date/time string=w2417:string)  [unwired: 1 in]
              n623 = Format Into String(format string="Select DATE,Production_Count,Station_ID,Stack_holder_ID\nfrom Production_COUNT\nWhere DATE between '%s' and '%s' and Shift_ID='%s'and Stack_holder_ID='%d'\nand Station_ID='%d'" ("string"), w2417, w2416, w2410, 4 ("input 4"), 1 ("input 4")) -> (resulting string=w2413:string)  [unwired: 2 in, 1 out]
              n624 = call "Execute query.vi"("String"=w2413, "connection reference"=w2415) -> ("Table"=w2412:string[][], "connection reference 2"=w2411:T1)  [unwired: 6 in, 2 out]
            }
            frame "3" {
              w2433 = "%Y-%m-%d " ("time format string (%c)")
              n625 = Format Date/Time String(time format string (%c)=w2433, seconds (now)=w2432) -> (date/time string=w2429:string)  [unwired: 1 in]
              n626 = Format Date/Time String(time format string (%c)=w2433, seconds (now)=w2431) -> (date/time string=w2430:string)  [unwired: 1 in]
              n627 = Format Into String(format string="Select DATE,Production_Count,Station_ID,Stack_holder_ID\nfrom Production_COUNT\nWhere DATE between '%s' and '%s' and Shift_ID='%s'and Stack_holder_ID='%d'\nand Station_ID='%d'" ("string"), w2430, w2429, w2423, 4 ("input 4"), 1 ("input 4")) -> (resulting string=w2426:string)  [unwired: 2 in, 1 out]
              n628 = call "Execute query.vi"("String"=w2426, "connection reference"=w2428) -> ("Table"=w2425:string[][], "connection reference 2"=w2424:T1)  [unwired: 6 in, 2 out]
            }
          }
        }
        frame "Production" {
          n629 = case shown="\"ALL\"" w2440 {
            selector: w2440 -> [_ _ w2456 w2469 w2482]
            tunnel: w2439 -> [_ w2452 w2465 w2478 w2491]
            tunnel: w2438 -> [_ w2451 w2464 w2477 w2490]
            tunnel: w2437 -> [_ _ _ _ _]
            tunnel: [_ w2445 w2458 w2471 w2484] -> w2436
            tunnel: w2435 -> [w2441 w2448 w2461 w2474 w2487]
            tunnel: [w2441 w2444 w2457 w2470 w2483] -> w2434
            frame "False", Default {
            }
            frame "ALL" {
              w2453 = "%Y-%m-%d " ("time format string (%c)")
              n630 = Format Date/Time String(time format string (%c)=w2453, seconds (now)=w2451) -> (date/time string=w2450:string)  [unwired: 1 in]
              n631 = Format Date/Time String(time format string (%c)=w2453, seconds (now)=w2452) -> (date/time string=w2449:string)  [unwired: 1 in]
              n632 = Format Into String(format string="Select DATE,Production_Count,Station_ID,Stack_holder_ID\nfrom Production_COUNT\nWhere DATE between '%s' and '%s' and Stack_holder_ID='%d'\nand Station_ID='%d'" ("string"), w2450, w2449, 5 ("input 3"), 1 ("input 3")) -> (resulting string=w2446:string)  [unwired: 2 in, 1 out]
              n633 = call "Execute query.vi"("String"=w2446, "connection reference"=w2448) -> ("Table"=w2445:string[][], "connection reference 2"=w2444:T1)  [unwired: 6 in, 2 out]
            }
            frame "1" {
              w2466 = "%Y-%m-%d " ("time format string (%c)")
              n634 = Format Date/Time String(time format string (%c)=w2466, seconds (now)=w2465) -> (date/time string=w2462:string)  [unwired: 1 in]
              n635 = Format Date/Time String(time format string (%c)=w2466, seconds (now)=w2464) -> (date/time string=w2463:string)  [unwired: 1 in]
              n636 = Format Into String(format string="Select DATE,Production_Count,Station_ID,Stack_holder_ID\nfrom Production_COUNT\nWhere DATE between '%s' and '%s' and Shift_ID='%s'and Stack_holder_ID='%d'\nand Station_ID='%d'" ("string"), w2463, w2462, w2456, 5 ("input 4"), 1 ("input 4")) -> (resulting string=w2459:string)  [unwired: 2 in, 1 out]
              n637 = call "Execute query.vi"("String"=w2459, "connection reference"=w2461) -> ("Table"=w2458:string[][], "connection reference 2"=w2457:T1)  [unwired: 6 in, 2 out]
            }
            frame "2" {
              w2479 = "%Y-%m-%d " ("time format string (%c)")
              n638 = Format Date/Time String(time format string (%c)=w2479, seconds (now)=w2478) -> (date/time string=w2475:string)  [unwired: 1 in]
              n639 = Format Date/Time String(time format string (%c)=w2479, seconds (now)=w2477) -> (date/time string=w2476:string)  [unwired: 1 in]
              n640 = Format Into String(format string="Select DATE,Production_Count,Station_ID,Stack_holder_ID\nfrom Production_COUNT\nWhere DATE between '%s' and '%s' and Shift_ID='%s'and Stack_holder_ID='%d'\nand Station_ID='%d'" ("string"), w2476, w2475, w2469, 5 ("input 4"), 1 ("input 4")) -> (resulting string=w2472:string)  [unwired: 2 in, 1 out]
              n641 = call "Execute query.vi"("String"=w2472, "connection reference"=w2474) -> ("Table"=w2471:string[][], "connection reference 2"=w2470:T1)  [unwired: 6 in, 2 out]
            }
            frame "3" {
              w2492 = "%Y-%m-%d " ("time format string (%c)")
              n642 = Format Date/Time String(time format string (%c)=w2492, seconds (now)=w2491) -> (date/time string=w2488:string)  [unwired: 1 in]
              n643 = Format Date/Time String(time format string (%c)=w2492, seconds (now)=w2490) -> (date/time string=w2489:string)  [unwired: 1 in]
              n644 = Format Into String(format string="Select DATE,Production_Count,Station_ID,Stack_holder_ID\nfrom Production_COUNT\nWhere DATE between '%s' and '%s' and Shift_ID='%s'and Stack_holder_ID='%d'\nand Station_ID='%d'" ("string"), w2489, w2488, w2482, 5 ("input 4"), 1 ("input 4")) -> (resulting string=w2485:string)  [unwired: 2 in, 1 out]
              n645 = call "Execute query.vi"("String"=w2485, "connection reference"=w2487) -> ("Table"=w2484:string[][], "connection reference 2"=w2483:T1)  [unwired: 6 in, 2 out]
            }
          }
        }
      }
    }
    frame "ST 6" {
      n646 = case shown="\"ALL\", Default" w2499 {
        tunnel: w2505 -> [w2517 w2618 w2677 w2733 w2792 w2851]
        tunnel: w2504 -> [w2516 w2617 w2676 w2732 w2791 w2850]
        tunnel: w2503 -> [w2515 w2616 w2675 w2731 w2790 w2849]
        tunnel: w2502 -> [w2514 w2615 w2674 w2730 w2789 w2848]
        tunnel: [w2513 w2614 w2673 w2729 w2788 w2847] -> w2496
        tunnel: w2501 -> [w2512 w2613 w2672 w2728 w2787 w2846]
        tunnel: [w2511 w2612 w2671 w2727 w2786 w2845] -> w2500
        tunnel: w2498 -> [w2510 _ _ _ _ _]
        tunnel: w2497 -> [w2509 _ _ _ _ _]
        tunnel: w2495 -> [w2508 _ _ _ _ _]
        tunnel: [w2507 _ _ _ _ _] -> w2494
        tunnel: w2493 -> [w2506 _ _ _ _ _]
        frame "ALL", Default {
          n647 = case shown="\"ALL\", Default" w2517 {
            selector: w2517 -> [_ w2542 w2566 w2590]
            tunnel: w2516 -> [_ _ _ _]
            tunnel: w2515 -> [_ _ _ _]
            tunnel: w2514 -> [_ _ _ _]
            tunnel: [w2520 w2543 w2567 w2591] -> w2513
            tunnel: w2512 -> [w2525 w2548 w2572 w2596]
            tunnel: [w2524 w2547 w2571 w2595] -> w2511
            tunnel: w2510 -> [w2523 w2546 w2570 w2594]
            tunnel: w2509 -> [_ _ _ _]
            tunnel: w2508 -> [w2522 w2545 w2569 w2593]
            tunnel: [w2519 w2541 w2565 w2589] -> w2507
            tunnel: w2506 -> [w2518 w2540 w2564 w2588]
            frame "ALL", Default {
              n648 = for {
                tunnel: w2523 -> [w2535]
                shift-right: [w2537] -> w2524
                shift-left: w2525 -> [w2539]
                tunnel: w2522 -> [w2531] mode=indexing
                shift-right: [w2528] -> w2520
                shift-left: string[][] [] -> [w2530]
                tunnel: [w2526] -> w2519
                tunnel: w2518 -> [w2527]
                n649 = Concatenate Strings("Select DISTINCT PLAN_DATE,PRODUCTION_COUNT,STATION_ID from  ", w2531, " Where year(PLAN_DATE) ='%s' and STATION_ID='%d'\n") -> (w2532:string)
                n650 = Format Into String(format string=w2532, w2535, 6 ("input 3")) -> (resulting string=w2538:string)  [unwired: 2 in, 1 out]
                n651 = call "Execute query.vi"("error in (no error)"=w2527, "String"=w2538, "connection reference"=w2539) -> ("error out"=w2526:errorcluster, "Table"=w2529:string[][], "connection reference 2"=w2537:T1)  [unwired: 5 in, 1 out]
                n652 = Build Array (concatenate)(w2530, w2529) -> (w2528:string[][])
              }
            }
            frame "1" {
              n653 = for {
                tunnel: w2546 -> [w2559]
                shift-right: [w2561] -> w2547
                shift-left: w2548 -> [w2563]
                tunnel: w2545 -> [w2555] mode=indexing
                shift-right: [w2552] -> w2543
                shift-left: string[][] [] -> [w2554]
                tunnel: w2542 -> [w2551]
                tunnel: [w2549] -> w2541
                tunnel: w2540 -> [w2550]
                n654 = Concatenate Strings("Select DISTINCT PLAN_DATE,PRODUCTION_COUNT,STATION_ID from  ", w2555, " Where year(PLAN_DATE) ='%s' and STATION_ID='%d' and  SHIFT='%s'\n") -> (w2556:string)
                n655 = Format Into String(format string=w2556, w2559, 6 ("input 3"), w2551) -> (resulting string=w2562:string)  [unwired: 2 in, 1 out]
                n656 = call "Execute query.vi"("error in (no error)"=w2550, "String"=w2562, "connection reference"=w2563) -> ("error out"=w2549:errorcluster, "Table"=w2553:string[][], "connection reference 2"=w2561:T1)  [unwired: 5 in, 1 out]
                n657 = Build Array (concatenate)(w2554, w2553) -> (w2552:string[][])
              }
            }
            frame "2" {
              n658 = for {
                tunnel: w2570 -> [w2583]
                shift-right: [w2585] -> w2571
                shift-left: w2572 -> [w2587]
                tunnel: w2569 -> [w2579] mode=indexing
                shift-right: [w2576] -> w2567
                shift-left: string[][] [] -> [w2578]
                tunnel: w2566 -> [w2575]
                tunnel: [w2573] -> w2565
                tunnel: w2564 -> [w2574]
                n659 = Concatenate Strings("Select DISTINCT PLAN_DATE,PRODUCTION_COUNT,STATION_ID from  ", w2579, " Where year(PLAN_DATE) ='%s' and STATION_ID='%d' and SHIFT='%s'\n") -> (w2580:string)
                n660 = Format Into String(format string=w2580, w2583, 6 ("input 3"), w2575) -> (resulting string=w2586:string)  [unwired: 2 in, 1 out]
                n661 = call "Execute query.vi"("error in (no error)"=w2574, "String"=w2586, "connection reference"=w2587) -> ("error out"=w2573:errorcluster, "Table"=w2577:string[][], "connection reference 2"=w2585:T1)  [unwired: 5 in, 1 out]
                n662 = Build Array (concatenate)(w2578, w2577) -> (w2576:string[][])
              }
            }
            frame "3" {
              n663 = for {
                tunnel: w2594 -> [w2607]
                shift-right: [w2609] -> w2595
                shift-left: w2596 -> [w2611]
                tunnel: w2593 -> [w2603] mode=indexing
                shift-right: [w2600] -> w2591
                shift-left: string[][] [] -> [w2602]
                tunnel: w2590 -> [w2599]
                tunnel: [w2597] -> w2589
                tunnel: w2588 -> [w2598]
                n664 = Concatenate Strings("Select DISTINCT PLAN_DATE,PRODUCTION_COUNT,STATION_ID from  ", w2603, " Where year(PLAN_DATE) ='%s' and STATION_ID='%d' and  SHIFT='%s'\n") -> (w2604:string)
                n665 = Format Into String(format string=w2604, w2607, 6 ("input 3"), w2599) -> (resulting string=w2610:string)  [unwired: 2 in, 1 out]
                n666 = call "Execute query.vi"("error in (no error)"=w2598, "String"=w2610, "connection reference"=w2611) -> ("error out"=w2597:errorcluster, "Table"=w2601:string[][], "connection reference 2"=w2609:T1)  [unwired: 5 in, 1 out]
                n667 = Build Array (concatenate)(w2602, w2601) -> (w2600:string[][])
              }
            }
          }
        }
        frame "Logistics" {
          n668 = case shown="\"ALL\"" w2618 {
            selector: w2618 -> [_ _ w2634 w2647 w2660]
            tunnel: w2617 -> [_ w2630 w2643 w2656 w2669]
            tunnel: w2616 -> [_ w2629 w2642 w2655 w2668]
            tunnel: w2615 -> [_ _ _ _ _]
            tunnel: [_ w2623 w2636 w2649 w2662] -> w2614
            tunnel: w2613 -> [w2619 w2626 w2639 w2652 w2665]
            tunnel: [w2619 w2622 w2635 w2648 w2661] -> w2612
            frame "False", Default {
            }
            frame "ALL" {
              w2631 = "%Y-%m-%d " ("time format string (%c)")
              n669 = Format Date/Time String(time format string (%c)=w2631, seconds (now)=w2629) -> (date/time string=w2628:string)  [unwired: 1 in]
              n670 = Format Date/Time String(time format string (%c)=w2631, seconds (now)=w2630) -> (date/time string=w2627:string)  [unwired: 1 in]
              n671 = Format Into String(format string="Select DATE,Production_Count,Station_ID,Stack_holder_ID\nfrom Production_COUNT\nWhere DATE between '%s' and '%s' and Stack_holder_ID='%d'\nand Station_ID='%d'" ("string"), w2628, w2627, 2 ("input 3"), 1 ("input 4")) -> (resulting string=w2624:string)  [unwired: 2 in, 1 out]
              n672 = call "Execute query.vi"("String"=w2624, "connection reference"=w2626) -> ("Table"=w2623:string[][], "connection reference 2"=w2622:T1)  [unwired: 6 in, 2 out]
            }
            frame "1" {
              w2644 = "%Y-%m-%d " ("time format string (%c)")
              n673 = Format Date/Time String(time format string (%c)=w2644, seconds (now)=w2643) -> (date/time string=w2640:string)  [unwired: 1 in]
              n674 = Format Date/Time String(time format string (%c)=w2644, seconds (now)=w2642) -> (date/time string=w2641:string)  [unwired: 1 in]
              n675 = Format Into String(format string="Select DATE,Production_Count,Station_ID,Stack_holder_ID\nfrom Production_COUNT\nWhere DATE between '%s' and '%s' and Shift_ID='%s'and Stack_holder_ID='%d'\nand Station_ID='%d'" ("string"), w2641, w2640, w2634, 2 ("input 4"), 1 ("input 4")) -> (resulting string=w2637:string)  [unwired: 2 in, 1 out]
              n676 = call "Execute query.vi"("String"=w2637, "connection reference"=w2639) -> ("Table"=w2636:string[][], "connection reference 2"=w2635:T1)  [unwired: 6 in, 2 out]
            }
            frame "2" {
              w2657 = "%Y-%m-%d " ("time format string (%c)")
              n677 = Format Date/Time String(time format string (%c)=w2657, seconds (now)=w2656) -> (date/time string=w2653:string)  [unwired: 1 in]
              n678 = Format Date/Time String(time format string (%c)=w2657, seconds (now)=w2655) -> (date/time string=w2654:string)  [unwired: 1 in]
              n679 = Format Into String(format string="Select DATE,Production_Count,Station_ID,Stack_holder_ID\nfrom Production_COUNT\nWhere DATE between '%s' and '%s' and Shift_ID='%s'and Stack_holder_ID='%d'\nand Station_ID='%d'" ("string"), w2654, w2653, w2647, 2 ("input 4"), 1 ("input 4")) -> (resulting string=w2650:string)  [unwired: 2 in, 1 out]
              n680 = call "Execute query.vi"("String"=w2650, "connection reference"=w2652) -> ("Table"=w2649:string[][], "connection reference 2"=w2648:T1)  [unwired: 6 in, 2 out]
            }
            frame "3" {
              w2670 = "%Y-%m-%d " ("time format string (%c)")
              n681 = Format Date/Time String(time format string (%c)=w2670, seconds (now)=w2669) -> (date/time string=w2666:string)  [unwired: 1 in]
              n682 = Format Date/Time String(time format string (%c)=w2670, seconds (now)=w2668) -> (date/time string=w2667:string)  [unwired: 1 in]
              n683 = Format Into String(format string="Select DATE,Production_Count,Station_ID,Stack_holder_ID\nfrom Production_COUNT\nWhere DATE between '%s' and '%s' and Shift_ID='%s'and Stack_holder_ID='%d'\nand Station_ID='%d'" ("string"), w2667, w2666, w2660, 2 ("input 4"), 1 ("input 4")) -> (resulting string=w2663:string)  [unwired: 2 in, 1 out]
              n684 = call "Execute query.vi"("String"=w2663, "connection reference"=w2665) -> ("Table"=w2662:string[][], "connection reference 2"=w2661:T1)  [unwired: 6 in, 2 out]
            }
          }
        }
        frame "Gap Leader" {
          n685 = case shown="\"3\"" w2677 {
            selector: w2677 -> [_ _ w2692 w2704 w2716]
            tunnel: w2676 -> [_ w2689 w2701 w2713 w2725]
            tunnel: w2675 -> [_ w2688 w2700 w2712 w2724]
            tunnel: w2674 -> [_ _ _ _ _]
            tunnel: [_ w2682 w2694 w2706 w2718] -> w2673
            tunnel: w2672 -> [w2678 w2685 w2697 w2709 w2721]
            tunnel: [w2678 w2681 w2693 w2705 w2717] -> w2671
            frame "False", Default {
            }
            frame "ALL" {
              w2690 = "%Y-%m-%d " ("time format string (%c)")
              n686 = Format Date/Time String(time format string (%c)=w2690, seconds (now)=w2688) -> (date/time string=w2687:string)  [unwired: 1 in]
              n687 = Format Date/Time String(time format string (%c)=w2690, seconds (now)=w2689) -> (date/time string=w2686:string)  [unwired: 1 in]
              n688 = Format Into String(format string="Select DATE,Production_Count,Station_ID,Stack_holder_ID\nfrom Production_COUNT\nWhere DATE between '%s' and '%s' and Stack_holder_ID='%d'\nand Station_ID='%d'" ("string"), w2687, w2686, 1 ("input 3"), 1 ("input 3")) -> (resulting string=w2683:string)  [unwired: 2 in, 1 out]
              n689 = call "Execute query.vi"("String"=w2683, "connection reference"=w2685) -> ("Table"=w2682:string[][], "connection reference 2"=w2681:T1)  [unwired: 6 in, 2 out]
            }
            frame "1" {
              w2691 = 1 ("input 4")
              w2702 = "%Y-%m-%d " ("time format string (%c)")
              n690 = Format Date/Time String(time format string (%c)=w2702, seconds (now)=w2701) -> (date/time string=w2698:string)  [unwired: 1 in]
              n691 = Format Date/Time String(time format string (%c)=w2702, seconds (now)=w2700) -> (date/time string=w2699:string)  [unwired: 1 in]
              n692 = Format Into String(format string="Select DATE,Production_Count,Station_ID,Stack_holder_ID\nfrom Production_COUNT\nWhere DATE between '%s' and '%s' and Shift_ID='%s'and Stack_holder_ID='%d'\nand Station_ID='%d'" ("string"), w2699, w2698, w2692, w2691, w2691) -> (resulting string=w2695:string)  [unwired: 2 in, 1 out]
              n693 = call "Execute query.vi"("String"=w2695, "connection reference"=w2697) -> ("Table"=w2694:string[][], "connection reference 2"=w2693:T1)  [unwired: 6 in, 2 out]
            }
            frame "2" {
              w2703 = 1 ("input 4")
              w2714 = "%Y-%m-%d " ("time format string (%c)")
              n694 = Format Date/Time String(time format string (%c)=w2714, seconds (now)=w2713) -> (date/time string=w2710:string)  [unwired: 1 in]
              n695 = Format Date/Time String(time format string (%c)=w2714, seconds (now)=w2712) -> (date/time string=w2711:string)  [unwired: 1 in]
              n696 = Format Into String(format string="Select DATE,Production_Count,Station_ID,Stack_holder_ID\nfrom Production_COUNT\nWhere DATE between '%s' and '%s' and Shift_ID='%s'and Stack_holder_ID='%d'\nand Station_ID='%d'" ("string"), w2711, w2710, w2704, w2703, w2703) -> (resulting string=w2707:string)  [unwired: 2 in, 1 out]
              n697 = call "Execute query.vi"("String"=w2707, "connection reference"=w2709) -> ("Table"=w2706:string[][], "connection reference 2"=w2705:T1)  [unwired: 6 in, 2 out]
            }
            frame "3" {
              w2715 = 1 ("input 4")
              w2726 = "%Y-%m-%d " ("time format string (%c)")
              n698 = Format Date/Time String(time format string (%c)=w2726, seconds (now)=w2725) -> (date/time string=w2722:string)  [unwired: 1 in]
              n699 = Format Date/Time String(time format string (%c)=w2726, seconds (now)=w2724) -> (date/time string=w2723:string)  [unwired: 1 in]
              n700 = Format Into String(format string="Select DATE,Production_Count,Station_ID,Stack_holder_ID\nfrom Production_COUNT\nWhere DATE between '%s' and '%s' and Shift_ID='%s'and Stack_holder_ID='%d'\nand Station_ID='%d'" ("string"), w2723, w2722, w2716, w2715, w2715) -> (resulting string=w2719:string)  [unwired: 2 in, 1 out]
              n701 = call "Execute query.vi"("String"=w2719, "connection reference"=w2721) -> ("Table"=w2718:string[][], "connection reference 2"=w2717:T1)  [unwired: 6 in, 2 out]
            }
          }
        }
        frame "Maintenance" {
          n702 = case shown="\"ALL\"" w2733 {
            selector: w2733 -> [_ _ w2749 w2762 w2775]
            tunnel: w2732 -> [_ w2745 w2758 w2771 w2784]
            tunnel: w2731 -> [_ w2744 w2757 w2770 w2783]
            tunnel: w2730 -> [_ _ _ _ _]
            tunnel: [_ w2738 w2751 w2764 w2777] -> w2729
            tunnel: w2728 -> [w2734 w2741 w2754 w2767 w2780]
            tunnel: [w2734 w2737 w2750 w2763 w2776] -> w2727
            frame "False", Default {
            }
            frame "ALL" {
              w2746 = "%Y-%m-%d " ("time format string (%c)")
              n703 = Format Date/Time String(time format string (%c)=w2746, seconds (now)=w2744) -> (date/time string=w2743:string)  [unwired: 1 in]
              n704 = Format Date/Time String(time format string (%c)=w2746, seconds (now)=w2745) -> (date/time string=w2742:string)  [unwired: 1 in]
              n705 = Format Into String(format string="Select DATE,Production_Count,Station_ID,Stack_holder_ID\nfrom Production_COUNT\nWhere DATE between '%s' and '%s' and Stack_holder_ID='%d'\nand Station_ID='%d'" ("string"), w2743, w2742, 3 ("input 3"), 1 ("input 4")) -> (resulting string=w2739:string)  [unwired: 2 in, 1 out]
              n706 = call "Execute query.vi"("String"=w2739, "connection reference"=w2741) -> ("Table"=w2738:string[][], "connection reference 2"=w2737:T1)  [unwired: 6 in, 2 out]
            }
            frame "1" {
              w2759 = "%Y-%m-%d " ("time format string (%c)")
              n707 = Format Date/Time String(time format string (%c)=w2759, seconds (now)=w2758) -> (date/time string=w2755:string)  [unwired: 1 in]
              n708 = Format Date/Time String(time format string (%c)=w2759, seconds (now)=w2757) -> (date/time string=w2756:string)  [unwired: 1 in]
              n709 = Format Into String(format string="Select DATE,Production_Count,Station_ID,Stack_holder_ID\nfrom Production_COUNT\nWhere DATE between '%s' and '%s' and Shift_ID='%s'and Stack_holder_ID='%d'\nand Station_ID='%d'" ("string"), w2756, w2755, w2749, 3 ("input 4"), 1 ("input 5")) -> (resulting string=w2752:string)  [unwired: 2 in, 1 out]
              n710 = call "Execute query.vi"("String"=w2752, "connection reference"=w2754) -> ("Table"=w2751:string[][], "connection reference 2"=w2750:T1)  [unwired: 6 in, 2 out]
            }
            frame "2" {
              w2772 = "%Y-%m-%d " ("time format string (%c)")
              n711 = Format Date/Time String(time format string (%c)=w2772, seconds (now)=w2771) -> (date/time string=w2768:string)  [unwired: 1 in]
              n712 = Format Date/Time String(time format string (%c)=w2772, seconds (now)=w2770) -> (date/time string=w2769:string)  [unwired: 1 in]
              n713 = Format Into String(format string="Select DATE,Production_Count,Station_ID,Stack_holder_ID\nfrom Production_COUNT\nWhere DATE between '%s' and '%s' and Shift_ID='%s'and Stack_holder_ID='%d'\nand Station_ID='%d'" ("string"), w2769, w2768, w2762, 3 ("input 4"), 1 ("input 5")) -> (resulting string=w2765:string)  [unwired: 2 in, 1 out]
              n714 = call "Execute query.vi"("String"=w2765, "connection reference"=w2767) -> ("Table"=w2764:string[][], "connection reference 2"=w2763:T1)  [unwired: 6 in, 2 out]
            }
            frame "3" {
              w2785 = "%Y-%m-%d " ("time format string (%c)")
              n715 = Format Date/Time String(time format string (%c)=w2785, seconds (now)=w2784) -> (date/time string=w2781:string)  [unwired: 1 in]
              n716 = Format Date/Time String(time format string (%c)=w2785, seconds (now)=w2783) -> (date/time string=w2782:string)  [unwired: 1 in]
              n717 = Format Into String(format string="Select DATE,Production_Count,Station_ID,Stack_holder_ID\nfrom Production_COUNT\nWhere DATE between '%s' and '%s' and Shift_ID='%s'and Stack_holder_ID='%d'\nand Station_ID='%d'" ("string"), w2782, w2781, w2775, 3 ("input 4"), 1 ("input 5")) -> (resulting string=w2778:string)  [unwired: 2 in, 1 out]
              n718 = call "Execute query.vi"("String"=w2778, "connection reference"=w2780) -> ("Table"=w2777:string[][], "connection reference 2"=w2776:T1)  [unwired: 6 in, 2 out]
            }
          }
        }
        frame "Quality" {
          n719 = case shown="\"ALL\"" w2792 {
            selector: w2792 -> [_ _ w2808 w2821 w2834]
            tunnel: w2791 -> [_ w2804 w2817 w2830 w2843]
            tunnel: w2790 -> [_ w2803 w2816 w2829 w2842]
            tunnel: w2789 -> [_ _ _ _ _]
            tunnel: [_ w2797 w2810 w2823 w2836] -> w2788
            tunnel: w2787 -> [w2793 w2800 w2813 w2826 w2839]
            tunnel: [w2793 w2796 w2809 w2822 w2835] -> w2786
            frame "False", Default {
            }
            frame "ALL" {
              w2805 = "%Y-%m-%d " ("time format string (%c)")
              n720 = Format Date/Time String(time format string (%c)=w2805, seconds (now)=w2803) -> (date/time string=w2802:string)  [unwired: 1 in]
              n721 = Format Date/Time String(time format string (%c)=w2805, seconds (now)=w2804) -> (date/time string=w2801:string)  [unwired: 1 in]
              n722 = Format Into String(format string="Select DATE,Production_Count,Station_ID,Stack_holder_ID\nfrom Production_COUNT\nWhere DATE between '%s' and '%s' and Stack_holder_ID='%d'\nand Station_ID='%d'" ("string"), w2802, w2801, 4 ("input 3"), 1 ("input 3")) -> (resulting string=w2798:string)  [unwired: 2 in, 1 out]
              n723 = call "Execute query.vi"("String"=w2798, "connection reference"=w2800) -> ("Table"=w2797:string[][], "connection reference 2"=w2796:T1)  [unwired: 6 in, 2 out]
            }
            frame "1" {
              w2818 = "%Y-%m-%d " ("time format string (%c)")
              n724 = Format Date/Time String(time format string (%c)=w2818, seconds (now)=w2817) -> (date/time string=w2814:string)  [unwired: 1 in]
              n725 = Format Date/Time String(time format string (%c)=w2818, seconds (now)=w2816) -> (date/time string=w2815:string)  [unwired: 1 in]
              n726 = Format Into String(format string="Select DATE,Production_Count,Station_ID,Stack_holder_ID\nfrom Production_COUNT\nWhere DATE between '%s' and '%s' and Shift_ID='%s'and Stack_holder_ID='%d'\nand Station_ID='%d'" ("string"), w2815, w2814, w2808, 4 ("input 4"), 1 ("input 4")) -> (resulting string=w2811:string)  [unwired: 2 in, 1 out]
              n727 = call "Execute query.vi"("String"=w2811, "connection reference"=w2813) -> ("Table"=w2810:string[][], "connection reference 2"=w2809:T1)  [unwired: 6 in, 2 out]
            }
            frame "2" {
              w2831 = "%Y-%m-%d " ("time format string (%c)")
              n728 = Format Date/Time String(time format string (%c)=w2831, seconds (now)=w2830) -> (date/time string=w2827:string)  [unwired: 1 in]
              n729 = Format Date/Time String(time format string (%c)=w2831, seconds (now)=w2829) -> (date/time string=w2828:string)  [unwired: 1 in]
              n730 = Format Into String(format string="Select DATE,Production_Count,Station_ID,Stack_holder_ID\nfrom Production_COUNT\nWhere DATE between '%s' and '%s' and Shift_ID='%s'and Stack_holder_ID='%d'\nand Station_ID='%d'" ("string"), w2828, w2827, w2821, 4 ("input 4"), 1 ("input 4")) -> (resulting string=w2824:string)  [unwired: 2 in, 1 out]
              n731 = call "Execute query.vi"("String"=w2824, "connection reference"=w2826) -> ("Table"=w2823:string[][], "connection reference 2"=w2822:T1)  [unwired: 6 in, 2 out]
            }
            frame "3" {
              w2844 = "%Y-%m-%d " ("time format string (%c)")
              n732 = Format Date/Time String(time format string (%c)=w2844, seconds (now)=w2843) -> (date/time string=w2840:string)  [unwired: 1 in]
              n733 = Format Date/Time String(time format string (%c)=w2844, seconds (now)=w2842) -> (date/time string=w2841:string)  [unwired: 1 in]
              n734 = Format Into String(format string="Select DATE,Production_Count,Station_ID,Stack_holder_ID\nfrom Production_COUNT\nWhere DATE between '%s' and '%s' and Shift_ID='%s'and Stack_holder_ID='%d'\nand Station_ID='%d'" ("string"), w2841, w2840, w2834, 4 ("input 4"), 1 ("input 4")) -> (resulting string=w2837:string)  [unwired: 2 in, 1 out]
              n735 = call "Execute query.vi"("String"=w2837, "connection reference"=w2839) -> ("Table"=w2836:string[][], "connection reference 2"=w2835:T1)  [unwired: 6 in, 2 out]
            }
          }
        }
        frame "Production" {
          n736 = case shown="\"ALL\"" w2851 {
            selector: w2851 -> [_ _ w2867 w2880 w2893]
            tunnel: w2850 -> [_ w2863 w2876 w2889 w2902]
            tunnel: w2849 -> [_ w2862 w2875 w2888 w2901]
            tunnel: w2848 -> [_ _ _ _ _]
            tunnel: [_ w2856 w2869 w2882 w2895] -> w2847
            tunnel: w2846 -> [w2852 w2859 w2872 w2885 w2898]
            tunnel: [w2852 w2855 w2868 w2881 w2894] -> w2845
            frame "False", Default {
            }
            frame "ALL" {
              w2864 = "%Y-%m-%d " ("time format string (%c)")
              n737 = Format Date/Time String(time format string (%c)=w2864, seconds (now)=w2862) -> (date/time string=w2861:string)  [unwired: 1 in]
              n738 = Format Date/Time String(time format string (%c)=w2864, seconds (now)=w2863) -> (date/time string=w2860:string)  [unwired: 1 in]
              n739 = Format Into String(format string="Select DATE,Production_Count,Station_ID,Stack_holder_ID\nfrom Production_COUNT\nWhere DATE between '%s' and '%s' and Stack_holder_ID='%d'\nand Station_ID='%d'" ("string"), w2861, w2860, 5 ("input 3"), 1 ("input 3")) -> (resulting string=w2857:string)  [unwired: 2 in, 1 out]
              n740 = call "Execute query.vi"("String"=w2857, "connection reference"=w2859) -> ("Table"=w2856:string[][], "connection reference 2"=w2855:T1)  [unwired: 6 in, 2 out]
            }
            frame "1" {
              w2877 = "%Y-%m-%d " ("time format string (%c)")
              n741 = Format Date/Time String(time format string (%c)=w2877, seconds (now)=w2876) -> (date/time string=w2873:string)  [unwired: 1 in]
              n742 = Format Date/Time String(time format string (%c)=w2877, seconds (now)=w2875) -> (date/time string=w2874:string)  [unwired: 1 in]
              n743 = Format Into String(format string="Select DATE,Production_Count,Station_ID,Stack_holder_ID\nfrom Production_COUNT\nWhere DATE between '%s' and '%s' and Shift_ID='%s'and Stack_holder_ID='%d'\nand Station_ID='%d'" ("string"), w2874, w2873, w2867, 5 ("input 4"), 1 ("input 4")) -> (resulting string=w2870:string)  [unwired: 2 in, 1 out]
              n744 = call "Execute query.vi"("String"=w2870, "connection reference"=w2872) -> ("Table"=w2869:string[][], "connection reference 2"=w2868:T1)  [unwired: 6 in, 2 out]
            }
            frame "2" {
              w2890 = "%Y-%m-%d " ("time format string (%c)")
              n745 = Format Date/Time String(time format string (%c)=w2890, seconds (now)=w2889) -> (date/time string=w2886:string)  [unwired: 1 in]
              n746 = Format Date/Time String(time format string (%c)=w2890, seconds (now)=w2888) -> (date/time string=w2887:string)  [unwired: 1 in]
              n747 = Format Into String(format string="Select DATE,Production_Count,Station_ID,Stack_holder_ID\nfrom Production_COUNT\nWhere DATE between '%s' and '%s' and Shift_ID='%s'and Stack_holder_ID='%d'\nand Station_ID='%d'" ("string"), w2887, w2886, w2880, 5 ("input 4"), 1 ("input 4")) -> (resulting string=w2883:string)  [unwired: 2 in, 1 out]
              n748 = call "Execute query.vi"("String"=w2883, "connection reference"=w2885) -> ("Table"=w2882:string[][], "connection reference 2"=w2881:T1)  [unwired: 6 in, 2 out]
            }
            frame "3" {
              w2903 = "%Y-%m-%d " ("time format string (%c)")
              n749 = Format Date/Time String(time format string (%c)=w2903, seconds (now)=w2902) -> (date/time string=w2899:string)  [unwired: 1 in]
              n750 = Format Date/Time String(time format string (%c)=w2903, seconds (now)=w2901) -> (date/time string=w2900:string)  [unwired: 1 in]
              n751 = Format Into String(format string="Select DATE,Production_Count,Station_ID,Stack_holder_ID\nfrom Production_COUNT\nWhere DATE between '%s' and '%s' and Shift_ID='%s'and Stack_holder_ID='%d'\nand Station_ID='%d'" ("string"), w2900, w2899, w2893, 5 ("input 4"), 1 ("input 4")) -> (resulting string=w2896:string)  [unwired: 2 in, 1 out]
              n752 = call "Execute query.vi"("String"=w2896, "connection reference"=w2898) -> ("Table"=w2895:string[][], "connection reference 2"=w2894:T1)  [unwired: 6 in, 2 out]
            }
          }
        }
      }
    }
  }
  "Table" <- w7
  "Refnum out" <- w20
  "error out" <- w2
  n753 = Index Array(array=w7, index (col)=0 ("disabled index (col)")) -> (element=w17:string[])  [unwired: 1 in]
  n754 = call "Search_1d_array_element.vi"("Count in"=string[] [] ("Count"), "BD Date"=w17, "Elements Found in"=string[] [] ("Elements Found")) -> ("Count out"=w14:string[], "Elements Found out"=w15:string[])  [unwired: 4 in, 1 out]
  "Elements Found out" <- w15
  "PROD COUNT TEST" <- w14
  n755 = call "Production_count_sum.vi"("Table 3"=w7, "date count"=w14, "Founded dates"=w15) -> ("sum"=→"sum":i32[], "Array 3"=→"Array 3":string[][])  [unwired: 7 in]
